vi "Position_TOTAL_R24_cleaned up front.vi"(5 "Distance Between \nCameras  (*unit)":sgl=2.3) -> (12 "dX, dY\nLeft Cam":cluster{"X":sgl[], "Y":sgl[]}={"X"=[-1.0065897, 0.099401906, 1.1628555, 2.2500029, 0.0], "Y"=[10.716516, 10.801518, 10.883252, 10.9668045, 0.0]}, 13 "Position Valid":bool=TRUE, 14 "Left Camera Real Coordinates":cluster{"X":sgl, "Y":sgl}={"X"=10.842023, "Y"=1.3735824}, 16 "dX, dY\nRight Cam":cluster{"X":sgl[], "Y":sgl[]}={"X"=[-2.8840373, -1.7780458, -0.7145921, 0.3725553, -1.8774476], "Y"=[9.387911, 9.472914, 9.554648, 9.638201, -1.3286046]}, 18 "Robot Coordinates":cluster{"X":sgl, "Y":sgl}={"X"=10.17772, "Y"=2.3123062}, 19 "Orietnation\n(current)":sgl=-30.94054 format="%#_13g")   [LabVIEW 2015]
uses:
  <vilib>/Analysis/coordinate.llb/2D Cartesian Coordinate Rotation (Array).vi
  <vilib>/myRIO/Common/Instrument Driver Framework/myRIO v1.0/DIO/vis/myRIO v1.0 Close DIO.vi
  <vilib>/myRIO/Common/Instrument Driver Framework/myRIO v1.0/DIO/vis/myRIO v1.0 Unreserve DIO.vi
  <vilib>/myRIO/Common/Instrument Driver Framework/myRIO v1.0/DIO/vis/myRIO v1.0 Build MUX Configuration DIO.vi
  <vilib>/myRIO/Common/Instrument Driver Framework/myRIO v1.0/Resource Manager/vis/myRIO v1.0 Unreserve Channel List.vi
  <vilib>/myRIO/Common/Instrument Driver Framework/myRIO v1.0/Resource Manager/vis/myRIO v1.0 Create Configuration List.vi
  <vilib>/myRIO/Common/Instrument Driver Framework/myRIO v1.0/Resource Manager/vis/myRIO v1.0 Unreserve Channel.vi
  <vilib>/myRIO/Common/Instrument Driver Framework/myRIO v1.0/Resource Manager/vis/myRIO v1.0 Build Mutex Name.vi
  <vilib>/Instr/_visa.llb/VISA Configure Serial Port (Instr).vi
  <vilib>/myRIO/Common/Instrument Driver Framework/myRIO v1.0/DIO/vis/myRIO v1.0 Shutdown DIO.vi
  <vilib>/Utility/error.llb/Error Cluster From Error Code.vi
  <vilib>/myRIO/Common/Instrument Driver Framework/myRIO v1.0/Resource Manager/vis/myRIO v1.0 Configure IO.vi
  <vilib>/myRIO/Common/Instrument Driver Framework/Utilities/vis/Configuration Manager.vi
  <vilib>/myRIO/Common/Instrument Driver Framework/Utilities/vis/IO Manager.vi
  <vilib>/myRIO/Common/Instrument Driver Framework/myRIO v1.0/myRIO v1.0 Close.vi
  <vilib>/Analysis/NI_AALPro.lvlib
  <vilib>/myRIO/Instrument Drivers/Onboard IO/DIO/DIO.lvlib
panel:
  in  "Tab Control 2":T1(tab)
  out "Beacon Coordinates - Right Image":T2={"Beacon Position - X px"=[88.975365, 121.85722, 157.60713, 192.74931, 229.82234], "Beacon Position - Y px"=[106.21975, 102.49595, 103.61968, 103.22959, 103.920715]}
  out "Beacon Coordinates - Left Image":T2={"Beacon Position - X px"=[96.57839, 127.0317, 159.93825, 190.94315, 221.86247], "Beacon Position - Y px"=[111.67795, 107.306076, 106.92789, 105.73433, 104.09002]}
  in  "Image Width (px)":sgl=320.0
  in  "Image Height (px)":sgl=240.0
  in  "Cam AOV Horizontal (deg)":sgl=58.0
  in  "Cam AOV Vertical (deg)":sgl=45.0
  out "Angle to Pixel Ratios":T3={"Angle to Pixel\nRatio - Horizontal"=0.18125, "Angle to Pixel\nRatio - Vertical"=0.1875} {"Angle to Pixel\nRatio - Vertical" format="%#_13g"; "Angle to Pixel\nRatio - Horizontal" format="%#_13g"}
  in  "Num of Beacons (Total)":i8=5
  out "Left Data\nInput Flag\n- Internal":bool
  out "Right Data\nInput Flag\n- Internal":bool
  out "This Servo \nAngle - Left":sgl=52.96875
  in  "Valid Angles - L":bool[](array[boolean])=[TRUE, TRUE, TRUE, TRUE, TRUE]
  in  "Valid Angles -R":bool[](array[boolean])=[TRUE, TRUE, TRUE, TRUE, TRUE]
  in  "Beacon Angles - L":sgl[](array[numeric])=[64.19745, 58.642975, 52.682835, 47.05908, 41.446476]
  in  "Beacon Angles -R":sgl[](array[numeric])=[71.43643, 65.46979, 58.9926, 52.62266, 45.904842]
  out "This Servo \nAngle - Right":sgl=58.76953
  in  "Position Calc\nReady":bool=TRUE
  out "Array":sgl[](array[numeric])=[9.555056, 8.575206, 8.036942, 7.810829, 6.6351933]
  out "Array 2":sgl[](array[numeric])=[5.5039287, 6.210328, 7.1312, 8.266513, 8.73579]
  out "Array 3":sgl[](array[numeric])=[3.2039287, 3.9103284, 4.8311996, 5.9665127, 6.4357905]
  in  "stop":bool
  in  "Current Servo Position\n- Left":u16
  in  "Current Servo Position\n- Right":u16
  in  "Servo Algorithm\nCycle Time(ms)":i32=25
  in  "Move Servo\nThreshold (deg)":sgl=2.0 format="%#_13g"
  in  "SERVO ENABLE":bool=TRUE
  in  "Max Write\nTx Attempts":u8=3
  in  "Max Read\nTx Attempts":u8=3
  in  "close comms":bool
  in  "Servo Comm\nLoop Time (ms)":i32=20
  out "dT - Comm Loop":u32=21
  in  "Left Servo\nID":string="\u0000"
  in  "Servo Comm\nWait Time - (ms)":i32
  in  "Right Servo\nID":string="\u0001"
  in  "Search Step Size\n(deg)":sgl=15.0 format="%#_13g"
  out "Last Orientation":sgl=-35.285717
  out "Last Position":cluster{"X":sgl, "Y":sgl}={"X"=10.147585, "Y"=2.64441}
  in  "Compliance Slope":u8=128
  in  "Search Step Size":u16=50
  in  "Mounting Offset - Left":sgl=-45.0
  in  "Minimum Delta \nServo Threshold":i16=3
  in  "Maximum Move \nServo Threshold":i16=300
  in  "Wait Tick Threshold":i32=10
  in  "Min Num Frames\nper Search":i32=5
  in  "Middle Beacon\nCoordinates":cluster{"X":sgl, "Y":sgl}={"X"=0.0, "Y"=2.5}
  in  "Max Recovery\nSearch Attempts":u16=3
  in  "Max Recovery Count\n(Recovery Search)":u16=20
  in  "Mounting Offset - Right":sgl=45.0
  in  "Tracking Timeout\nThreshold":i32=10
  in  "Timeout to \nEnable Reactive Predict":u16=5
  out "Beacon Scales - Right":sgl[](array[numeric])=[50.81787, 54.150085, 54.01553, 51.723366, 54.605507]
  out "Beacon Scales - Left":sgl[](array[numeric])=[46.59789, 48.180458, 47.842606, 46.504417, 45.297752]
  in  "Recovery Parallel\nSearch Offset":u16=50
  in  "Max # Pan Moves":u16=20
  in  "Current Angle\n - Right (internal)":sgl=58.76953
  in  "Current Angle\n - Left (internal)":sgl=52.96875
  in  "Servo Goal Position\n - Left":u16=232
  in  "Servo Goal Position\n - Right":u16=563
  out "Move Servo - R":bool
  out "Move Servo - L":bool
  out "Current L (10bit)":u16=232
  out "Servo Moving - L":bool
  out "Servo Moving - R":bool
  out "Current R (10bit)":u16=559
  out "deltaMoveServo\n- L":i16
  out "Move Respond - L":bool
  out "Move Respond - R":bool
  out "deltaMoveServo\n- R":i16
  out "Current Main State - Left":T4(ring)=enum."Tracking"
  in  "Initial Main State - Left":T4(ring)
  in  "Image Lock - Left":bool=TRUE
  in  "Track Angle Valid - Left":bool=TRUE
  out "New Data  Flag\nLeft Servo":bool
  in  "Tracking Angle - Left":sgl=52.933372
  in  "Search Direction - in - L":bool
  out "Frames Processed\nCount - in -L":i32
  out "Recovery Mode Count - in Left":u16
  in  "Image Lock - Right":bool
  out "Recovery Search\nmove Count - in - L":u16
  out "Recovery Search\nAttempt Count - in - L":u16
  out "Current Move Delta - L":u16
  out "Next Main State - Left":T4(ring)=enum."Tracking"
  in  "Recovery Search\nDirection - L":bool=TRUE
  out "Last Track Angle - L":sgl=52.96875
  in  "Initial Main State- Right":T4(ring)
  out "Current Main State - Right":T4(ring)=enum."Tracking"
  in  "Track Angle Valid  - Right":bool
  out "New Data  Flag\nRight Servo":bool
  in  "Tracking Angle - Right":sgl=58.953144
  out "Recovery Search\nAttempt Count - Right":u16
  out "Recovery Search\nmove Count - Right":u16
  out "Frames Processed\nCount - in Right":i32
  out "Recovery Mode Count in Right":i32
  in  "Recovery Search\nDirection - R":bool
  out "Next Main State - Right":T4(ring)=enum."Tracking"
  in  "Search Direction - in - Right":bool=TRUE
  out "Tracking Timeout\nCount - L":i32
  out "Tracking Timeout\nCount - R":i32
  out "Current Tracking State - Left":enum16{"Track", "Reactive Predict", ""}(ring)
  in  "Initial Tracking State - Left":enum16{"Track", "Reactive Predict", ""}(ring)
  out "Next Tracking State - Left":enum16{"Track", "Reactive Predict", ""}(ring)
  in  "Initial Tracking State - Right":enum16{"Track", "Reactive Predict", ""}(ring)
  out "Current Tracking State - Right 2":enum16{"Track", "Reactive Predict", ""}(ring)
  out "Next Tracking State - Right":enum16{"Track", "Reactive Predict", ""}(ring)
  in  "Initial Recovery State - L":enum16{"Generic Sweep", "Recovery Search"}(ring)=enum."Recovery Search"
  in  "Initial Recovery State  - Right":enum16{"Generic Sweep", "Recovery Search"}(ring)=enum."Recovery Search"
  out "Current Recovery State - Right":enum16{"Generic Sweep", "Recovery Search"}(ring)=enum."Recovery Search"
  out "Next Recovery State - Right":enum16{"Generic Sweep", "Recovery Search"}(ring)=enum."Recovery Search"
  out "Next Recovery State - Left":enum16{"Generic Sweep", "Recovery Search"}(ring)=enum."Recovery Search"
  out "Current Recovery State -L":enum16{"Generic Sweep", "Recovery Search"}(ring)=enum."Recovery Search"
  out "Current Move Delta - R":u16
  in  "Real Beacon\n - Coordinates":cluster{"X":dbl[], "Y":dbl[]}={"X"=[0.0, 0.0, 0.0, 0.0, 0.0, 0.0], "Y"=[0.5, 1.5, 2.5, 3.5, 4.5, 0.0]}
  out "LOCAL\nBeacon Coordinates\nRelative to Robot":cluster{"dX_beacon":sgl[], "dY_beacon":sgl[]}={"dX_beacon"=[5.5039287, 6.210328, 7.1312, 8.266513, 8.73579], "dY_beacon"=[9.555056, 8.575206, 8.036942, 7.810829, 6.6351933]}
  out "Local Coordinates - Calculated":cluster{sgl[], sgl[]}(graph)={[5.5039287, 6.210328, 7.1312, 8.266513, 8.73579], [9.555056, 8.575206, 8.036942, 7.810829, 6.6351933]}
  out "Distance to LBF":sgl[](array[numeric])=[0.024284193, 0.015691843, 0.008273765, 0.028971607, 0.03291407]
  out "Right Camera Real Coordinate":cluster{"X":sgl, "Y":sgl}={"X"=9.513418, "Y"=3.25103}
  out "Post Filtering\n- Valid Beacons":bool[](array[boolean])=[TRUE, TRUE, TRUE, TRUE, FALSE]
  in  "Distance\nBetween Beacons":sgl=1.0 format="%#_13g"
  in  "Distance\nBetween Beacons \n- Tolerance":sgl=0.5 format="%#_13g"
  out "All Object Coordinates \n- Local":cluster{"X":sgl[], "Y":sgl[]}={"X"=[2.3, 5.368779, 6.320682, 7.235974, 8.171657, 0.0], "Y"=[0.0, 9.329155, 8.759661, 8.21207, 7.6522775, 0.0]}
  out "Local Coordinates - Normalized":cluster{sgl[], dbl[]}(graph)={[2.3, 5.368779, 6.320682, 7.235974, 8.171657, 0.0], [0.0, 9.329154968261719, 8.759660720825195, 8.21207046508789, 7.65227746963501, 0.0]}
  out "All Object Coordinates \n- Local - Rotated":cluster{"X":sgl[], "Y":sgl[]}={"X"=[1.8774476, -1.0065897, 0.099401906, 1.1628555, 2.2500029, 0.0], "Y"=[1.3286046, 10.716516, 10.801518, 10.883252, 10.9668045, 0.0]}
  out "Local Coordinates - Rotated":cluster{dbl[], dbl[]}(graph)={[1.8774476489648846, -1.0065896210507148, 0.09940190570174412, 1.1628555490135675, 2.250002943734801, 0.0], [1.3286045709883498, 10.716515276262749, 10.801518262128845, 10.883252530212562, 10.966804865321656, 0.0]}
  out "Current Cam State - R":T5(ring)=enum."Normal - 5"
  out "Current Cam State - L":T5(ring)=enum."Normal - 5"
  out "Right_Flag 2":bool
  out "Beacons Found\n- Right (Bool Array)":bool[](array[boolean])=[TRUE, TRUE, TRUE, TRUE, TRUE]
  out "RIGHT Beacon Position - Y px (IN)":sgl[](array[numeric])=[106.21975, 102.49595, 103.61968, 103.22959, 103.920715]
  out "RIGHT Beacon Coord - X px (IN)":sgl[](array[numeric])=[88.975365, 121.85722, 157.60713, 192.74931, 229.82234]
  out "Left_Flag 2":bool
  out "Beacons Found\n- Left (Bool Array) 2":bool[](array[boolean])=[TRUE, TRUE, TRUE, TRUE, TRUE]
  out "LEFT Beacon Coord - X px (IN) 2":sgl[](array[numeric])=[96.57839, 127.0317, 159.93825, 190.94315, 221.86247]
  out "LEFT Beacon Position - Y px (IN) 2":sgl[](array[numeric])=[111.67795, 107.306076, 106.92789, 105.73433, 104.09002]
  in  "Fetch Input\n(mSec)":u32=20 caption="Update Camera Input\n(mSec)"
  in  "Max Std Dev (5)":sgl=0.1 format="%#_13g"
  out "Position \nLock Status":bool=TRUE
  out "Real Position in Course 2":cluster{"X":dbl[], "Y":dbl[]}(graph)={"X"=[10.147584990557128], "Y"=[2.644409845240164]}
  out "Robot Coordinates - Avgd":cluster{"X":sgl, "Y":sgl}={"X"=10.147585, "Y"=2.64441}
  in  "Max Std Dev (4)":sgl=0.1 format="%#_13g"
  in  "Max Std Dev (3)":sgl=0.2 format="%#_13g"
  in  "New Position\nWeight (X coord)":sgl=0.8 format="%#_13g"
  in  "Max X (arena)":sgl=35.0
  in  "Max Y (arena)":sgl=15.0
  in  "History Size":u8=15
  out "Orientation Avgd":sgl=-35.285717
  in  "New Position \nThreshold":sgl=2.0
  out "Robot Coordinates\nHistory":cluster{sgl, sgl}[](array[cluster])=[{10.147585, 2.64441}, {10.056327, 2.8351064}, {10.020484, 2.7815769}, {10.034186, 2.7172103}, {0.0, 0.0}, {10.036168, 2.7859242}, {9.938812, 2.8961887}, {10.1160965, 2.6632404}, {10.016709, 2.7454932}, {10.037537, 2.8544023}, {10.017025, 2.7817721}, {9.997087, 2.8064857}, {10.065648, 2.6537364}, {10.084976, 2.6750228}, {10.082739, 2.688601}]
  out "Orientation\nHistory":sgl[](array[numeric])=[-35.285717, -36.86449, -36.153664, -35.44657, 0.0, -37.6105, -36.02637, -35.82032, -36.08894, -37.01076, -36.293255, -36.40525, -35.738438, -35.683483, -35.770218]
  out "Position Valid\nHistory":bool[](array[boolean])=[TRUE, TRUE, TRUE, TRUE, FALSE, TRUE, TRUE, TRUE, TRUE, TRUE, TRUE, TRUE, TRUE, TRUE, TRUE]
  in  "Moving Average\nWindow Length":u8=10
  in  "New Orientation \nThreshold":sgl=20.0
  in  "Triangle Based\nWeight":sgl format="%#_13g"
  out "Scale Based\nWeight":sgl=1.0 format="%#_13g"
  in  "New Position\nWeight (Y coord)":sgl=0.3 format="%#_13g"
  in  "New Orientation\nWeight":sgl=0.2
  out "dT":dbl=144.111
  in  "Position Calc\nTimer":u32=100 caption="Position Calc Timer"
  out "dA2 3":sgl=44.126 format="%#_13g"
  in  "Distance Threshold\nRef Triangles (*unit)":sgl=30.0
  out "Valid Beacon Sets_":bool[](array[boolean])=[TRUE, TRUE, TRUE, TRUE, TRUE]
  in  "Check Shared Var Timer":u32=50 caption="Main Loop\n Timer (ms)"
  out "dA2 2":sgl=48.543114 format="%#_13g"
  out "dA2 4":sgl=48.543114 format="%#_13g"
  out "Last Track Angle - R":sgl=59.941406
  in  "Recovery Search\nDirection - L 2":bool
  in  "Max Recovery Count\n(Recovery Search) 2":u16
  in  "Max Recovery\nSearch Attempts 2":u16
  in  "Image Lock - Right 2":bool
  # "SETTINGS"
  # "IMAGE TO ANGLE VARIABLES"
  # "INPUTS"
  # "OUTPUT VALUES"
  # "CONFIG"
  # "SERVO CONTROL VARIABLES"
  # "SERVO CONTROL VARIABLES"
  # "CONFIG"
  # "SHARED VARIABLE INPUTS"
  # "LOCAL VARIABLE INPUTS"
  # "INTERNRAL VARIABLES"
  # "MISC"
  # "SERVO IDs"
  # "CONTROL DELAYS"
  # "COMM LOOP DELAY"
  # "COMM PROTOCOL"
  # "Make function of distance^^"
  # "LEFT SERVO"
  # "RIGHT SERVO"
  # "Main State Machine"
  # "Recovery State Machine"
  # "Current Track Angle Inputs"
  # "Servo Status Inputs"
  # "Main State Machine Inputs"
  # "Recovery State Machine Inputs"
  # "Current Track Angle Inputs"
  # "Servo Status Inputs"
  # "Tracking State Machine Inputs"
  # "Tracking State Machine Inputs"
  # "POSITION CALCULATION VARIABLES"
  # "OUTPUT VALUES"
  # "CONFIG VALUES"
  # "FILTER CONFIG VALUES"
  # "FEEDBACK INPUT VALUES"
  # "INPUT VALUES"
  # "INTERMEDIATE VALUES"
  # "Use moving average for previous orientation thresholds"
  # "*********************"
  # "unfiltered"
  # "Inter Beacon Distance Filtering"
  # "NOTE: Must be 1 bigger than amount of beacons"
  # "NOTE: Must be 1 bigger than amount of beacons"
  # "VISION PROCESSEING INPUTS"
  # "update to coordinate outlier filtering R2"
  # "NEW FILTER VALS"
  # "MOVING AVERAGE\nVARIABLES"
  # "DISTANCE SOURCE WEIGHT"
  # "*****  I made this 0\n         bc it seems to be \n        more stable"
  # "**** only left side starts search\nat previously known good angle"
  # "Recovery State Machine Feedback"
  # "SEARCH ROUTINE VARIABLES"
types:
  T1 = enum32{"image to angle ", "servo control 2", "servo control", "left and right servo", "left and right servo 2", "left and right servo 3", "left and right servo 4", "left and right servo 5", "left and right servo 6"}
  T2 = cluster{"Beacon Position - X px":sgl[], "Beacon Position - Y px":sgl[]}
  T3 = cluster{"Angle to Pixel\nRatio - Horizontal":sgl, "Angle to Pixel\nRatio - Vertical":sgl}
  T4 = enum16{"Start Up Search", "Tracking", "Recovery Mode", ""}
  T5 = enum16{"Sub - 2", "Sub - 3", "Sub - 4", "Normal - 5"}
  T6 = cluster{"Tracking Coordinates":cluster{"X":dbl, "Y":dbl}, "Current Valid":bool, "Current State - Out":enum16{"Sub - 2", "Sub - 3", "Sub - 4", "Normal - 5"}, "Setting Values":cluster{"Min Scale":dbl, "Max Scale":dbl, "Min Score":dbl}}
  T7 = cluster{"Array of Double":dbl[], "Array of Double":dbl[]}
  T8 = typedef "DIO.lvlib/DIO Reference.ctl" = cluster{"myRIO Reference":T9, "DIO Channels List":T13}
  T9 = typedef "myRIO Generic Hardware Reference.ctl" = cluster{"myRIO Model":T10, "myRIO Hardware Reference":T11}
  T10 = typedef "Hardware Version Enum.ctl" = enum16{"Unknown", "myRIO-1900", "myRIO-1950", "roboRIO"}
  T11 = typedef "myRIO v1.0 Reference.ctl" = cluster{"Generic FPGA Reference":T12, "Allow multiple opens":bool}
  T12 = typedef "Generic FPGA Reference.ctl" = refnum<k20>
  T13 = typedef "DIO Channels List.ctl" = T14[]
  T14 = typedef "DIO Channels Enum.ctl" = enum16{"Not Connected", "C/DIO0", "C/DIO1", "C/DIO2", "C/DIO3", "C/DIO4", "C/DIO5", "C/DIO6", "C/DIO7", "A/DIO0", "A/DIO1", "A/DIO2", "A/DIO3", "A/DIO4", "A/DIO5", "A/DIO6", "A/DIO7", "A/DIO8", "A/DIO9", "A/DIO10", "A/DIO11", "A/DIO12", "A/DIO13", "A/DIO14", "A/DIO15", "B/DIO0", "B/DIO1", "B/DIO2", "B/DIO3", "B/DIO4", "B/DIO5", "B/DIO6", "B/DIO7", "B/DIO8", "B/DIO9", "B/DIO10", "B/DIO11", "B/DIO12", "B/DIO13", "B/DIO14", "B/DIO15", "LED0", "LED1", "LED2", "LED3", "Button0", "DIO/DIO0", "DIO/DIO1", "DIO/DIO2", "DIO/DIO3", "DIO/DIO4", "DIO/DIO5", "DIO/DIO6", "DIO/DIO7", "DIO/DIO8", "DIO/DIO9", "SPI/CS0", "SPI/CS1", "SPI/CS2", "SPI/CS3", "LED RADIO (Green)", "LED RADIO (Red)", "LED COMM (Green)", "LED COMM (Red)", "LED MODE (Green)", "LED MODE (Red)"}
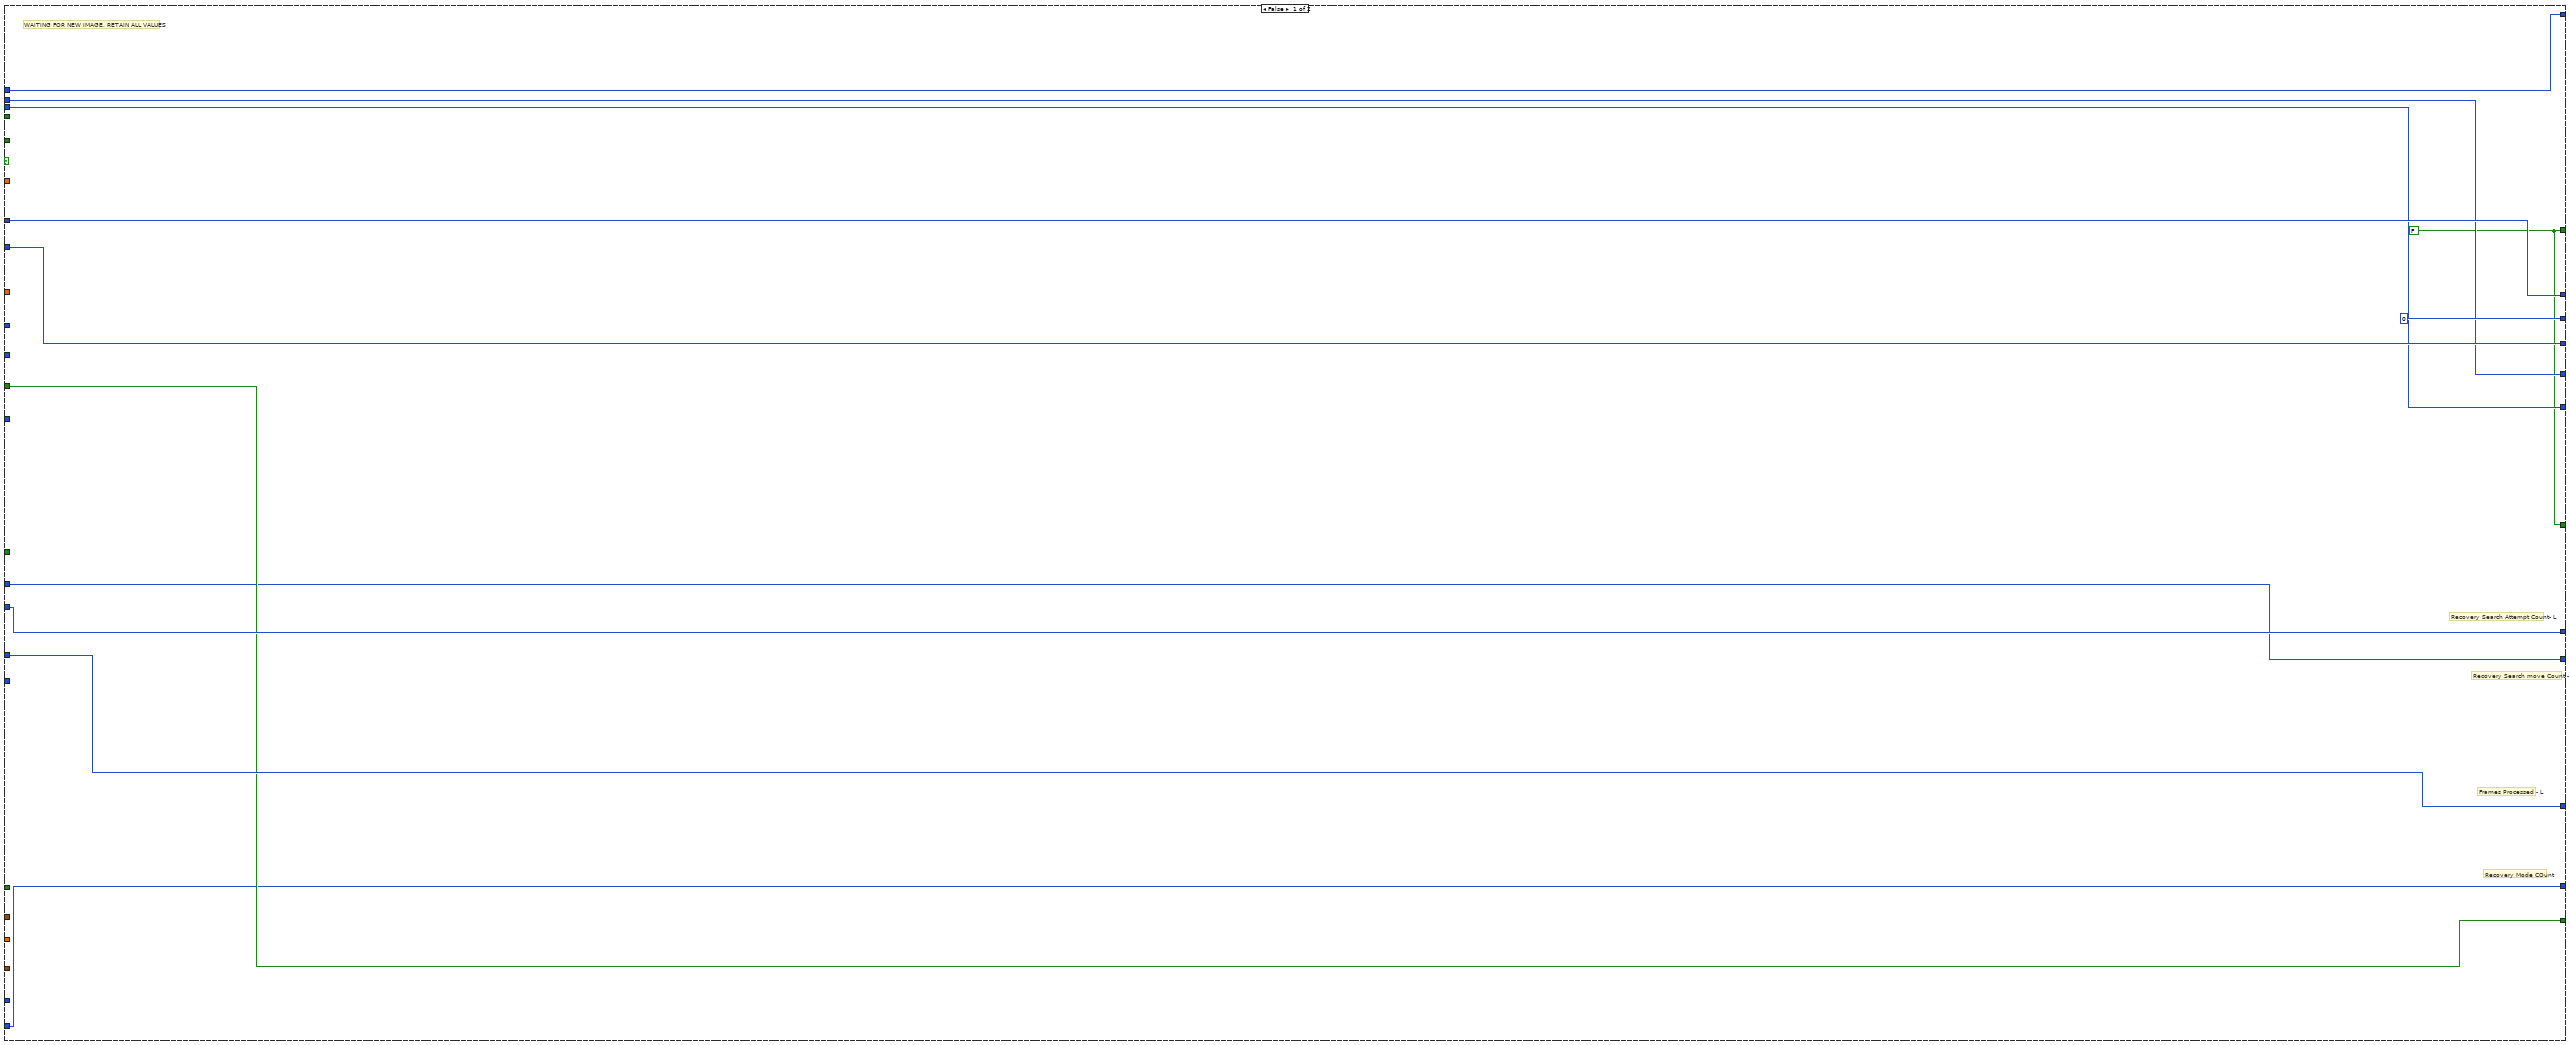
[diagram p2: hidden frame]
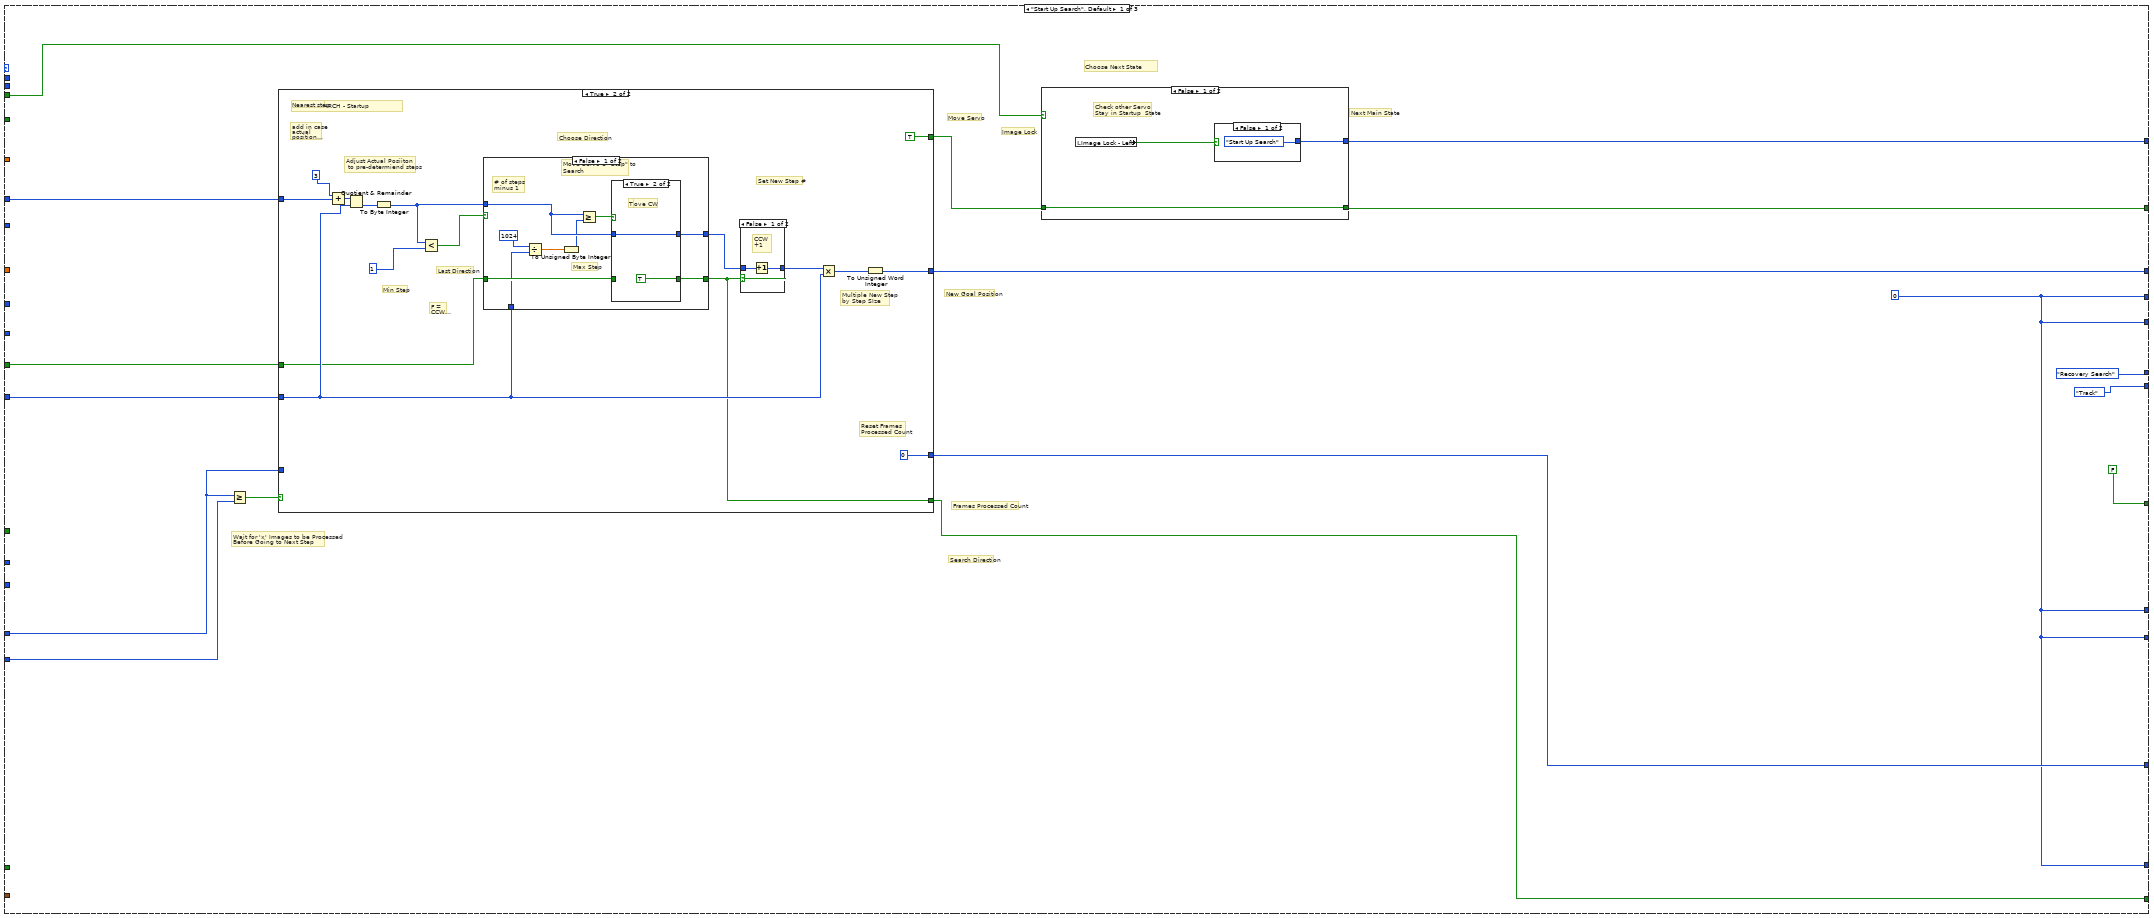
[diagram p3: hidden frame]
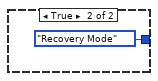
[diagram p4: hidden frame]
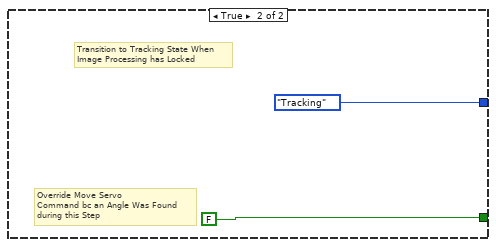
[diagram p5: hidden frame]
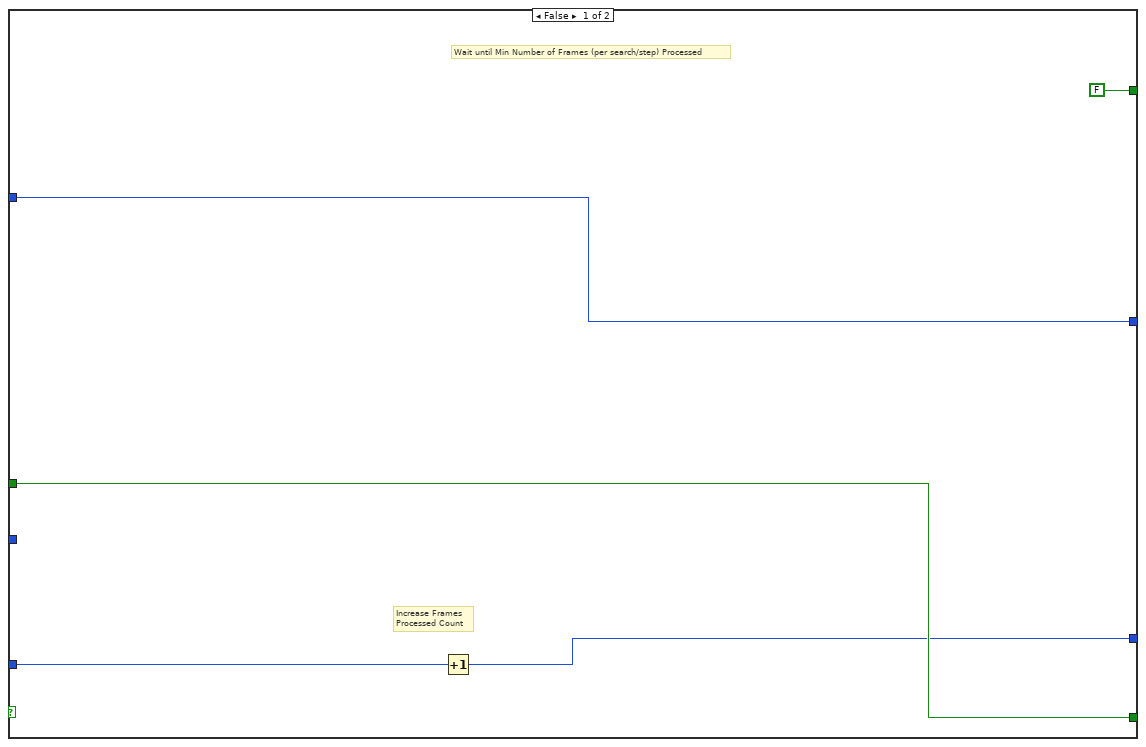
[diagram p6: hidden frame]
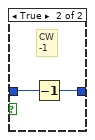
[diagram p7: hidden frame]
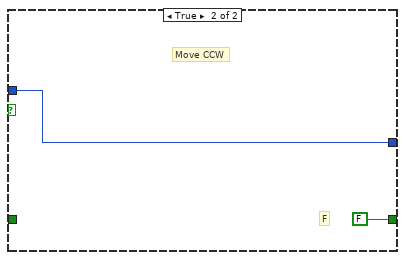
[diagram p9: hidden frame]
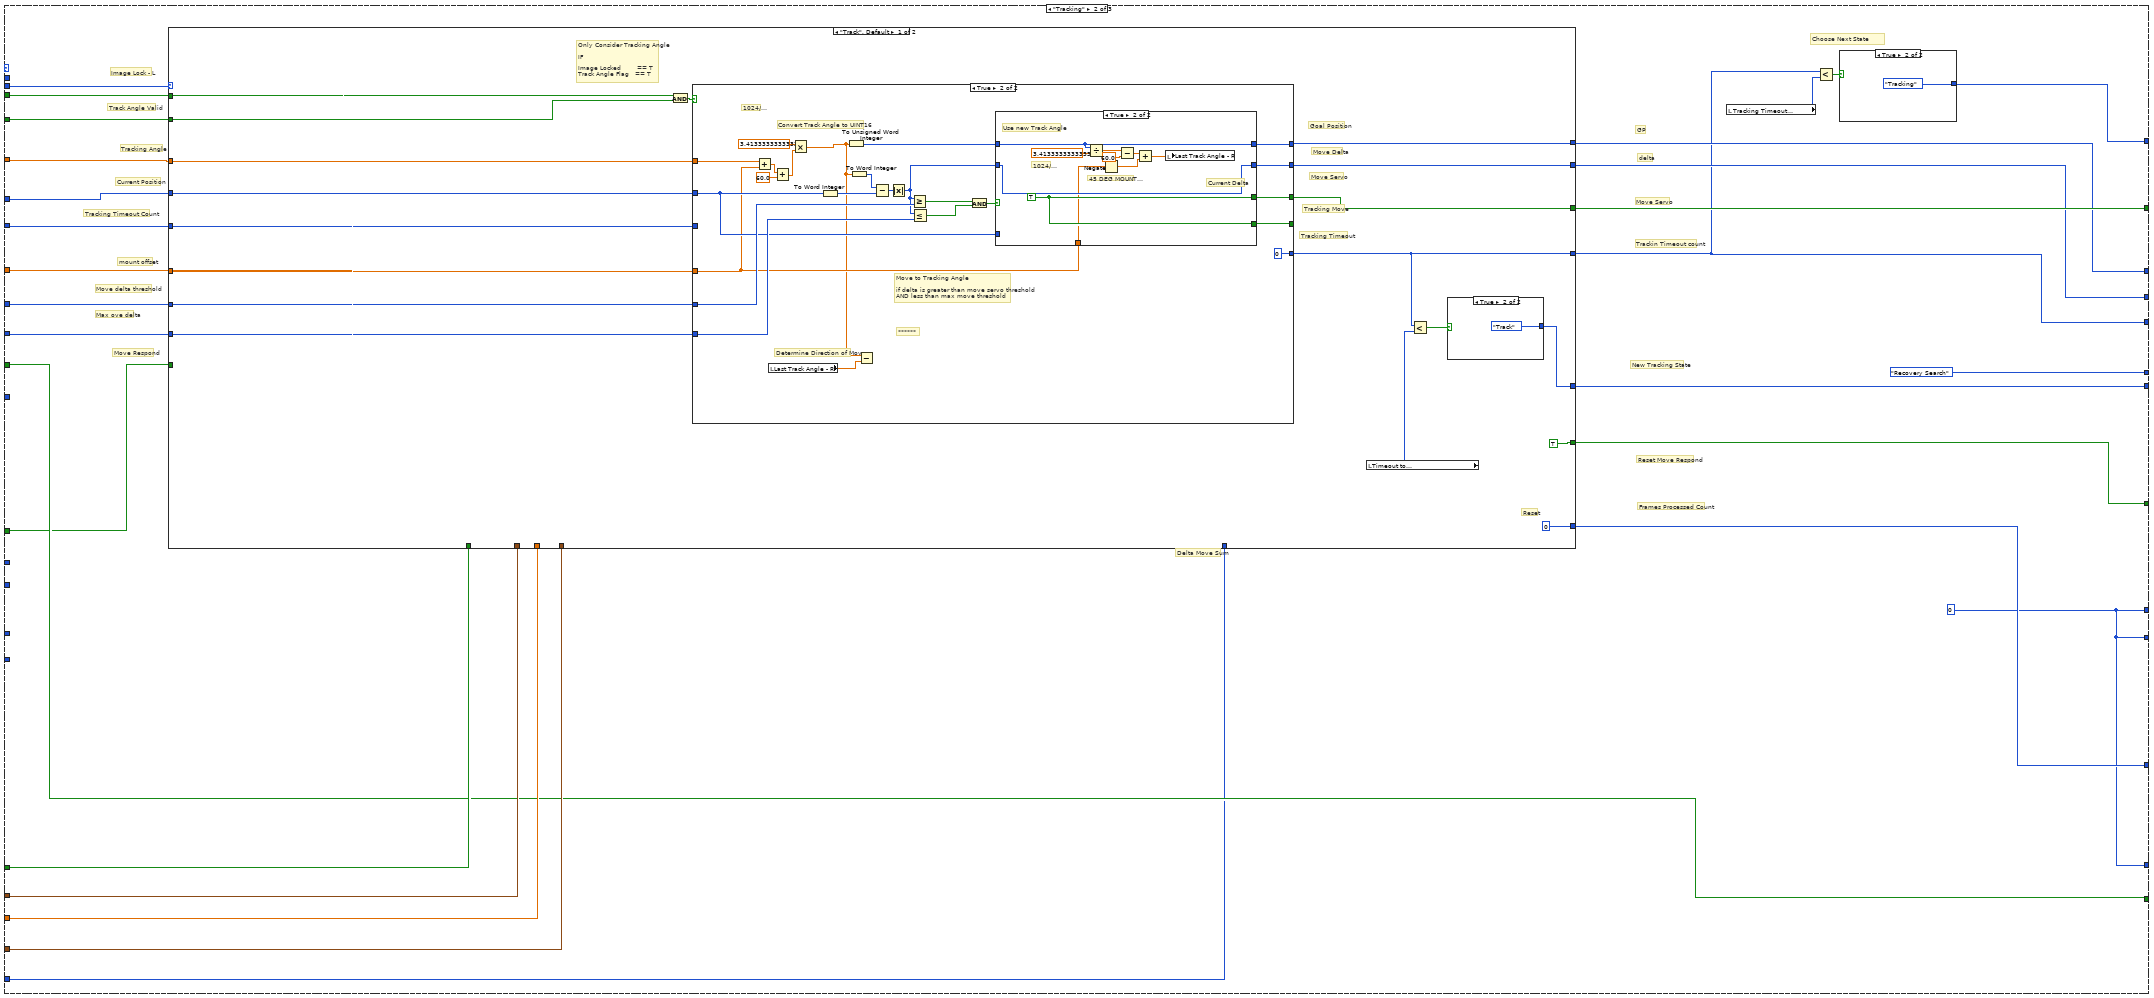
[diagram p10: hidden frame]
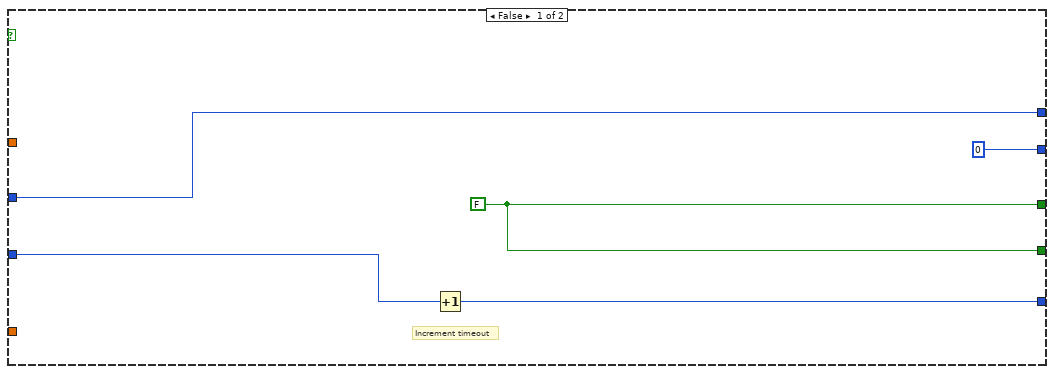
[diagram p11: hidden frame]
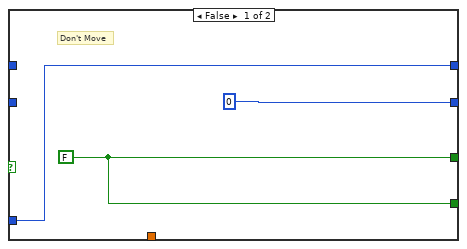
[diagram p12: hidden frame]
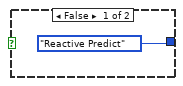
[diagram p13: hidden frame]
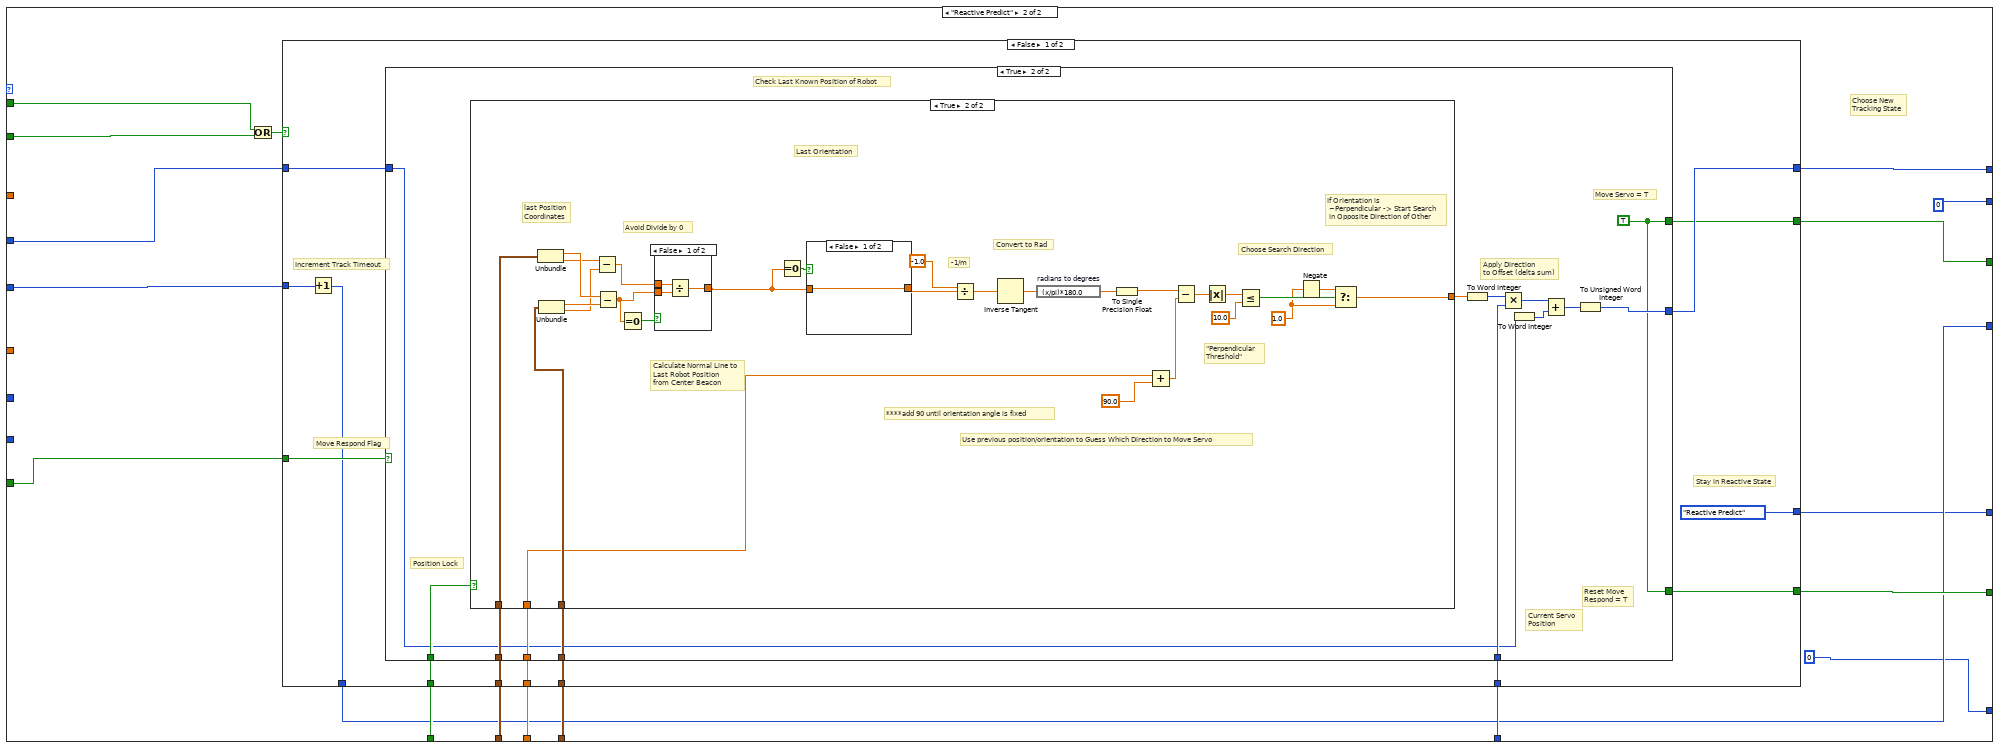
[diagram p14: hidden frame]
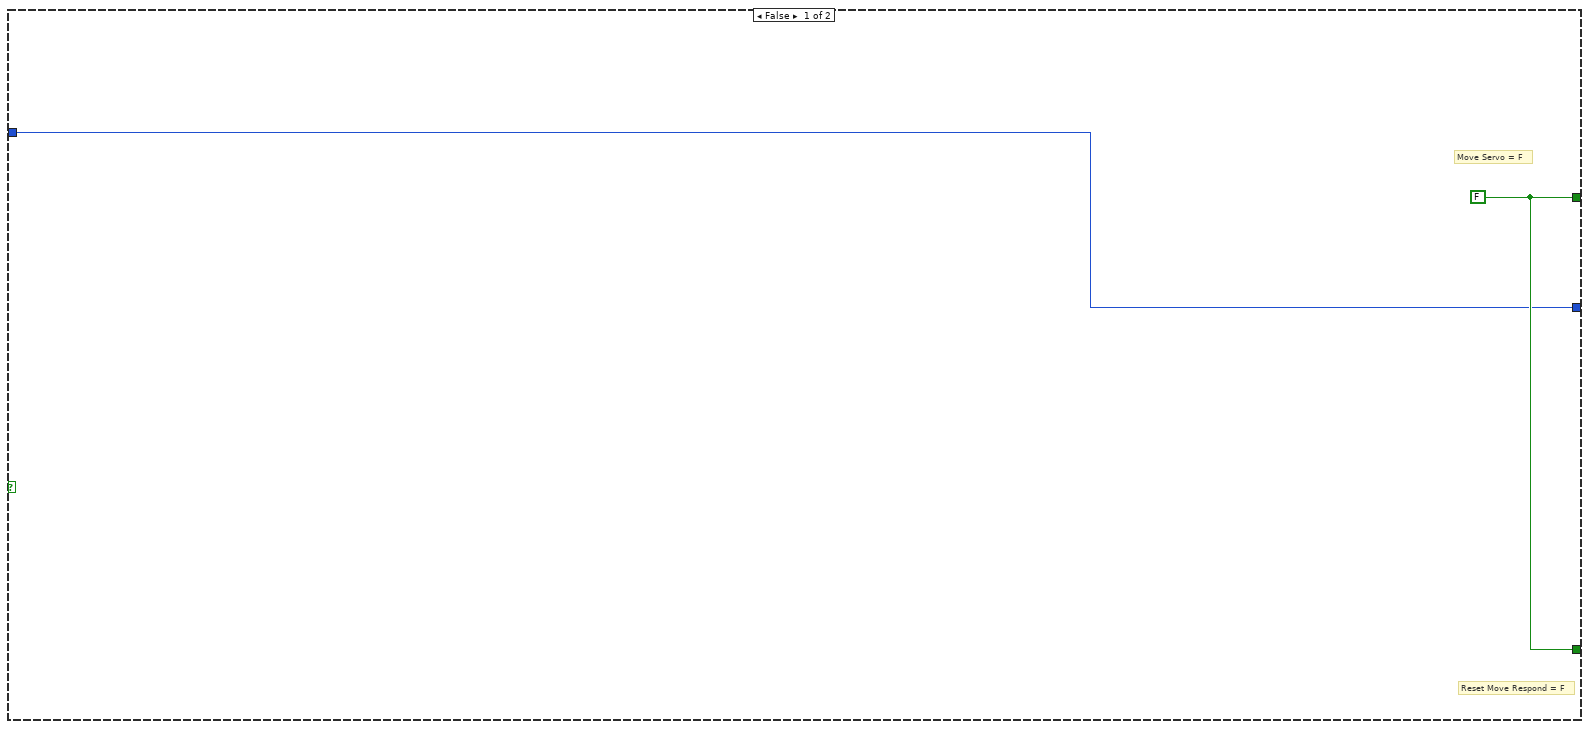
[diagram p15: hidden frame]
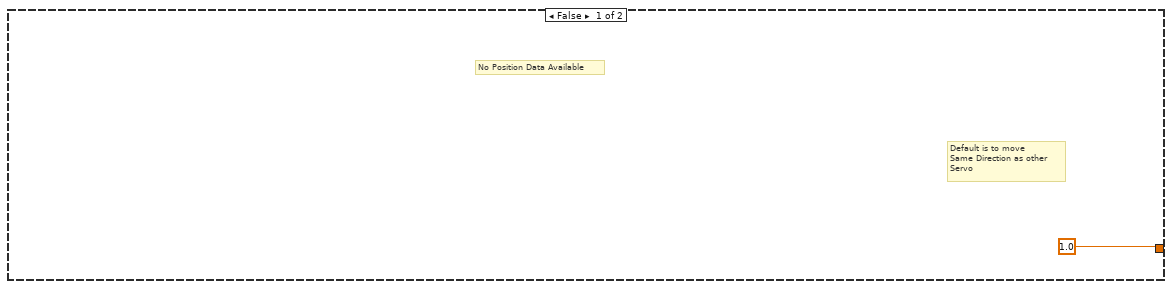
[diagram p16: hidden frame]
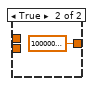
[diagram p17: hidden frame]
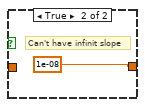
[diagram p18: hidden frame]
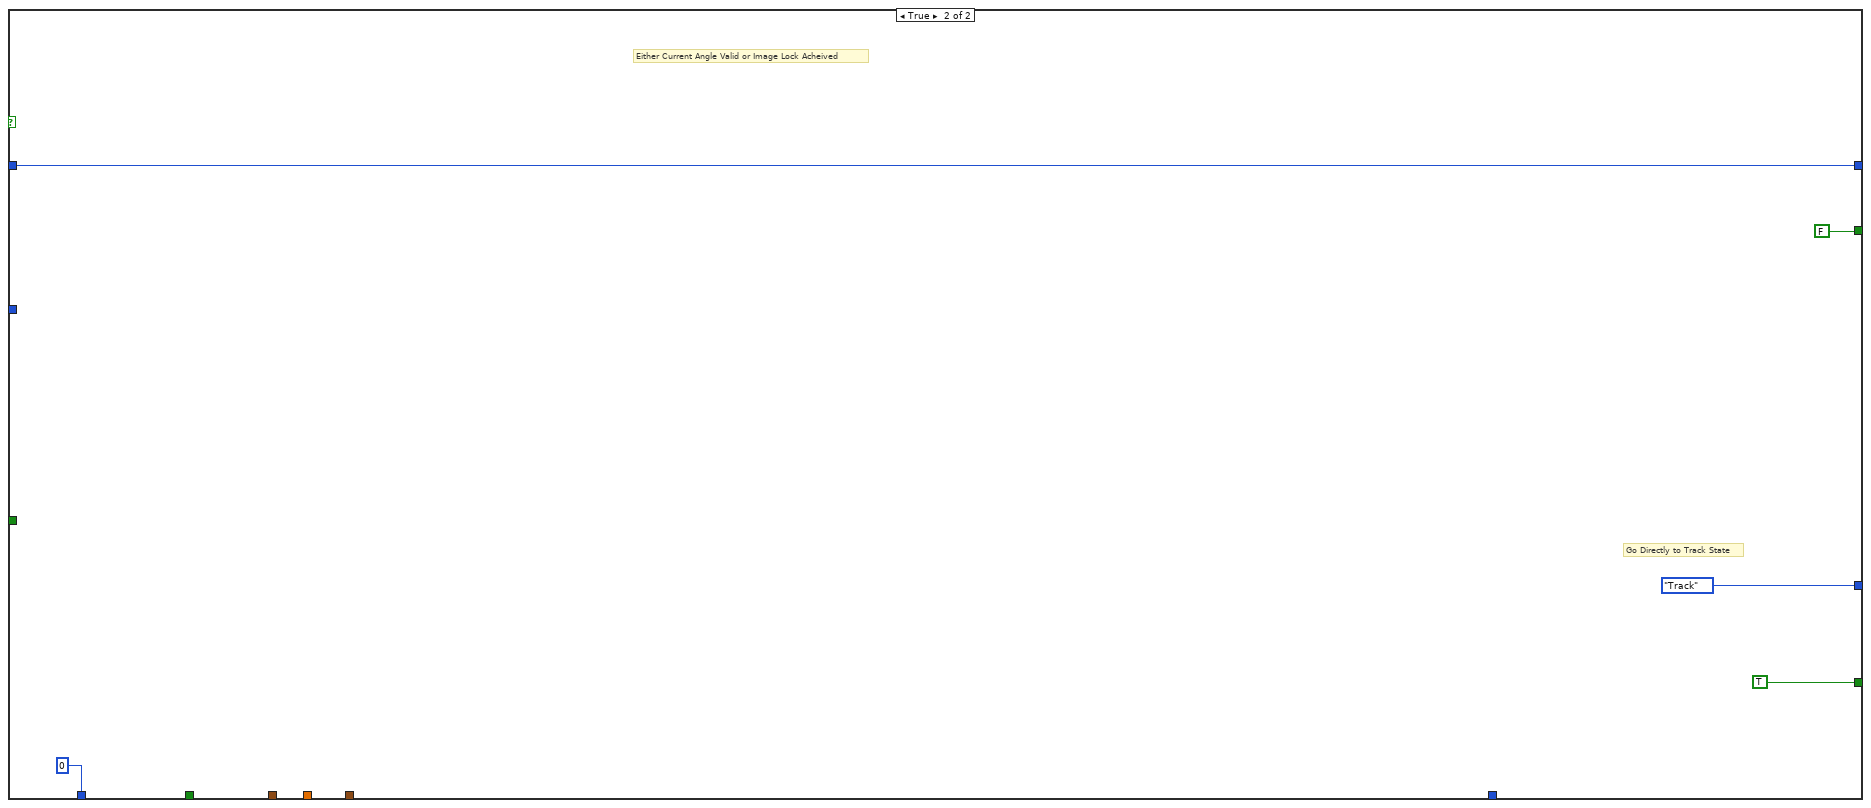
[diagram p19: hidden frame]
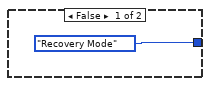
[diagram p20: hidden frame]
diagram:
  (unwired) enum16{"Generic Sweep", "Recovery Search"}."Recovery Search"
  w12 = 0 ("Frames Processed\nCount - in")
  w13 = 0 ("Frames Processed\nCount - in")
  w2 = FALSE
  w34 = sgl 0.0
  # "SERVO CONTROL FLAGS"
  # "***"
  # "Next Tracking State"
  # "Tracking Timeout Count"
  # "Search Direction - L"
  # "Next Recovery State"
  # "Move Respond"
  # "Recovery Mode Count - L"
  # "Delta Move Sum - L"
  # "Wait Tick Count - L"
  # "Frames Processed - L"
  # "Recovery Search move Count - L"
  # "Recovery Search Attempt Count- L"
  # "Next Main State"
  # "Search Direction - L"
  # "Next Recovery State"
  # "INPUTS - Local vars"
  # "Recovery Mode Count - L"
  # "Delta Move Sum - L"
  # "Frames Processed\nLeft"
  # "Move Respond - R"
  # "Initial Search Direction\n- Right"
  # "Move Respond"
  # "Recovery Mode Count - L"
  # "Delta Move Sum - L"
  # "Wait Tick Count - L"
  # "Frames Processed - L"
  # "Recovery Search move Count - L"
  # "Recovery Search Attempt Count- L"
  # "Next Main State"
  # "Settings -- Update in a slow loop"
  # "Recovery Mode Count - L"
  # "Delta Move Sum - L"
  # "Frames Processed\nLeft"
  # "Move Respond - L"
  # "Replace these with\nconstants"
  # "Initial Search Direction\n- Left"
  # "Read Inputs when Available"
  # "# of Physical Beacons"
  # "Right Data Internal Falg"
  # "Left Data Internal Falg"
  # "Initialize Shift Arrays"
  # "Robot Position (cluster)\nShift Array"
  # "Robot Position (cluster)\nShift Array"
  # "Position Valid Shift Array"
  # "Orientation Shift Array"
  # "Position Valid Shift Array"
  # "Orientation Shift Array"
  # "Servo Communication (to Servo- UART))"
  # "Internal Local Variables"
  # "Servo Control Logic"
  # "Local Variables"
  # "Images to Robot Position Calculation Process"
  # "SERVO MOTOR CONTROL"
  # "SERVO MOTOR CONTROL"
  n1 = Divide(x="Cam AOV Horizontal (deg)", y="Image Width (px)") -> (x/y=w25:sgl)
  n2 = Divide(x="Cam AOV Vertical (deg)", y="Image Height (px)") -> (x/y=w26:sgl)
  n3 = Bundle(w25, w26) -> (w20:cluster{sgl, sgl})  [unwired: 1 in]
  "Angle to Pixel Ratios" <- w20
  n4 = disable-structure shown="Disabled" {
    frame Disabled {
      # "Always Read Incoming Flags & Store"
      n5 = while {
        tunnel: "Check Shared Var Timer" -> [w46]
        stop <- FALSE stop-if-true
        n6 = shared-variable "myRIO-1900\\Lib1.lvlib\\RIGHT_FLAG"() -> (→"Right_Flag 2":bool)  [unwired: 1 in, 1 out]
        n7 = shared-variable "myRIO-1900\\Lib1.lvlib\\Left_Flag"() -> (→"Left_Flag 2":bool)  [unwired: 1 in, 1 out]
        n8 = call "Wait8"("Count(mSec)"=w46) -> ()  [unwired: 1 out]
      }
    }
    frame Enabled {
    }
  }
  n9 = while {
    shift-right: [w55] -> _
    shift-left: w2 -> [w60]
    shift-right: [w54] -> _
    shift-left: w2 -> [w58]
    tunnel: w20 -> [w56]
    tunnel: "Num of Beacons (Total)" -> [w57]
    stop <- FALSE stop-if-true
    # "Wait for Both Internal Flags"
    n10 = call "Wait6"("Count(mSec)"="Fetch Input\n(mSec)") -> ()  [unwired: 1 out]
    n11 = shared-variable "RT myRIO Target - Overlord\\Localization_Variables_r0.lvlib\\RIGHT_FLAG"() -> (w51:bool)  [unwired: 1 in, 1 out]
    n12 = shared-variable "RT myRIO Target - Overlord\\Localization_Variables_r0.lvlib\\Left_Flag"() -> (w52:bool)  [unwired: 1 in, 1 out]
    n13 = case shown="True" w51 {
      tunnel: w57 -> [_ w79]
      tunnel: w56 -> [_ w77]
      tunnel: [w61 w67] -> w49
      tunnel: w58 -> [w61 _]
      frame False {
        # "Don't Update Servo Position\nbc we're waiting on new Data to\ncome in and the servo position\nwas set at the previous set of data"
      }
      frame True {
        w67 = TRUE
        # "Store Values"
        # "Raise Internal Flag"
        # "If New Data Available"
        # "From Shift Reg"
        # "Perforrm Indivudual Angle Calculation"
        # "Pull Down Individual Flag"
        n14 = shared-variable "RT myRIO Target - Overlord\\Localization_Variables_r0.lvlib\\RIGHT_BEACON_X_array"() -> (w73:dbl[])  [unwired: 1 in, 1 out]
        "RIGHT Beacon Coord - X px (IN)" <- w73
        n15 = shared-variable "RT myRIO Target - Overlord\\Localization_Variables_r0.lvlib\\Image Lock - R"() -> (w68:bool)  [unwired: 1 in, 1 out]
        n16 = shared-variable "RT myRIO Target - Overlord\\Localization_Variables_r0.lvlib\\RIGHT_BEACON_Scales"() -> (→"Beacon Scales - Right":sgl[])  [unwired: 1 in, 1 out]
        n17 = shared-variable "RT myRIO Target - Overlord\\Localization_Variables_r0.lvlib\\Info - Right"() -> (w65:T6)  [unwired: 1 in, 1 out]
        n18 = shared-variable "RT myRIO Target - Overlord\\Localization_Variables_r0.lvlib\\RIGHT_BEACON_Y_array"() -> (w72:dbl[])  [unwired: 1 in, 1 out]
        "RIGHT Beacon Position - Y px (IN)" <- w72
        n19 = shared-variable "RT myRIO Target - Overlord\\Localization_Variables_r0.lvlib\\RIGHT_BEACON_BOOL_array"() -> (w71:bool[])  [unwired: 1 in, 1 out]
        "Beacons Found\n- Right (Bool Array)" <- w71
        n20 = Unbundle By Name(w65) -> ("Tracking Coordinates"=w64:cluster{"X":dbl, "Y":dbl}, "Current Valid"=w63:bool, "Current State - Out"=→"Current Cam State - R":T5)
        n21 = local write "Image Lock - Right"(w68) -> ()
        n22 = Bundle("Array of Double"=w73, "Array of Double"=w72) -> (w70:T7)  [unwired: 1 in]
        "Beacon Coordinates - Right Image" <- w70
        n23 = shared-variable "RT myRIO Target - Overlord\\Localization_Variables_r0.lvlib\\Right Servo Angle_Image"() -> (w69:dbl)  [unwired: 1 in, 1 out]
        "This Servo \nAngle - Right" <- w69
        n24 = shared-variable "RT myRIO Target - Overlord\\Localization_Variables_r0.lvlib\\RIGHT_FLAG"(FALSE) -> ()  [unwired: 1 in, 1 out]
        n25 = feedback #1() -> (w81:sgl[])  [unwired: 1 in]
        n26 = feedback #2() -> (w80:bool[])  [unwired: 1 in]
        n27 = call "Angle Calc_Individual Process R4.vi"("Angle to Pixel Ratios"=w77, "Previous Angles"=w81, "Num of Beacons"=w79, "Beacon Coordinates - Image"=w70, "Current Servo Angle"=w69, "Beacons Found (Bool Array)"=w71, "Previous Valid Angles"=w80, "Tracking Coordinates"=w64) -> ("Servo Goal Angle"=w76:sgl, "Valid Beacons (Bool Array)\nPosition Calc"=w75:bool[], "Angle Of Beacons \nRelative to Robot"=w74:sgl[])  [unwired: 4 in, 1 out]
        n28 = feedback-in #1(w74) -> ()
        n29 = feedback-in #2(w75) -> ()
        n30 = local write "Beacon Angles -R"(w74) -> ()
        n31 = local write "Tracking Angle - Right"(w76) -> ()
        n32 = local write "Valid Angles -R"(w75) -> ()
        n33 = local write "Track Angle Valid  - Right"(w63) -> ()
        n34 = local write "New Data  Flag\nRight Servo"(w67) -> ()
      }
    }
    "Right Data\nInput Flag\n- Internal" <- w49
    n35 = case shown="True" w52 {
      tunnel: [w82 w88] -> w48
      tunnel: w60 -> [w82 _]
      tunnel: w56 -> [_ w92]
      tunnel: w57 -> [_ w91]
      frame False {
        # "Don't Update Servo Position\nbc we're waiting on new Data to\ncome in and the servo position\nwas set at the previous set of data"
      }
      frame True {
        w88 = TRUE
        # "Store Values"
        # "Raise Internal Flag"
        # "If New Data Available"
        # "Perforrm Indivudual Angle Calculation"
        # "Pull Down Individual Flag"
        n36 = shared-variable ".\\Localization_Variables_r0.lvlib\\LEFT_BEACON_X_array"() -> (w98:dbl[])  [unwired: 1 in, 1 out]
        "LEFT Beacon Coord - X px (IN) 2" <- w98
        n37 = shared-variable "RT myRIO Target - Overlord\\Localization_Variables_r0.lvlib\\LEFT_BEACON_Scales"() -> (→"Beacon Scales - Left":sgl[])  [unwired: 1 in, 1 out]
        n38 = shared-variable "RT myRIO Target - Overlord\\Localization_Variables_r0.lvlib\\LEFT_BEACON_Y_array"() -> (w99:dbl[])  [unwired: 1 in, 1 out]
        "LEFT Beacon Position - Y px (IN) 2" <- w99
        n39 = shared-variable "RT myRIO Target - Overlord\\Localization_Variables_r0.lvlib\\LEFT_BEACON_BOOL_array"() -> (w100:bool[])  [unwired: 1 in, 1 out]
        "Beacons Found\n- Left (Bool Array) 2" <- w100
        n40 = shared-variable "RT myRIO Target - Overlord\\Localization_Variables_r0.lvlib\\Image Lock - L"() -> (w89:bool)  [unwired: 1 in, 1 out]
        n41 = shared-variable "RT myRIO Target - Overlord\\Localization_Variables_r0.lvlib\\Info - Left"() -> (w86:T6)  [unwired: 1 in, 1 out]
        n42 = Unbundle By Name(w86) -> ("Tracking Coordinates"=w85:cluster{"X":dbl, "Y":dbl}, "Current Valid"=w84:bool, "Current State - Out"=→"Current Cam State - L":T5)
        n43 = local write "Image Lock - Left"(w89) -> ()
        n44 = Bundle("Array of Double"=w98, "Array of Double"=w99) -> (w96:T7)  [unwired: 1 in]
        "Beacon Coordinates - Left Image" <- w96
        n45 = shared-variable "RT myRIO Target - Overlord\\Localization_Variables_r0.lvlib\\Left Servo Angle_Image"() -> (w90:dbl)  [unwired: 1 in, 1 out]
        "This Servo \nAngle - Left" <- w90
        n46 = shared-variable "RT myRIO Target - Overlord\\Localization_Variables_r0.lvlib\\Left_Flag"(FALSE) -> ()  [unwired: 1 in, 1 out]
        n47 = feedback #3() -> (w102:sgl[])  [unwired: 1 in]
        n48 = feedback #4() -> (w101:bool[])  [unwired: 1 in]
        n49 = call "Angle Calc_Individual Process R4.vi"("Angle to Pixel Ratios"=w92, "Previous Angles"=w102, "Num of Beacons"=w91, "Beacon Coordinates - Image"=w96, "Current Servo Angle"=w90, "Beacons Found (Bool Array)"=w100, "Previous Valid Angles"=w101, "Tracking Coordinates"=w85) -> ("Servo Goal Angle"=w95:sgl, "Valid Beacons (Bool Array)\nPosition Calc"=w94:bool[], "Angle Of Beacons \nRelative to Robot"=w93:sgl[])  [unwired: 4 in, 1 out]
        n50 = feedback-in #3(w93) -> ()
        n51 = feedback-in #4(w94) -> ()
        n52 = local write "Beacon Angles - L"(w93) -> ()
        n53 = local write "Valid Angles - L"(w94) -> ()
        n54 = local write "Tracking Angle - Left"(w95) -> ()
        n55 = local write "Track Angle Valid - Left"(w84) -> ()
        n56 = local write "New Data  Flag\nLeft Servo"(w88) -> ()
      }
    }
    "Left Data\nInput Flag\n- Internal" <- w48
    n57 = And(x=w48, y=w49) -> (x .and. y?=w59:bool)
    n58 = case shown="True" w59 {
      selector: w59 -> [_ w105]
      tunnel: w48 -> [w104 _]
      tunnel: [w104 w106] -> w55
      tunnel: [w103 w106] -> w54
      tunnel: w49 -> [w103 _]
      frame False {
      }
      frame True {
        w106 = FALSE
        # "Reset Internal Data Flags"
        # "Position Data\nReady Enabled"
        n59 = local write "Position Calc\nReady"(w105) -> ()
      }
    }
  }
  n60 = Bundle(w34, w34) -> (w37:cluster{sgl, sgl})  [unwired: 1 in]
  n61 = Initialize Array(w34, "History Size") -> (w32:sgl[])
  n62 = Initialize Array(w37, "History Size") -> (w33:cluster{sgl, sgl}[])
  n63 = Initialize Array(FALSE, "History Size") -> (w31:bool[])
  n64 = call "Tick Count4"() -> ("Tick Count(uSec)"=w30:u32)
  n65 = while {
    shift-right: [w117] -> _
    shift-left: w32 -> [w114]
    shift-right: [w116] -> _
    shift-left: w31 -> [w115]
    shift-right: [w118] -> _
    shift-left: w33 -> [w109]
    shift-right: [w110] -> _
    shift-left: w30 -> [w111]
    stop <- "stop" stop-if-true
    n66 = call "Wait5"("Count(mSec)"="Position Calc\nTimer") -> ()  [unwired: 1 out]
    n67 = case shown="True" "Position Calc\nReady" {
      selector: "Position Calc\nReady" -> [_ w188]
      tunnel: w109 -> [_ w209]
      tunnel: w109 -> [w127 w203]
      tunnel: w114 -> [w129 w202]
      tunnel: w115 -> [w128 w201]
      tunnel: [w129 w208] -> w117
      tunnel: [w128 w206] -> w116
      tunnel: [w127 w207] -> w118
      tunnel: w115 -> [_ w200]
      tunnel: w114 -> [_ w199]
      tunnel: [w126 w195] -> w112
      tunnel: w111 -> [_ w195]
      tunnel: [FALSE TRUE] -> w113
      tunnel: w109 -> [_ w190]
      frame False {
        n68 = call "Tick Count5"() -> ("Tick Count(uSec)"=w126:u32)
      }
      frame True {
        # "dY"
        # "dX"
        # "Valid"
        # "Find Local Coordinates"
        # "Valid COunt"
        # "Make sure 2+ Data Sets are Still available"
        # "Check 1st element\nwith rest of elements"
        # "Make Sure all Pointed \nIn Same Direction"
        # "For Each Valid Beacon\nCalculate Distance from Each Camera to Each Beacon"
        # "Find Common Beacons\nAmong Cameras"
        # "Currently will only\ncalculate position if 2+ \nbeacons are available \nfrom both cameras"
        # "System is in Normal (long range) State"
        # "Average Both Data Sets"
        # "Estimate Distance for each Available Beacon Angle\nPER Camera, indivduallly"
        # "At least 2+ Avaialbe"
        # "CALCULATE AVERAGE ORIENTATION"
        # "Update Outputs\nif Current Calc is Invalid\n(shouldn't matter)"
        # "Estimate Orienation Based on Previous Position"
        # "****# of previous in history that must be true\nin order for position to be considered \"locked\""
        # "New Position is Valid if both \nOrientation and Positions\nis within range of previous"
        # "Robot Position\n Shift Array"
        # "Position Valid Shift Array"
        # "Orientation Shift Array"
        # "Orientation Value"
        # "Shift & Insert Current Position Valid"
        # "Position Valid\n(orientation)"
        # "Position Valid\n(position)"
        # "Update Shift Registers"
        # "Shift & Insert Current Calculated Orientation"
        # "Shift & Insert Current Robot Position"
        # "UPDATE FINAL OUTPUT\n VALUES"
        n69 = local read "Num of Beacons (Total)"() -> (w171:i8)
        n70 = Not(x=w188) -> (.not. x?=w189:bool)
        n71 = local write "Position Calc\nReady"(w189) -> ()
        n72 = disable-structure shown="Disabled" {
          frame Disabled {
            w210 = T5."Normal - 5" ("Initial State")
            # "***********do for both"
            # "sTATE"
            n73 = local read "Current Cam State - L"() -> (w214:T5)
            n74 = local read "Current Cam State - R"() -> (w213:T5)
            n75 = Equal?(x=w214, y=w210) -> (x = y?=w212:bool)
            n76 = Equal?(x=w213, y=w210) -> (x = y?=w211:bool)
            n77 = And(x=w212, y=w211) -> ()  [unwired: 1 out]
          }
          frame Enabled {
          }
        }
        n78 = local read "Beacon Scales - Left"() -> (w177:sgl[])
        n79 = local read "Beacon Scales - Right"() -> (w174:sgl[])
        n80 = for {
          N: w171 -> [_]
          tunnel: "Valid Angles - L" -> [w346] mode=indexing
          tunnel: "Beacon Angles - L" -> [w353] mode=indexing
          tunnel: w177 -> [w354] mode=indexing
          tunnel: "Valid Angles -R" -> [w339] mode=indexing
          tunnel: "Beacon Angles -R" -> [w352] mode=indexing
          tunnel: w174 -> [w351] mode=indexing
          tunnel: "Distance Between \nCameras  (*unit)" -> [w350]
          tunnel: [w345] -> w168 mode=indexing
          tunnel: [w344] -> w167 mode=indexing
          tunnel: [w343] -> w169 mode=indexing
          tunnel: [w342] -> w133 mode=indexing
          tunnel: [w341] -> w132 mode=indexing
          tunnel: [w340] -> w131 mode=indexing
          # "dY"
          # "dX"
          # "Valid"
          # "If Both Cameras are using Same Beacon Data,\nAverage the 2 independently esitmated positions"
          # "dY"
          # "dX"
          # "dY"
          # "dX"
          n81 = case shown="True" w346 {
            tunnel: w353 -> [_ w431]
            tunnel: [w418 w422] -> w348
            tunnel: [w418 w423] -> w347
            tunnel: w354 -> [_ w419]
            frame False {
              w418 = sgl 0.0
              # "Current Data Set Was Not Valid\nFill with 0\nWill not be used later"
            }
            frame True {
              # "Estimate Distance"
              # "Negate dX if A2>90"
              # "Find LOCAL Coordinate of Each Beacon"
              # "Current - Valid Data Set"
              n82 = call "Scaling and Mapping"("Signals"=w419) -> ("Scaled Signals"=w420:dynamicdata)  [unwired: 9 in, 1 out]
              n83 = To Single Precision Float(number=w420) -> (single precision float=w421:sgl)
              n84 = Less?(x=w431, y=sgl 90.0) -> (x < y?=w433:bool)
              n85 = case shown="False" w433 {
                tunnel: w431 -> [w440 w442]
                tunnel: [w438 w443] -> w430
                tunnel: [FALSE TRUE] -> w425
                frame False {
                  # "Negative Y"
                  # "A2 is > 90"
                  n86 = Subtract(x=w440, y=sgl 90.0) -> (x-y=w438:sgl)
                }
                frame True {
                  # "Positive Y"
                  # "A2 is < 90"
                  n87 = Subtract(x=sgl 90.0, y=w442) -> (x-y=w443:sgl)
                }
              }
              "dA2 2" <- w430
              n88 = expression code="(x/180.0)*pi" "degrees to radians"(w430) -> (w428:sgl)
              n89 = expression code="(x/180.0)*pi" "degrees to radians"(w430) -> (w429:sgl)
              n90 = Cosine(x=w428) -> (cos(x)=w426:sgl)
              n91 = Sine(x=w429) -> (sin(x)=w427:sgl)
              n92 = Multiply(x=w421, y=w426) -> (x*y=w423:sgl)
              n93 = Multiply(x=w421, y=w427) -> (x*y=w424:sgl)
              n94 = case shown="True" w425 {
                tunnel: w424 -> [w435 w436]
                tunnel: [w434 w436] -> w422
                frame False {
                  n95 = Negate(x=w435) -> (-x=w434:sgl)
                }
                frame True {
                }
              }
            }
          }
          n96 = case shown="True" w339 {
            tunnel: w352 -> [_ w404]
            tunnel: [w389 w394] -> w341
            tunnel: [w389 w393] -> w342
            tunnel: w351 -> [_ w391]
            tunnel: w350 -> [_ w395]
            tunnel: [w389 w392] -> w340
            frame False {
              w389 = sgl 0.0
              # "Current Data Set Was Not Valid\nFill with 0\nWill not be used later"
            }
            frame True {
              # "Add delta for\nRIGHT camera ONLY"
              # "Estimate Distance"
              # "Negate dX if A2>90"
              # "Find LOCAL Coordinate of Each Beacon"
              # "Current - Valid Data Set"
              n97 = call "Scaling and Mapping3"("Signals"=w391) -> ("Scaled Signals"=w390:dynamicdata)  [unwired: 9 in, 1 out]
              n98 = To Single Precision Float(number=w390) -> (single precision float=w396:sgl)
              n99 = Less?(x=w404, y=sgl 90.0) -> (x < y?=w406:bool)
              n100 = case shown="False" w406 {
                tunnel: w404 -> [w413 w415]
                tunnel: [w411 w416] -> w403
                tunnel: [FALSE TRUE] -> w398
                frame False {
                  # "Negative Y"
                  # "A2 is > 90"
                  n101 = Subtract(x=w413, y=sgl 90.0) -> (x-y=w411:sgl)
                }
                frame True {
                  # "Positive Y"
                  # "A2 is < 90"
                  n102 = Subtract(x=sgl 90.0, y=w415) -> (x-y=w416:sgl)
                }
              }
              "dA2 3" <- w403
              n103 = expression code="(x/180.0)*pi" "degrees to radians"(w403) -> (w401:sgl)
              n104 = expression code="(x/180.0)*pi" "degrees to radians"(w403) -> (w402:sgl)
              n105 = Cosine(x=w401) -> (cos(x)=w399:sgl)
              n106 = Sine(x=w402) -> (sin(x)=w400:sgl)
              n107 = Multiply(x=w396, y=w399) -> (x*y=w393:sgl)
              n108 = Multiply(x=w396, y=w400) -> (x*y=w397:sgl)
              n109 = case shown="True" w398 {
                tunnel: w397 -> [w408 w409]
                tunnel: [w407 w409] -> w392
                frame False {
                  n110 = Negate(x=w408) -> (-x=w407:sgl)
                }
                frame True {
                }
              }
              n111 = Add(x=w395, y=w392) -> (x+y=w394:sgl)
            }
          }
          n112 = And(x=w346, y=w339) -> (x .and. y?=w349:bool)
          n113 = case shown="False" w349 {
            tunnel: w348 -> [w362 w388]
            tunnel: w347 -> [w359 w387]
            tunnel: w341 -> [w361 w386]
            tunnel: w342 -> [w360 w385]
            tunnel: [w357 w381] -> w345
            tunnel: [w356 w380] -> w344
            tunnel: w346 -> [w358 _]
            tunnel: w339 -> [w363 _]
            tunnel: [w355 TRUE] -> w343
            frame False {
              n114 = Exclusive Or(1:w363, 2:w358) -> (0:w364:bool)
              n115 = case shown="True" w364 {
                tunnel: w362 -> [_ w372]
                tunnel: w361 -> [_ w369]
                tunnel: w360 -> [_ w368]
                tunnel: w359 -> [_ w370]
                tunnel: w358 -> [_ w374]
                tunnel: [w365 w373] -> w357
                tunnel: [w365 w371] -> w356
                tunnel: [FALSE TRUE] -> w355
                frame False {
                  w365 = sgl 0.0
                  # "None are valid,"
                }
                frame True {
                  # "Only 1 beacon is valid,\nUse the valid beacon"
                  n116 = case shown="False" w374 {
                    tunnel: [w376 w378] -> w373
                    tunnel: w372 -> [_ w378]
                    tunnel: [w375 w377] -> w371
                    tunnel: w370 -> [_ w377]
                    tunnel: w369 -> [w376 _]
                    tunnel: w368 -> [w375 _]
                    frame False {
                      # "Left is invalid,\nRight MUST be valid"
                    }
                    frame True {
                      # "Left is Valid"
                    }
                  }
                }
              }
            }
            frame True {
              w382 = sgl 2.0 ("y")
              # "Both are Valid"
              n117 = Add(x=w388, y=w386) -> (x+y=w383:sgl)
              n118 = Add(x=w387, y=w385) -> (x+y=w384:sgl)
              n119 = Divide(x=w384, y=w382) -> (x/y=w380:sgl)
              n120 = Divide(x=w383, y=w382) -> (x/y=w381:sgl)
            }
          }
        }
        "Array" <- w133
        "Array 2" <- w132
        "Array 3" <- w131
        n121 = And(x="Valid Angles - L", y="Valid Angles -R") -> (x .and. y?=w159:bool[])
        n122 = Boolean To (0,1)(Boolean=w159) -> (0, 1=w156:i16[])
        n123 = Add Array Elements(numeric array=w156) -> (sum=w157:i16)
        n124 = Greater?(x=w157, y=1) -> (0:w155:bool)
        n125 = for {
          N: w171 -> [_]
          tunnel: w155 -> [w275]
          tunnel: "Beacon Angles - L" -> [w274] mode=indexing
          tunnel: "Beacon Angles -R" -> [w273] mode=indexing
          tunnel: "Distance Between \nCameras  (*unit)" -> [w272]
          tunnel: "Distance Threshold\nRef Triangles (*unit)" -> [w271]
          tunnel: [w270] -> w142 mode=indexing
          tunnel: [w269] -> _ mode=indexing
          tunnel: [w268] -> w141 mode=indexing
          tunnel: [w267] -> _ mode=indexing
          tunnel: [w266] -> w143 mode=indexing
          tunnel: [w265] -> w149 mode=indexing
          n126 = case shown="True" w275 {
            tunnel: w274 -> [w280 w290]
            tunnel: w273 -> [w279 w289]
            tunnel: w272 -> [_ w281]
            tunnel: w271 -> [_ w282]
            tunnel: [w280 w288] -> w270
            tunnel: [w279 w287] -> w269
            tunnel: [FALSE w286] -> w268
            tunnel: [w277 w285] -> w267
            tunnel: [w277 w284] -> w266
            tunnel: [0 w283] -> w265
            frame False {
              w277 = sgl 1.0
            }
            frame True {
              # "Build Reference Triangle"
              n127 = call "Position Calc_Build Reference Triangle_R1.vi"("A2_in"=w290, "A3_in"=w289, "S1 (Length Between\n Cameras - inches)"=w281, "Distance\nThreshold"=w282) -> ("S2"=w285:sgl, "S3"=w284:sgl, "Direction"=w283:i8, "A2"=w288:sgl, "A3"=w287:sgl, "Accept"=w286:bool)  [unwired: 6 in]
            }
          }
        }
        n128 = for {
          N: w171 -> [_]
          tunnel: w141 -> [w260] mode=indexing
          tunnel: w149 -> [w264] mode=indexing
          tunnel: [w264] -> w151 mode=indexing if=w260
          shift-right: [w263] -> w145
          shift-left: 0 -> [w261]
          # "Only add to array\nif valid distance"
          n129 = Increment(x=w261) -> (x+1=w262:i32)
          n130 = Select(t=w262, s=w260, f=w261) -> (s? t:f=w263:i32)
        }
        n131 = Index Array(array=w151, index=0) -> (element=w152:i32)
        n132 = Equal?(x=w151, y=w152) -> (x = y?=w153:bool[])
        n133 = And Array Elements(Boolean array=w153) -> (logical AND=w147:bool)
        n134 = Greater?(x=w145, y=1) -> (0:w146:bool)
        n135 = And(x=w147, y=w146) -> (x .and. y?=w140:bool)
        n136 = case shown="True" w140 {
          tunnel: w171 -> [w217 w226]
          tunnel: w143 -> [_ w225]
          tunnel: w142 -> [_ w224]
          tunnel: w141 -> [_ w223]
          tunnel: [w216 w222] -> w170
          tunnel: [w215 w221] -> w166
          tunnel: [w215 w220] -> w165
          frame False {
            # "Build Array for False"
            n137 = for {
              N: w217 -> [_]
              tunnel: [sgl 0.0] -> w215 mode=indexing
              tunnel: [FALSE] -> w216 mode=indexing
            }
          }
          frame True {
            n138 = for {
              N: w226 -> [_]
              tunnel: w224 -> [w232] mode=indexing
              tunnel: w225 -> [w231] mode=indexing
              tunnel: [w230] -> w221 mode=indexing
              tunnel: [w229] -> w220 mode=indexing
              tunnel: [w228] -> w222 mode=indexing
              tunnel: w223 -> [w227] mode=indexing
              n139 = case shown="True" w227 {
                selector: w227 -> [w234 w238]
                tunnel: w232 -> [_ w246]
                tunnel: [w233 w236] -> w230
                tunnel: [w233 w237] -> w229
                tunnel: w231 -> [_ w235]
                tunnel: [w234 w238] -> w228
                frame False {
                  w233 = sgl 0.0
                  # "Current Data Set Was Not Valid\nFill with 0\nWill not be used later"
                }
                frame True {
                  # "dY"
                  # "dX"
                  # "Negate dX if A2>90"
                  # "Find LOCAL Coordinate of Each Beacon"
                  # "Current - Valid Data Set"
                  n140 = Less?(x=w246, y=sgl 90.0) -> (x < y?=w248:bool)
                  n141 = case shown="False" w248 {
                    tunnel: w246 -> [w255 w257]
                    tunnel: [w253 w258] -> w245
                    tunnel: [FALSE TRUE] -> w240
                    frame False {
                      # "Negative Y"
                      # "A2 is > 90"
                      n142 = Subtract(x=w255, y=sgl 90.0) -> (x-y=w253:sgl)
                    }
                    frame True {
                      # "Positive Y"
                      # "A2 is < 90"
                      n143 = Subtract(x=sgl 90.0, y=w257) -> (x-y=w258:sgl)
                    }
                  }
                  "dA2 4" <- w245
                  n144 = expression code="(x/180.0)*pi" "degrees to radians"(w245) -> (w243:sgl)
                  n145 = expression code="(x/180.0)*pi" "degrees to radians"(w245) -> (w244:sgl)
                  n146 = Cosine(x=w243) -> (cos(x)=w241:sgl)
                  n147 = Sine(x=w244) -> (sin(x)=w242:sgl)
                  n148 = Multiply(x=w235, y=w241) -> (x*y=w237:sgl)
                  n149 = Multiply(x=w235, y=w242) -> (x*y=w239:sgl)
                  n150 = case shown="True" w240 {
                    tunnel: w239 -> [w250 w251]
                    tunnel: [w249 w251] -> w236
                    frame False {
                      n151 = Negate(x=w250) -> (-x=w249:sgl)
                    }
                    frame True {
                    }
                  }
                }
              }
            }
          }
        }
        n152 = Subtract(x=sgl 1.0, y="Triangle Based\nWeight") -> (x-y=w162:sgl)
        "Scale Based\nWeight" <- w162
        n153 = for {
          N: w171 -> [_]
          tunnel: w170 -> [w295] mode=indexing
          tunnel: w169 -> [w294] mode=indexing
          tunnel: w168 -> [w299] mode=indexing
          tunnel: w167 -> [w298] mode=indexing
          tunnel: w166 -> [w301] mode=indexing
          tunnel: w165 -> [w300] mode=indexing
          tunnel: "Triangle Based\nWeight" -> [w297]
          tunnel: w162 -> [w296]
          tunnel: [w293] -> w139 mode=indexing
          tunnel: [w292] -> w161 mode=indexing
          tunnel: [w291] -> w160 mode=indexing
          # "If Beacon info \nis available from\nboth"
          n154 = And(x=w295, y=w294) -> (x .and. y?=w302:bool)
          n155 = case shown="True" w302 {
            selector: w302 -> [_ w328]
            tunnel: w301 -> [w309 w336]
            tunnel: w300 -> [w307 w337]
            tunnel: w299 -> [w305 w335]
            tunnel: w298 -> [w304 w334]
            tunnel: w297 -> [_ w338]
            tunnel: w296 -> [_ w333]
            tunnel: [w308 w326] -> w291
            tunnel: [w310 w327] -> w292
            tunnel: w295 -> [w311 _]
            tunnel: w294 -> [w306 _]
            tunnel: [w303 w328] -> w293
            frame False {
              n156 = case shown="False" w311 {
                selector: w311 -> [_ w323]
                tunnel: [w316 w325] -> w310
                tunnel: w309 -> [_ w325]
                tunnel: [w314 w324] -> w308
                tunnel: w307 -> [_ w324]
                tunnel: w306 -> [w317 _]
                tunnel: w305 -> [w315 _]
                tunnel: w304 -> [w313 _]
                tunnel: [w312 w323] -> w303
                frame False {
                  n157 = case shown="False" w317 {
                    selector: w317 -> [w318 w320]
                    tunnel: [w319 w322] -> w316
                    tunnel: w315 -> [_ w322]
                    tunnel: [w319 w321] -> w314
                    tunnel: w313 -> [_ w321]
                    tunnel: [w318 w320] -> w312
                    frame False {
                      w319 = sgl 0.0
                      # "None avail"
                    }
                    frame True {
                    }
                  }
                }
                frame True {
                }
              }
            }
            frame True {
              n158 = Multiply(x=w336, y=w338) -> (x*y=w332:sgl)
              n159 = Multiply(x=w337, y=w338) -> (x*y=w330:sgl)
              n160 = Multiply(x=w335, y=w333) -> (x*y=w331:sgl)
              n161 = Multiply(x=w334, y=w333) -> (x*y=w329:sgl)
              n162 = Add(x=w332, y=w331) -> (x+y=w327:sgl)
              n163 = Add(x=w330, y=w329) -> (x+y=w326:sgl)
            }
          }
        }
        "Valid Beacon Sets_" <- w139
        n164 = Boolean To (0,1)(Boolean=w139) -> (0, 1=w182:i16[])
        n165 = Add Array Elements(numeric array=w182) -> (sum=w181:i16)
        n166 = Greater?(x=w181, y=i16 1) -> (0:w179:bool)
        n167 = case shown="True" w179 {
          tunnel: w209 -> [_ w535]
          tunnel: [0.0 ("f") w534] -> w205
          tunnel: [w447 w533] -> w204
          tunnel: w200 -> [_ w452]
          tunnel: w199 -> [_ w532]
          tunnel: [FALSE w531] -> w193
          tunnel: [FALSE w530] -> w192
          tunnel: w190 -> [_ w529]
          tunnel: [sgl 0.0 w527] -> w183
          tunnel: "Distance Between \nCameras  (*unit)" -> [_ w464]
          tunnel: w161 -> [_ w463]
          tunnel: w160 -> [_ w462]
          tunnel: w139 -> [_ w461]
          tunnel: w171 -> [_ w460]
          frame False {
            w446 = 0.0 ("f")
            n168 = Bundle("f"=w446, "f"=w446) -> (w447:cluster{"f":dbl, "f":dbl})  [unwired: 1 in]
          }
          frame True {
            w499 = sgl 2.0
            w516 = 0
            # "Current Orientaiton"
            # "Valid Position Ccount\n(within moving avg\nwinfow)"
            # "Valid Position Ccount"
            # "Only Apply This Filtering \nif 3 or More Beacons Still Valid"
            # "Orientation Value"
            # "Orientation Valid"
            # "Y (current)"
            # "X (current)"
            # "Number of Valid\nPrevious Orientations"
            # "More than 1 Previous\nValid Positions"
            # "More than\n2previous position\navailable"
            # "Choose Beacon Set\nwith Lowest Std Dev"
            # "Y value cannot be negative"
            # "Find New # Of Valid Beacons"
            # "Adjust/Normalize\nLocal Beacon Positions\nusing Line of Best fit"
            # "# Valid\nData Sets"
            # "cam, y"
            # "cam, x"
            # "Calculate dX and dY\nfor right cam"
            # "Average dX and dY from each (valid) beacon to find position of each camera\n\nthen average all  positions for each camera find center between"
            # "Convert Slope\nto Radians"
            # "*rotate CCW in rad"
            # "Rotate Coordinate\n System by Slope"
            n169 = Boolean To (0,1)(Boolean=w452) -> (0, 1=w483:i16[])
            n170 = Initialize Array(u8 0, "Moving Average\nWindow Length") -> (w457:u8[])
            n171 = Add Array Elements(numeric array=w483) -> (sum=w451:i16)
            n172 = Greater?(x=w451, y=0) -> (0:w454:bool)
            n173 = while {
              shift-right: [w537] -> w455
              shift-left: w457 -> [w539]
              tunnel: w452 -> [w544] mode=indexing
              shift-right: [w543] -> w453
              shift-left: u8 0 -> [w545]
              tunnel: "Moving Average\nWindow Length" -> [w536]
              i -> [w538]
              stop <- w540 stop-if-true
              # "Grab Last 2 Valid Position Indexes"
              n174 = case shown="True" w544 {
                tunnel: w545 -> [w547 w549]
                tunnel: [w547 w552] -> w543
                tunnel: w539 -> [w546 w551]
                tunnel: w538 -> [_ w550]
                tunnel: [w546 w548] -> w537
                frame False {
                }
                frame True {
                  # "Update Index\nto use"
                  # "Increment\nValid Count"
                  n175 = Replace Array Subset(array=w551, new element=w550, index=w549) -> (w548:u8[])
                  n176 = Increment(x=w549) -> (x+1=w552:u8)
                }
              }
              n177 = Greater Or Equal?(x=w543, y=w536) -> (x >= y?=w542:bool)
              n178 = Greater Or Equal?(x=w538, y=w536) -> (x >= y?=w541:bool)
              n179 = Or(x=w542, y=w541) -> (x .or. y?=w540:bool)
            }
            n180 = Bundle(w463, w462) -> (→"LOCAL\nBeacon Coordinates\nRelative to Robot" →"Local Coordinates - Calculated":cluster{sgl[], sgl[]})  [unwired: 1 in]
            n181 = call "Coordinate_Outlier_Filtering_R2.vi"("Num of Beacons"=w460, "Max Std Dev(all 5)"="Max Std Dev (5)", "X in"=w463, "Valid Data\nSets in"=w461, "Y in"=w462, "Max Std Dev( 4 )"="Max Std Dev (4)", "Max Std Dev (3)"="Max Std Dev (3)") -> ("Y out"=w474:sgl[], "X out"=w475:sgl[], "Valid Beacons\nout"=w472:bool[], "Slope out"=w480:dbl)  [unwired: 3 in, 2 out]
            n182 = Inverse Tangent(1:w480) -> (0:w495:dbl)
            n183 = expression code="(x/pi)*180.0" "radians to degrees"(w495) -> (w479:dbl)
            n184 = Boolean To (0,1)(Boolean=w472) -> (0, 1=w471:i16[])
            n185 = To Single Precision Float(number=w479) -> (single precision float=w527:sgl)
            n186 = case shown="True" w454 {
              tunnel: [w562 w580] -> w530
              tunnel: w532 -> [_ w582]
              tunnel: w527 -> [w563 w577]
              tunnel: [w561 w581] -> w534
              tunnel: w529 -> [_ _]
              tunnel: w455 -> [_ w578]
              tunnel: w453 -> [_ w568]
              frame False {
                # "Since no history available,\ncheck that current is with 0-360"
                # "Use Current Orientation bc \nPrevious are not available"
                # "New Position\nValid"
                n187 = In Range and Coerce(upper limit=sgl 360.0, x=w563, lower limit=sgl -360.0 ("upper limit")) -> (In Range?=w562:bool)  [unwired: 1 out]
                n188 = Select(t=w563, s=w562, f=sgl 0.0) -> (s? t:f=w561:sgl)
              }
              frame True {
                # "Moving Average Out"
                n189 = for {
                  N: w568 -> [_]
                  shift-right: [w606] -> w574
                  shift-left: 0.0 -> [w605]
                  tunnel: w578 -> [w604] mode=indexing
                  tunnel: w582 -> [w602]
                  # "Fetch Last Valid Values\nand Sum"
                  n190 = Index Array(array=w602, index=w604) -> (element=w603:sgl)
                  n191 = Add(x=w603, y=w605) -> (x+y=w606:dbl)
                }
                n192 = Subtract(x=sgl 1.0, y="New Orientation\nWeight") -> (x-y=w573:sgl)
                n193 = Multiply(x=w577, y="New Orientation\nWeight") -> (x*y=w571:sgl)
                n194 = Multiply(x=w573, y=w574) -> (x*y=w569:dbl)
                n195 = To Double Precision Float(number=w568) -> (double precision float=w567:dbl)
                n196 = Divide(x=w569, y=w567) -> (x/y=w570:dbl)
                n197 = Add(x=w571, y=w570) -> (x+y=w572:dbl)
                n198 = Greater Than 0?(x=w568) -> (x > 0?=w579:bool)
                n199 = case shown="True" w579 {
                  tunnel: w572 -> [w586 w592]
                  tunnel: w578 -> [_ w599]
                  tunnel: w582 -> [_ w598]
                  tunnel: [w585 w591] -> w581
                  tunnel: [w584 w594] -> w580
                  frame False {
                    # "No Pevious is Available to Compare\ncheck that current is real angle"
                    n200 = In Range and Coerce(upper limit=sgl 360.0, x=w586, lower limit=sgl -360.0 ("upper limit")) -> (In Range?=w584:bool)  [unwired: 1 out]
                    n201 = Select(t=w586, s=w584, f=sgl 0.0) -> (s? t:f=w585:dbl)
                  }
                  frame True {
                    # "Calculate New, Weighted\nOrientation"
                    # "Check That New Value\nis within Range of Old\n(avg)"
                    # "(X1 - X2)^2"
                    # "Previous"
                    # "Pevious is Available to Compare"
                    n202 = Index Array(array=w599, index=u8 0) -> (element=w600:u8)
                    n203 = Index Array(array=w598, index=w600) -> (element=w597:sgl)
                    n204 = Subtract(x=w597, y=w592) -> (x-y=w596:dbl)
                    n205 = Absolute Value(x=w596) -> (abs(x)=w595:dbl)
                    n206 = Less Or Equal?(x=w595, y="New Orientation \nThreshold") -> (x <= y?=w594:bool)
                    n207 = Select(t=w592, s=w594, f=sgl 0.0) -> (s? t:f=w591:dbl)
                  }
                }
              }
            }
            n208 = Add Array Elements(numeric array=w471) -> (sum=w470:i16)
            n209 = Greater?(x=w470, y=i16 2) -> (0:w468:bool)
            n210 = case shown="True" w468 {
              tunnel: w460 -> [_ w560]
              tunnel: w472 -> [w553 w559]
              tunnel: w475 -> [_ w558]
              tunnel: w474 -> [_ w557]
              tunnel: [w553 w556] -> w473
              tunnel: "Distance\nBetween Beacons" -> [_ w555]
              tunnel: "Distance\nBetween Beacons \n- Tolerance" -> [_ w554]
              frame False {
                # "Don't apply filtering,\nnot enough data points"
              }
              frame True {
                # "This will filter beacons if they are calculate to be \ntoo close to each other. The beacon(s) that is\n discarded is chosen based distance between each/every\nbeacon,. Capable of filtering as long as 1/2 of sample\nset has uniform distances (between beacons)."
                # "Validate Distance Between\nEach Beacon"
                n211 = call "Beacon_Filtering_Inter_Beacon_Distance_R1.vi"("Num of Beacons"=w560, "Inter Beacon\nReal Distance"=w555, "X in"=w558, "Inter Beacon\ndelta Threshold"=w554, "Y in"=w557, "Valid Data\nSets in"=w559) -> ("Beacons Valid - Out"=w556:bool[])  [unwired: 9 in]
              }
            }
            "Post Filtering\n- Valid Beacons" <- w473
            n212 = Increment(x=w460) -> (x+1=w517:i8)
            n213 = for {
              N: w517 -> [_]
              tunnel: [w722] -> w518 mode=indexing
              tunnel: w475 -> [w718]
              tunnel: w474 -> [w721]
              tunnel: [w720] -> w519 mode=indexing
              tunnel: w464 -> [w717]
              i -> [w719]
              # "Build Array's of Coordinates\nFor All Objects"
              n214 = Greater Than 0?(x=w719) -> (x > 0?=w723:bool)
              n215 = case shown="True" w723 {
                tunnel: [w725 w731] -> w722
                tunnel: w718 -> [w728 _]
                tunnel: w721 -> [w727 _]
                tunnel: [w724 0.0] -> w720
                tunnel: w719 -> [w729 _]
                tunnel: w717 -> [_ w731]
                frame True {
                  # "Rest of Array is\nBeacon Coordinates"
                  n216 = Decrement(x=w729) -> (x-1=w726:i32)
                  n217 = Index Array(array=w728, index=w726) -> (element=w725:sgl)
                  n218 = Index Array(array=w727, index=w726) -> (element=w724:sgl)
                }
                frame False {
                  # "First object is the\nother Camera\n\nthis coordinate\nis simply:\nx = 0\ny = distance btween cams"
                }
              }
            }
            n219 = Bundle(w518, w519) -> (→"All Object Coordinates \n- Local" →"Local Coordinates - Normalized":cluster{sgl[], dbl[]})  [unwired: 1 in]
            n220 = expression code="(x/180.0)*pi" "degrees to radians"(w534) -> (w478:dbl)
            n221 = call-poly <vilib>:"2D Cartesian Coordinate Rotation.vi"("theta"=w478, "Y"=w519, "X"=w518) -> ("Y Out"=w496:dbl[], "X Out"=w497:dbl[])  [unwired: 6 in, 1 out]
            n222 = Bundle("X Out"=w497, "Y Out"=w496) -> (→"All Object Coordinates \n- Local - Rotated" →"Local Coordinates - Rotated":cluster{"X Out":dbl[], "Y Out":dbl[]})  [unwired: 1 in]
            n223 = Index Array(array=w496, index=w516) -> (element=w492:dbl)
            n224 = Index Array(array=w497, index=w516) -> (element=w515:dbl)
            n225 = for {
              N: w460 -> [_]
              tunnel: w496 -> [w713]
              tunnel: w497 -> [w714]
              tunnel: w515 -> [w712]
              tunnel: w492 -> [w711]
              tunnel: [w710] -> w489 mode=indexing
              tunnel: [w709] -> w488 mode=indexing
              tunnel: [w708] -> w465 mode=indexing
              tunnel: [w707] -> w490 mode=indexing
              i -> [w716]
              n226 = Increment(x=w716) -> (x+1=w715:i32)
              n227 = Index Array(array=w713, index=w715) -> (element=w707:dbl)
              n228 = Index Array(array=w714, index=w715) -> (element=w708:dbl)
              n229 = Subtract(x=w707, y=w711) -> (x-y=w709:dbl)
              n230 = Subtract(x=w708, y=w712) -> (x-y=w710:dbl)
            }
            n231 = Bundle(w489, w488) -> (→"dX, dY\nRight Cam":cluster{dbl[], dbl[]})  [unwired: 1 in]
            n232 = Bundle(w465, w490) -> (→"dX, dY\nLeft Cam":cluster{dbl[], dbl[]})  [unwired: 1 in]
            n233 = Unbundle("Real Beacon\n - Coordinates") -> ("X"=w513:dbl[], "Y"=w493:dbl[])
            n234 = Boolean To (0,1)(Boolean=w473) -> (0, 1=w491:i16[])
            n235 = for {
              N: w460 -> [_]
              tunnel: w473 -> [w693] mode=indexing
              tunnel: w513 -> [w690] mode=indexing
              tunnel: w493 -> [w689] mode=indexing
              tunnel: w465 -> [w692] mode=indexing
              tunnel: w490 -> [w688] mode=indexing
              tunnel: w489 -> [w691] mode=indexing
              tunnel: w488 -> [w687] mode=indexing
              tunnel: [w686] -> w512 mode=indexing
              tunnel: [w685] -> w511 mode=indexing
              tunnel: [w684] -> w510 mode=indexing
              tunnel: [w683] -> w509 mode=indexing
              n236 = case shown="True" w693 {
                tunnel: w692 -> [_ w706]
                tunnel: w691 -> [_ w705]
                tunnel: w690 -> [_ w696]
                tunnel: w689 -> [_ w695]
                tunnel: w688 -> [_ w704]
                tunnel: w687 -> [_ w697]
                tunnel: [w694 w702] -> w686
                tunnel: [w694 w701] -> w685
                tunnel: [w694 w700] -> w684
                tunnel: [w694 w699] -> w683
                frame False {
                  w694 = sgl 0.0
                  # "Add Nothing"
                }
                frame True {
                  # "realX = beaconX + dY\nrealY = beaconY + (-dx)"
                  # "Right Cam"
                  # "Left Cam"
                  # "dX = -dX\nSwap dX, dY"
                  # "Translate to Real Coordinates\nOnly Apply for Valid Beacons"
                  n237 = Negate(x=w706) -> (-x=w703:dbl)
                  n238 = Negate(x=w705) -> (-x=w698:dbl)
                  n239 = Add(x=w696, y=w704) -> (x+y=w702:dbl)
                  n240 = Add(x=w695, y=w703) -> (x+y=w701:dbl)
                  n241 = Add(x=w696, y=w697) -> (x+y=w700:dbl)
                  n242 = Add(x=w695, y=w698) -> (x+y=w699:dbl)
                }
              }
            }
            n243 = Add Array Elements(numeric array=w491) -> (sum=w494:i16)
            n244 = Add Array Elements(numeric array=w512) -> (sum=w508:dbl)
            n245 = Add Array Elements(numeric array=w511) -> (sum=w507:dbl)
            n246 = Add Array Elements(numeric array=w510) -> (sum=w506:dbl)
            n247 = Add Array Elements(numeric array=w509) -> (sum=w505:dbl)
            n248 = Divide(x=w508, y=w494) -> (x/y=w504:dbl)
            n249 = Divide(x=w507, y=w494) -> (x/y=w502:dbl)
            n250 = Divide(x=w506, y=w494) -> (x/y=w503:dbl)
            n251 = Divide(x=w505, y=w494) -> (x/y=w501:dbl)
            n252 = Bundle(w504, w502) -> (→"Left Camera Real Coordinates":cluster{dbl, dbl})  [unwired: 1 in]
            n253 = Bundle(w503, w501) -> (→"Right Camera Real Coordinate":cluster{dbl, dbl})  [unwired: 1 in]
            n254 = Add(x=w504, y=w503) -> (x+y=w500:dbl)
            n255 = Add(x=w502, y=w501) -> (x+y=w498:dbl)
            n256 = Divide(x=w500, y=w499) -> (x/y=w482:dbl)
            n257 = Divide(x=w498, y=w499) -> (x/y=w481:dbl)
            n258 = Bundle(w482, w481) -> (→"Robot Coordinates":cluster{dbl, dbl})  [unwired: 1 in]
            n259 = Less Than 0?(x=w481) -> ()  [unwired: 1 out]
            n260 = case shown="True" w454 {
              tunnel: w451 -> [_ _]
              tunnel: w482 -> [w611 w632]
              tunnel: [w612 w642] -> w531
              tunnel: w535 -> [_ w636]
              tunnel: w481 -> [w610 w619]
              tunnel: [w609 w646] -> w533
              tunnel: "Max X (arena)" -> [w608 w641]
              tunnel: "Max Y (arena)" -> [w607 w640]
              tunnel: w455 -> [_ w638]
              tunnel: w453 -> [_ w637]
              frame False {
                # "New Position\nValid"
                # "Since no history available,\ncheck that current is within\nthe bounds of the arena size"
                # "Use Current Position bc \nPrevious are not available"
                n261 = In Range and Coerce(upper limit=w608, x=w611, lower limit=sgl 0.0 ("upper limit")) -> (In Range?=w614:bool)  [unwired: 1 out]
                n262 = In Range and Coerce(upper limit=w607, x=w610, lower limit=sgl 0.0 ("upper limit")) -> (In Range?=w613:bool)  [unwired: 1 out]
                n263 = Bundle(w611, w610) -> (w609:cluster{dbl, dbl})  [unwired: 1 in]
                n264 = And(x=w614, y=w613) -> (x .and. y?=w612:bool)
              }
              frame True {
                w639 = 0.0
                # "If needed, make seperate FOR Loop for \nY only... Using more previous values than X"
                # "New Y"
                # "New X"
                # "Only consider if velocity is\ngreater than certain speed"
                # "Weighted Robot \nCoordinates"
                # "Position\nValid\n(current)"
                n265 = for {
                  N: w637 -> [_]
                  shift-right: [w655] -> w635
                  shift-left: w639 -> [w654]
                  shift-right: [w653] -> w620
                  shift-left: w639 -> [w652]
                  tunnel: w638 -> [w650] mode=indexing
                  tunnel: w636 -> [w648]
                  # "Fetch Last Valid Values\nand Sum"
                  n266 = Index Array(array=w648, index=w650) -> (element=w649:cluster{sgl, sgl})
                  n267 = Unbundle(w649) -> (w651:sgl, w647:sgl)
                  n268 = Add(x=w647, y=w652) -> (x+y=w653:dbl)
                  n269 = Add(x=w651, y=w654) -> (x+y=w655:dbl)
                }
                n270 = Subtract(x=sgl 1.0, y="New Position\nWeight (X coord)") -> (x-y=w634:sgl)
                n271 = Subtract(x=sgl 1.0, y="New Position\nWeight (Y coord)") -> (x-y=w618:sgl)
                n272 = To Single Precision Float(number=w637) -> (single precision float=w626:sgl)
                n273 = Multiply(x=w634, y=w635) -> (x*y=w627:dbl)
                n274 = Multiply(x=w620, y=w618) -> (x*y=w628:dbl)
                n275 = Divide(x=w627, y=w626) -> (x/y=w624:dbl)
                n276 = Divide(x=w628, y=w626) -> (x/y=w625:dbl)
                n277 = Multiply(x="New Position\nWeight (X coord)", y=w632) -> (x*y=w630:dbl)
                n278 = Multiply(x=w619, y="New Position\nWeight (Y coord)") -> (x*y=w629:dbl)
                n279 = Add(x=w630, y=w624) -> (x+y=w623:dbl)
                n280 = Add(x=w629, y=w625) -> (x+y=w622:dbl)
                n281 = Greater Than 0?(x=w637) -> (x > 0?=w645:bool)
                n282 = case shown="True" w645 {
                  tunnel: w623 -> [w660 w667]
                  tunnel: w622 -> [w659 w666]
                  tunnel: w638 -> [_ w679]
                  tunnel: w636 -> [_ w678]
                  tunnel: [w657 w667] -> w644
                  tunnel: [w656 w666] -> w643
                  tunnel: [w661 w668] -> w642
                  tunnel: w641 -> [w663 _]
                  tunnel: w640 -> [w662 _]
                  frame False {
                    w658 = sgl 0.0 ("upper limit")
                    # "Check that within bounds of arena"
                    # "No Pevious is Available to Compare"
                    n283 = In Range and Coerce(upper limit=w663, x=w660, lower limit=w658) -> (In Range?=w665:bool)  [unwired: 1 out]
                    n284 = In Range and Coerce(upper limit=w662, x=w659, lower limit=w658) -> (In Range?=w664:bool)  [unwired: 1 out]
                    n285 = And(x=w665, y=w664) -> (x .and. y?=w661:bool)
                    n286 = Select(t=w660, s=w661, f=w658) -> (s? t:f=w657:dbl)
                    n287 = Select(t=w659, s=w661, f=w658) -> (s? t:f=w656:dbl)
                  }
                  frame True {
                    # "New"
                    # "(Y1 - Y2)^2"
                    # "(X1 - X2)^2"
                    # "Previous"
                    # "Pevious is Available to Compare"
                    n288 = Index Array(array=w679, index=u8 0) -> (element=w681:u8)
                    n289 = Index Array(array=w678, index=w681) -> (element=w680:cluster{sgl, sgl})
                    n290 = Unbundle(w680) -> (w670:sgl, w669:sgl)
                    n291 = Subtract(x=w670, y=w667) -> (x-y=w675:dbl)
                    n292 = Subtract(x=w666, y=w669) -> (x-y=w674:dbl)
                    n293 = Square(x=w675) -> (x^2=w673:dbl)
                    n294 = Square(x=w674) -> (x^2=w672:dbl)
                    n295 = Add(x=w673, y=w672) -> (x+y=w676:dbl)
                    n296 = Square Root(x=w676) -> (sqrt(x)=w671:dbl)
                    n297 = Less Or Equal?(x=w671, y="New Position \nThreshold") -> (x <= y?=w668:bool)
                  }
                }
                n298 = Bundle("upper limit"=w644, "upper limit"=w643) -> (w646:cluster{"upper limit":dbl, "upper limit":dbl})  [unwired: 1 in]
              }
            }
          }
        }
        "Orietnation\n(current)" <- w183
        n299 = And(x=w193, y=w192) -> (x .and. y?=w134:bool)
        "Position Valid" <- w134
        n300 = Exclusive Or(1:w192, 2:w193) -> (0:w191:bool)
        n301 = case shown="True" w134 {
          tunnel: [w738 w741] -> w135
          tunnel: [w739 w740] -> w138
          tunnel: w205 -> [_ w741]
          tunnel: w204 -> [_ w740]
          tunnel: w191 -> [_ _]
          frame False {
            w738 = sgl 0.0 ("f")
            n302 = Bundle("f"=w738, "f"=w738) -> (w739:cluster{"f":sgl, "f":sgl})  [unwired: 1 in]
          }
          frame True {
            # "For Servos"
            "Last Orientation" <- w741
            "Last Position" <- w740
          }
        }
        "Robot Coordinates - Avgd" <- w138
        "Orientation Avgd" <- w135
        n303 = local read "History Size"() -> (w185:u8)
        n304 = Decrement(x=w185) -> (x-1=w186:u8)
        n305 = for {
          N: w185 -> [_]
          shift-right: [w779] -> w207
          shift-left: w203 -> [w778]
          tunnel: w138 -> [w777]
          tunnel: w186 -> [w776]
          i -> [w775]
          n306 = Subtract(x=w776, y=w775) -> (x-y=w774:i32)
          n307 = Equal To 0?(x=w774) -> (x = 0?=w773:bool)
          n308 = case shown="False" w773 {
            tunnel: w774 -> [w781 w786]
            tunnel: w778 -> [w784 w787]
            tunnel: [w782 w788] -> w779
            tunnel: w777 -> [_ w785]
            frame False {
              n309 = Decrement(x=w781) -> (x-1=w780:i32)
              n310 = Index Array(array=w784, index=w780) -> (element=w783:cluster{sgl, sgl})
              n311 = Replace Array Subset(array=w784, new element=w783, index=w781) -> (w782:cluster{sgl, sgl}[])
            }
            frame True {
              n312 = Replace Array Subset(array=w787, new element=w785, index=w786) -> (w788:cluster{sgl, sgl}[])
            }
          }
        }
        n313 = Unbundle(w138) -> ("upper limit"=w137:dbl, "upper limit"=w136:dbl)
        n314 = shared-variable "RT myRIO Target - Overlord\\Localization_Variables_r0.lvlib\\loc_x"(w137) -> ()  [unwired: 1 in, 1 out]
        n315 = shared-variable "RT myRIO Target - Overlord\\Localization_Variables_r0.lvlib\\loc_y"(w136) -> ()  [unwired: 1 in, 1 out]
        n316 = shared-variable "RT myRIO Target - Overlord\\Localization_Variables_r0.lvlib\\loc_theta"(w135) -> ()  [unwired: 1 in, 1 out]
        n317 = shared-variable "RT myRIO Target - Overlord\\Localization_Variables_r0.lvlib\\loc_flag"(w134) -> ()  [unwired: 1 in, 1 out]
        n318 = Decrement(x=w185) -> (x-1=w187:u8)
        n319 = for {
          N: w185 -> [_]
          shift-right: [w763] -> w208
          shift-left: w202 -> [w762]
          tunnel: w135 -> [w761]
          tunnel: w187 -> [w760]
          i -> [w759]
          n320 = Subtract(x=w760, y=w759) -> (x-y=w757:i32)
          n321 = Equal To 0?(x=w757) -> (x = 0?=w758:bool)
          n322 = case shown="False" w758 {
            tunnel: w757 -> [w765 w770]
            tunnel: w762 -> [w768 w771]
            tunnel: [w766 w772] -> w763
            tunnel: w761 -> [_ w769]
            frame False {
              # "Shift"
              n323 = Decrement(x=w765) -> (x-1=w764:i32)
              n324 = Index Array(array=w768, index=w764) -> (element=w767:sgl)
              n325 = Replace Array Subset(array=w768, new element=w767, index=w765) -> (w766:sgl[])
            }
            frame True {
              # "insert new"
              n326 = Replace Array Subset(array=w771, new element=w769, index=w770) -> (w772:sgl[])
            }
          }
        }
        n327 = Decrement(x=w185) -> (x-1=w184:u8)
        n328 = for {
          N: w185 -> [_]
          shift-right: [w748] -> w206
          shift-left: w201 -> [w747]
          tunnel: w134 -> [w746]
          tunnel: w184 -> [w745]
          i -> [w744]
          n329 = Subtract(x=w745, y=w744) -> (x-y=w742:i32)
          n330 = Equal To 0?(x=w742) -> (x = 0?=w743:bool)
          n331 = case shown="False" w743 {
            tunnel: w747 -> [w753 w755]
            tunnel: [w751 w756] -> w748
            tunnel: w746 -> [_ w754]
            tunnel: w742 -> [w749 _]
            frame False {
              n332 = Decrement(x=w749) -> (x-1=w750:i32)
              n333 = Index Array(array=w753, index=w750) -> (element=w752:bool)
              n334 = Replace Array Subset(array=w753, new element=w752, index=w749) -> (w751:bool[])
            }
            frame True {
              n335 = Replace Array Subset(array=w755, new element=w754) -> (w756:bool[])  [unwired: 1 in]
            }
          }
        }
        n336 = Boolean To (0,1)(Boolean=w206) -> (0, 1=w198:i16[])
        n337 = Add Array Elements(numeric array=w198) -> (sum=w197:i16)
        n338 = Greater Or Equal?(x=w197, y=i16 2) -> (x >= y?=w130:bool)
        "Position \nLock Status" <- w130
        n339 = shared-variable "RT myRIO Target - Overlord\\Localization_Variables_r0.lvlib\\Position_Lock"(w130) -> ()  [unwired: 1 in, 1 out]
        n340 = case shown="True" w134 {
          tunnel: w138 -> [_ w737]
          frame False {
          }
          frame True {
            # "update debug graph\nif current is valid"
            n341 = Unbundle(w737) -> ("upper limit"=w736:dbl, "upper limit"=w735:dbl)
            n342 = Build Array(w735) -> (w733:dbl[])
            n343 = Build Array(w736) -> (w734:dbl[])
            n344 = Bundle(w734, w733) -> (→"Real Position in Course 2":cluster{dbl[], dbl[]})  [unwired: 1 in]
          }
        }
      }
    }
    n345 = case shown="True" w113 {
      tunnel: w112 -> [_ w120]
      frame False {
      }
      frame True {
        n346 = call "Tick Count3"() -> ("Tick Count(uSec)"=w121:u32)
        n347 = Subtract(x=w121, y=w120) -> (x-y=w124:u32)
        n348 = Divide(x=w124, y=u32 1000 ("x")) -> (x/y=→"dT":dbl)
      }
    }
    n349 = call "Tick Count6"() -> ("Tick Count(uSec)"=w110:u32)
    "Robot Coordinates\nHistory" <- w109
    "Orientation\nHistory" <- w114
    "Position Valid\nHistory" <- w115
  }
  n350 = disable-structure shown="Enabled" {
    disable-tunnel: [w791 _] -> _
    disable-tunnel: ["Search Step Size\n(deg)" _] -> _
    frame Enabled {
      n351 = Multiply(x=3.413333333333333, y="Search Step Size\n(deg)") -> (x*y=w789:dbl)
      n352 = To Unsigned Word Integer(number=w789) -> (unsigned 16bit integer=w791:u16)
    }
    frame Disabled {
    }
  }
  n353 = Multiply(x="Move Servo\nThreshold (deg)", y=3.413333333333333) -> (x*y=w18:dbl)
  n354 = To Unsigned Word Integer(number=w18) -> ()  [unwired: 1 out]
  n355 = call "Tick Count8"() -> ()  [unwired: 1 out]
  n356 = flat-sequence {
    tunnel: [w795] -> w42
    tunnel: [w794] -> w41
    tunnel: [w799] -> w40
    tunnel: ["Left Servo\nID"] -> w29
    tunnel: ["Right Servo\nID"] -> w28
    tunnel: ["Compliance Slope"] -> w27
    tunnel: [w839] -> w39
    tunnel: [w838] -> w38
    tunnel: w42 -> [w837]
    tunnel: w41 -> [w836]
    tunnel: w40 -> [w835]
    tunnel: w29 -> [w833]
    tunnel: w28 -> [w832]
    tunnel: w27 -> [w831]
    tunnel: w39 -> [w1112]
    tunnel: w38 -> [w1111]
    frame #0 {
      # "BAUD RATE"
      # "Initialize UART and DIO"
      n357 = call-poly "VISA Configure Serial Port"("VISA resource name"=refnum<visa-resource-name> "ASRL1::INSTR", "Enable Termination\nChar (T)"=FALSE ("Enable Termination\nChar (T)"), "baud rate (9600)"=u32 115200) -> ("VISA resource name out"=w795:refnum<visa-resource-name>)  [unwired: 11 in, 1 out]
      n358 = call <vilib>:"Smart Open.vi"("Channel Names"=tag[] ["A/DIO2"]) -> ("DIO Ref Out"=w794:T8)  [unwired: 9 in, 1 out]
      n359 = flat-sequence {
        tunnel: w795 -> [w807]
        tunnel: w794 -> [w806]
        tunnel: "Left Servo\nID" -> [w808]
        tunnel: [w805] -> w796
        tunnel: "Compliance Slope" -> [w804]
        tunnel: "Right Servo\nID" -> [w821]
        tunnel: w796 -> [w820]
        tunnel: "Compliance Slope" -> [w819]
        tunnel: w795 -> [w818]
        tunnel: w794 -> [w817]
        frame #0 {
          w805 = 3
          n360 = while {
            tunnel: w805 -> [w814]
            tunnel: w807 -> [w812]
            tunnel: w806 -> [w811]
            tunnel: w808 -> [w810]
            tunnel: w804 -> [w809]
            i -> [w815]
            stop <- w813 stop-if-true
            n361 = call "Set_Compliance_Slope_R2.vi"("Compliance Slope"=w809, "DIO Ref Out"=w811, "VISA resource name"=w812, "Servo ID"=w810) -> ()  [unwired: 6 in, 2 out]
            n362 = Increment(x=w815) -> (x+1=w816:i32)
            n363 = Greater Or Equal?(x=w816, y=w814) -> (x >= y?=w813:bool)
          }
        }
        frame #1 {
          n364 = while {
            tunnel: w820 -> [w827]
            tunnel: w821 -> [w825]
            tunnel: w818 -> [w824]
            tunnel: w817 -> [w823]
            tunnel: w819 -> [w822]
            i -> [w828]
            stop <- w826 stop-if-true
            n365 = call "Set_Compliance_Slope_R2.vi"("Compliance Slope"=w822, "DIO Ref Out"=w823, "VISA resource name"=w824, "Servo ID"=w825) -> ()  [unwired: 6 in, 2 out]
            n366 = Increment(x=w828) -> (x+1=w829:i32)
            n367 = Greater Or Equal?(x=w829, y=w827) -> (x >= y?=w826:bool)
          }
        }
      }
      n368 = call "Tick Count"() -> ("Tick Count(uSec)"=w799:u32)
    }
    frame #1 {
      # "Service Count"
      n369 = while {
        shift-right: [w842] -> _
        shift-left: w835 -> [w859]
        tunnel: "Max Write\nTx Attempts" -> [w854]
        tunnel: "Max Read\nTx Attempts" -> [w853]
        shift-right: [w849] -> w839
        shift-left: w837 -> [w852]
        shift-right: [w848] -> w838
        shift-left: w836 -> [w851]
        tunnel: w833 -> [w847]
        tunnel: w832 -> [w846]
        tunnel: w831 -> [w845]
        shift-right: [w843] -> _
        shift-left: u16 0 -> [w844]
        stop <- "close comms" stop-if-true
        # "Loop Timer"
        n370 = local read "SERVO ENABLE"() -> (w841:bool)
        n371 = call "Tick Count2"() -> ("Tick Count(uSec)"=w842:u32)
        n372 = Subtract(x=w842, y=w859) -> (x-y=w858:u32)
        n373 = call "Wait4"("Count(mSec)"="Servo Comm\nLoop Time (ms)") -> ()  [unwired: 1 out]
        n374 = Divide(x=w858, y=u32 1000) -> (x/y=→"dT - Comm Loop":dbl)
        n375 = case shown="True" w841 {
          tunnel: w854 -> [_ w868]
          tunnel: w853 -> [_ w899]
          tunnel: w852 -> [w862 w863]
          tunnel: w851 -> [w861 w892]
          tunnel: [w862 w865] -> w849
          tunnel: [w861 w864] -> w848
          tunnel: w847 -> [_ w871]
          tunnel: w846 -> [_ w870]
          tunnel: w845 -> [_ w869]
          tunnel: w844 -> [_ w867]
          tunnel: [u16 100 w866] -> w843
          frame False {
            # "Restart at same value\nUsed to Periodically update \nCompliance Slope"
          }
          frame True {
            n376 = flat-sequence {
              tunnel: [w905] -> w903
              tunnel: [w906] -> w902
              tunnel: [w904] -> w901
              tunnel: w899 -> [w907]
              tunnel: [w909] -> w890
              tunnel: [w908] -> w888
              tunnel: w863 -> [w909]
              tunnel: w892 -> [w908]
              tunnel: w871 -> [w904]
              tunnel: w903 -> [w927]
              tunnel: w902 -> [w928]
              tunnel: w901 -> [w926]
              tunnel: [w926] -> w900
              tunnel: [w925] -> w893
              tunnel: [w924] -> w891
              tunnel: w890 -> [w924]
              tunnel: [w923] -> w889
              tunnel: w888 -> [w923]
              tunnel: w900 -> [w949]
              tunnel: w868 -> [w948]
              tunnel: w893 -> [w943]
              tunnel: w891 -> [w945]
              tunnel: w889 -> [w944]
              tunnel: [w945] -> w886
              tunnel: [w944] -> w884
              tunnel: [w982] -> w887
              tunnel: w886 -> [w982]
              tunnel: [w981] -> w885
              tunnel: w884 -> [w981]
              tunnel: ["Servo Comm\nWait Time - (ms)"] -> w876
              tunnel: w899 -> [w989]
              tunnel: [w988] -> w898
              tunnel: [w987] -> w897
              tunnel: [w983] -> w895
              tunnel: w887 -> [w986]
              tunnel: w885 -> [w985]
              tunnel: [w986] -> w883
              tunnel: [w985] -> w880
              tunnel: [w984] -> w877
              tunnel: w876 -> [w984]
              tunnel: w870 -> [w983]
              tunnel: w898 -> [w1009]
              tunnel: w897 -> [w1008]
              tunnel: [w1007] -> w896
              tunnel: w895 -> [w1007]
              tunnel: [w1006] -> w894
              tunnel: w883 -> [w1005]
              tunnel: [w1005] -> w882
              tunnel: [w1004] -> w881
              tunnel: w880 -> [w1004]
              tunnel: w877 -> [w1003]
              tunnel: [w1003] -> w875
              tunnel: w896 -> [w1031]
              tunnel: w894 -> [w1029]
              tunnel: w868 -> [w1030]
              tunnel: w882 -> [w1028]
              tunnel: w881 -> [w1027]
              tunnel: [w1028] -> w879
              tunnel: [w1027] -> w878
              tunnel: w875 -> [w1024]
              tunnel: [w1024] -> w874
              tunnel: w879 -> [w1064]
              tunnel: w878 -> [w1063]
              tunnel: w874 -> [w1062]
              tunnel: [w1064] -> w873
              tunnel: [w1063] -> w872
              tunnel: w873 -> [w1068]
              tunnel: w872 -> [w1067]
              tunnel: w871 -> [w1073]
              tunnel: w870 -> [w1072]
              tunnel: w869 -> [w1071]
              tunnel: w867 -> [w1066]
              tunnel: w868 -> [w1070]
              tunnel: [w1069] -> w866
              tunnel: [w1068] -> w865
              tunnel: [w1067] -> w864
              frame #0 {
                n377 = while {
                  tunnel: [w922] -> w905
                  tunnel: w904 -> [w921]
                  tunnel: [w914] -> w906
                  tunnel: w907 -> [w912]
                  tunnel: w909 -> [w911]
                  tunnel: w908 -> [w910]
                  i -> [w913]
                  stop <- w915 stop-if-true
                  # "Attemp to Read Until\nMax Read Tx Attemps Limit"
                  n378 = call "ReadServo_R3.vi"("DIO Ref In"=w910, "VISA resource name out"=w911, "Servo ID"=w921) -> ("Error"=w918:u8, "Valid Checksum"=w919:bool, "Current Position"=w922:u64)  [unwired: 6 in]
                  n379 = Increment(x=w913) -> (x+1=w916:i32)
                  n380 = Equal To 0?(x=w918) -> (x = 0?=w920:bool)
                  n381 = Greater Or Equal?(x=w916, y=w912) -> (x >= y?=w917:bool)
                  n382 = And(x=w919, y=w920) -> (x .and. y?=w914:bool)
                  n383 = Or(x=w914, y=w917) -> (x .or. y?=w915:bool)
                }
              }
              frame #1 {
                # "Read Position First"
                n384 = local read "Servo Goal Position\n - Left"() -> (w925:u16)
                n385 = case shown="True" w928 {
                  tunnel: w927 -> [_ w933]
                  tunnel: w925 -> [_ w931]
                  frame False {
                  }
                  frame True {
                    # "Convert Received Position to Angle Relative to Robot"
                    # "45 DEG MOUNT OFFSET"
                    # "1024/300"
                    n386 = local write "Current L (10bit)"(w933) -> ()
                    n387 = To Word Integer(number=w933) -> (16bit integer=w937:i16)
                    n388 = To Word Integer(number=w931) -> (16bit integer=w936:i16)
                    n389 = Subtract(x=w936, y=w937) -> (x-y=w935:i16)
                    n390 = Divide(x=w933, y=3.413333333333333) -> (x/y=w941:dbl)
                    n391 = Absolute Value(x=w935) -> (abs(x)=w934:i16)
                    n392 = Subtract(x=w941, y=sgl 60.0) -> (x-y=w939:dbl)
                    n393 = Greater?(x=w934, y=u16 5) -> (0:w930:bool)
                    n394 = Add(x=w939, y=sgl 45.0) -> (x+y=w929:dbl)
                    n395 = local write "Move Servo - L"(w930) -> ()
                    n396 = local write "Servo Moving - L"(w930) -> ()
                    n397 = local write "Current Angle\n - Left (internal)"(w929) -> ()
                    n398 = shared-variable "RT myRIO Target - Overlord\\Localization_Variables_r0.lvlib\\Left Servo Angle_Current"(w929) -> ()  [unwired: 1 in, 1 out]
                  }
                }
              }
              frame #2 {
                n399 = local read "Move Servo - L"() -> (w946:bool)
                n400 = case shown="True" w946 {
                  tunnel: w949 -> [_ w964]
                  tunnel: w943 -> [_ w951]
                  tunnel: [TRUE w962] -> w947
                  tunnel: w948 -> [_ w954]
                  tunnel: w945 -> [_ w953]
                  tunnel: w944 -> [_ w952]
                  frame False {
                    # "Only Send if Current Position is far enough"
                  }
                  frame True {
                    w960 = 1
                    # "High Byte"
                    # "Low Byte"
                    n401 = Type Cast(type="", x=w951) -> (*(type *) &x=w961:string)
                    n402 = local write "Servo Moving - L"(TRUE) -> ()
                    n403 = String Subset(string=w961, offset (0)=1, length (rest)=w960) -> (substring=w956:string)
                    n404 = String Subset(string=w961, offset (0)=0, length (rest)=w960) -> (substring=w955:string)
                    n405 = while {
                      tunnel: w964 -> [w978]
                      tunnel: [w970] -> w962
                      tunnel: w956 -> [w974]
                      tunnel: w955 -> [w973]
                      tunnel: w954 -> [w967]
                      tunnel: w953 -> [w966]
                      tunnel: w952 -> [w965]
                      i -> [w968]
                      stop <- w969 stop-if-true
                      # "Attemp to Write Until\nMax Write Tx Attemps Limit"
                      n406 = call "MoveServo_R3.vi"("DIO Ref Out"=w965, "VISA resource name out"=w966, "GP - Low Byte"=w974, "GP - High Byte"=w973, "Servo ID"=w978) -> ("Valid Checksum"=w975:bool, "Error"=w977:u64)  [unwired: 5 in]
                      n407 = Equal To 0?(x=w977) -> (x = 0?=w976:bool)
                      n408 = And(x=w975, y=w976) -> (x .and. y?=w970:bool)
                      n409 = Increment(x=w968) -> (x+1=w972:i32)
                      n410 = Greater Or Equal?(x=w972, y=w967) -> (x >= y?=w971:bool)
                      n411 = Or(x=w970, y=w971) -> (x .or. y?=w969:bool)
                    }
                  }
                }
                n412 = case shown="True" w947 {
                  frame False {
                  }
                  frame True {
                    # "Update Servo flag"
                    n413 = local write "Move Servo - L"(FALSE) -> ()
                  }
                }
              }
              frame #3 {
                n414 = call "Wait2"("Count(mSec)"="Servo Comm\nWait Time - (ms)") -> ()  [unwired: 1 out]
              }
              frame #4 {
                n415 = while {
                  tunnel: [w1002] -> w988
                  tunnel: w983 -> [w1001]
                  tunnel: [w994] -> w987
                  tunnel: w989 -> [w992]
                  tunnel: w986 -> [w991]
                  tunnel: w985 -> [w990]
                  i -> [w993]
                  stop <- w995 stop-if-true
                  # "Attemp to Read Until\nMax Read Tx Attemps Limit"
                  n416 = call "ReadServo_R3.vi"("DIO Ref In"=w990, "VISA resource name out"=w991, "Servo ID"=w1001) -> ("Error"=w998:u8, "Valid Checksum"=w999:bool, "Current Position"=w1002:u64)  [unwired: 6 in]
                  n417 = Increment(x=w993) -> (x+1=w996:i32)
                  n418 = Equal To 0?(x=w998) -> (x = 0?=w1000:bool)
                  n419 = Greater Or Equal?(x=w996, y=w992) -> (x >= y?=w997:bool)
                  n420 = And(x=w999, y=w1000) -> (x .and. y?=w994:bool)
                  n421 = Or(x=w994, y=w997) -> (x .or. y?=w995:bool)
                }
              }
              frame #5 {
                n422 = local read "Servo Goal Position\n - Right"() -> (w1006:u16)
                n423 = case shown="True" w1008 {
                  tunnel: w1009 -> [_ w1013]
                  tunnel: w1006 -> [_ w1012]
                  frame False {
                    # "Don't update current position"
                  }
                  frame True {
                    # "Convert Received Position to Angle Relative to Robot"
                    # "45 DEG MOUNT OFFSET"
                    # "1024/300"
                    n424 = local write "Current R (10bit)"(w1013) -> ()
                    n425 = Divide(x=w1013, y=3.413333333333333) -> (x/y=w1022:dbl)
                    n426 = Subtract(x=w1022, y=sgl 60.0) -> (x-y=w1020:dbl)
                    n427 = Subtract(x=w1020, y=sgl 45.0) -> (x-y=w1010:dbl)
                    n428 = To Word Integer(number=w1012) -> (16bit integer=w1017:i16)
                    n429 = To Word Integer(number=w1013) -> (16bit integer=w1018:i16)
                    n430 = shared-variable "RT myRIO Target - Overlord\\Localization_Variables_r0.lvlib\\Right Servo Angle_Current"(w1010) -> ()  [unwired: 1 in, 1 out]
                    n431 = local write "Current Angle\n - Right (internal)"(w1010) -> ()
                    n432 = Subtract(x=w1017, y=w1018) -> (x-y=w1016:i16)
                    n433 = Absolute Value(x=w1016) -> (abs(x)=w1015:i16)
                    n434 = Greater?(x=w1015, y=u16 5) -> (0:w1011:bool)
                    n435 = local write "Move Servo - R"(w1011) -> ()
                    n436 = local write "Servo Moving - R"(w1011) -> ()
                  }
                }
              }
              frame #6 {
                n437 = local read "Move Servo - R"() -> (w1025:bool)
                n438 = case shown="True" w1025 {
                  tunnel: w1029 -> [_ w1034]
                  tunnel: w1031 -> [_ w1041]
                  tunnel: [TRUE w1042] -> w1026
                  tunnel: w1030 -> [_ w1037]
                  tunnel: w1028 -> [_ w1036]
                  tunnel: w1027 -> [_ w1035]
                  frame False {
                  }
                  frame True {
                    w1044 = 1
                    # "High Byte"
                    # "Low Byte"
                    n439 = Type Cast(type="", x=w1034) -> (*(type *) &x=w1043:string)
                    n440 = local write "Servo Moving - R"(TRUE) -> ()
                    n441 = String Subset(string=w1043, offset (0)=1, length (rest)=w1044) -> (substring=w1040:string)
                    n442 = String Subset(string=w1043, offset (0)=0, length (rest)=w1044) -> (substring=w1039:string)
                    n443 = while {
                      tunnel: [w1053] -> w1042
                      tunnel: w1041 -> [w1058]
                      tunnel: w1040 -> [w1057]
                      tunnel: w1039 -> [w1056]
                      tunnel: w1037 -> [w1051]
                      tunnel: w1036 -> [w1049]
                      tunnel: w1035 -> [w1048]
                      i -> [w1052]
                      stop <- w1050 stop-if-true
                      # "Attemp to Write Until\nMax Write Tx Attemps Limit"
                      n444 = call "MoveServo_R3.vi"("DIO Ref Out"=w1048, "VISA resource name out"=w1049, "GP - Low Byte"=w1057, "GP - High Byte"=w1056, "Servo ID"=w1058) -> ("Valid Checksum"=w1060:bool, "Error"=w1059:u64)  [unwired: 5 in]
                      n445 = Increment(x=w1052) -> (x+1=w1054:i32)
                      n446 = Greater Or Equal?(x=w1054, y=w1051) -> (x >= y?=w1055:bool)
                      n447 = Equal To 0?(x=w1059) -> (x = 0?=w1061:bool)
                      n448 = And(x=w1060, y=w1061) -> (x .and. y?=w1053:bool)
                      n449 = Or(x=w1053, y=w1055) -> (x .or. y?=w1050:bool)
                    }
                  }
                }
                n450 = case shown="True" w1026 {
                  frame False {
                  }
                  frame True {
                    # "Update Servo flag"
                    n451 = local write "Move Servo - R"(FALSE) -> ()
                  }
                }
              }
              frame #7 {
                n452 = call "Wait3"("Count(mSec)"=w1062) -> ()  [unwired: 1 out]
              }
              frame #8 {
                # "Increment Service Count"
                # "Update Compliance Slope\nEvery x loops"
                n453 = Equal?(x=w1066, y=u16 1000) -> (x = y?=w1075:bool)
                n454 = case shown="True" w1075 {
                  tunnel: w1071 -> [_ w1085]
                  tunnel: w1068 -> [_ w1084]
                  tunnel: w1067 -> [_ w1083]
                  tunnel: w1068 -> [_ w1082]
                  tunnel: w1067 -> [_ w1081]
                  tunnel: w1073 -> [_ w1080]
                  tunnel: w1072 -> [_ w1079]
                  tunnel: w1066 -> [w1076 _]
                  tunnel: [w1076 u16 0] -> w1074
                  tunnel: w1070 -> [_ w1077]
                  frame False {
                  }
                  frame True {
                    # "Reset Service\nCount"
                    n455 = flat-sequence {
                      tunnel: w1084 -> [w1090]
                      tunnel: w1083 -> [w1089]
                      tunnel: w1080 -> [w1091]
                      tunnel: [w1087] -> w1086
                      tunnel: w1085 -> [w1088]
                      tunnel: w1077 -> [w1087]
                      tunnel: w1079 -> [w1103]
                      tunnel: w1086 -> [w1102]
                      tunnel: w1085 -> [w1101]
                      tunnel: w1082 -> [w1100]
                      tunnel: w1081 -> [w1099]
                      frame #0 {
                        n456 = while {
                          tunnel: w1087 -> [w1098]
                          tunnel: w1090 -> [w1096]
                          tunnel: w1089 -> [w1095]
                          tunnel: w1091 -> [w1094]
                          tunnel: w1088 -> [w1093]
                          i -> [w1092]
                          stop <- w1097 stop-if-true
                          n457 = call "Set_Compliance_Slope_R2.vi"("Compliance Slope"=w1093, "DIO Ref Out"=w1095, "VISA resource name"=w1096, "Servo ID"=w1094) -> ()  [unwired: 6 in, 2 out]
                          n458 = Greater Or Equal?(x=w1092, y=w1098) -> (x >= y?=w1097:bool)
                        }
                      }
                      frame #1 {
                        n459 = while {
                          tunnel: w1102 -> [w1110]
                          tunnel: w1103 -> [w1108]
                          tunnel: w1100 -> [w1107]
                          tunnel: w1099 -> [w1106]
                          tunnel: w1101 -> [w1105]
                          i -> [w1104]
                          stop <- w1109 stop-if-true
                          n460 = call "Set_Compliance_Slope_R2.vi"("Compliance Slope"=w1105, "DIO Ref Out"=w1106, "VISA resource name"=w1107, "Servo ID"=w1108) -> ()  [unwired: 6 in, 2 out]
                          n461 = Greater Or Equal?(x=w1104, y=w1110) -> (x >= y?=w1109:bool)
                        }
                      }
                    }
                  }
                }
                n462 = Increment(x=w1074) -> (x+1=w1069:u16)
              }
            }
          }
        }
      }
    }
    frame #2 {
      n463 = VISA Close(VISA resource name=w1112) -> ()  [unwired: 1 in, 1 out]
      n464 = call <vilib>:"Close.vi"("DIO Ref In"=w1111) -> ()  [unwired: 10 in, 1 out]
    }
  }
  n465 = while {
    stop <- FALSE stop-if-true
    n466 = call "Wait9"("Count(mSec)"=u32 1000) -> ()  [unwired: 1 out]
  }
  n467 = while {
    shift-right: [w1183] -> _
    shift-left: "Initial Main State - Left" -> [w1205]
    shift-right: [w1175] -> _
    shift-left: "Search Direction - in - L" -> [w1199]
    shift-right: [w1174] -> _
    shift-left: FALSE -> [w1198]
    shift-right: [w1177] -> _
    shift-left: w13 -> [w1176]
    shift-right: [w1178] -> _
    shift-left: w13 -> [w1192]
    shift-right: [w1179] -> _
    shift-left: w13 -> [w1197]
    shift-right: [w1180] -> _
    shift-left: w13 -> [w1191]
    shift-right: [w1181] -> _
    shift-left: w13 -> [w1190]
    shift-right: [w1127] -> _
    shift-left: "Search Direction - in - Right" -> [w1140]
    shift-right: [w1171] -> _
    shift-left: FALSE -> [w1138]
    shift-right: [w1172] -> _
    shift-left: w12 -> [w1129]
    shift-right: [w1126] -> _
    shift-left: w12 -> [w1128]
    shift-right: [w1125] -> _
    shift-left: w12 -> [w1135]
    shift-right: [w1124] -> _
    shift-left: w12 -> [w1137]
    shift-right: [w1123] -> _
    shift-left: w12 -> [w1136]
    shift-right: [w1115] -> _
    shift-left: "Initial Main State- Right" -> [w1152]
    shift-right: [w1167] -> _
    shift-left: 0 -> [w1169]
    shift-right: [w1119] -> _
    shift-left: 0 -> [w1144]
    shift-right: [w1166] -> _
    shift-left: "Initial Tracking State - Left" -> [w1168]
    shift-right: [w1121] -> _
    shift-left: "Initial Tracking State - Right" -> [w1150]
    shift-right: [w1120] -> _
    shift-left: "Initial Recovery State  - Right" -> [w1151]
    shift-right: [w1164] -> _
    shift-left: "Initial Recovery State - L" -> [w1165]
    stop <- FALSE stop-if-true
    w1159 = enum16{"Track", "Reactive Predict", ""}."Track" ("Initial Tracking State - Right")
    w1185 = T4."Tracking" ("Next Main State")
    # "Wait for New"
    # "ADD TRACKING TIMEOUT COUNT**********************"
    # "Service Track Angle Flag"
    # "Add Logic to Have Search Directions\nopposite if Both Searching"
    # "REMOVE LAST GOAL POSITION WITH cURRENT"
    # "Go to Current State"
    # "Add Logic to Have Search Directions\nopposite if Both Searching"
    # "Manuallly Reset\nRespond Var"
    # "Manuallly Reset\nRespond Var"
    # "Update Comm Process Variables"
    # "Both  inTracking (main state)"
    # "Current delta - L"
    # "delta move sum - R"
    # "delta move sum - L"
    # "Current delta - R"
    # "Service Move Respond Variables"
    n468 = local read "Min Num Frames\nper Search"() -> (w1173:i32)
    n469 = local read "Minimum Delta \nServo Threshold"() -> (w1189:i16)
    n470 = local read "Maximum Move \nServo Threshold"() -> (w1188:i16)
    n471 = local read "Middle Beacon\nCoordinates"() -> (w1130:cluster{"X":sgl, "Y":sgl})
    n472 = local read "Position \nLock Status"() -> (w1196:bool)
    n473 = local read "Position \nLock Status"() -> (w1133:bool)
    n474 = local read "Search Step Size"() -> (w1187:u16)
    n475 = local read "Last Orientation"() -> (w1194:sgl)
    n476 = local read "Last Orientation"() -> (w1131:sgl)
    n477 = local read "Last Position"() -> (w1195:cluster{"X":sgl, "Y":sgl})
    n478 = local read "Last Position"() -> (w1132:cluster{"X":sgl, "Y":sgl})
    n479 = local read "Min Num Frames\nper Search"() -> (w1134:i32)
    n480 = call "Wait"("Count(mSec)"="Servo Algorithm\nCycle Time(ms)") -> ()  [unwired: 1 out]
    n481 = local read "Minimum Delta \nServo Threshold"() -> (w1142:i16)
    n482 = local read "Maximum Move \nServo Threshold"() -> (w1141:i16)
    n483 = local read "Search Step Size"() -> (w1139:u16)
    n484 = local read "New Data  Flag\nRight Servo"() -> (w1147:bool)
    n485 = local read "New Data  Flag\nLeft Servo"() -> (w1163:bool)
    n486 = local read "Image Lock - Right"() -> (w1149:bool)
    n487 = local read "Image Lock - Left"() -> (w1204:bool)
    n488 = local read "Tracking Angle - Right"() -> (w1146:sgl)
    n489 = local read "Tracking Angle - Left"() -> (w1202:sgl)
    n490 = local read "Current R (10bit)"() -> (w1145:u16)
    n491 = local read "Current L (10bit)"() -> (w1201:u16)
    n492 = case shown="True" w1163 {
      tunnel: [w1734 w1772] -> w1207
      tunnel: [w1728 w1771] -> w1206
      tunnel: w1205 -> [w1729 w1770]
      tunnel: w1204 -> [_ w1769]
      tunnel: "Track Angle Valid - Left" -> [_ w1768]
      tunnel: w1202 -> [_ w1767]
      tunnel: w1201 -> [w1734 w1766]
      tunnel: "Mounting Offset - Left" -> [_ w1765]
      tunnel: w1199 -> [w1725 w1764]
      tunnel: w1198 -> [_ w1763]
      tunnel: w1197 -> [w1726 w1762]
      tunnel: w1196 -> [_ w1761]
      tunnel: w1195 -> [_ w1760]
      tunnel: w1194 -> [_ w1759]
      tunnel: "Middle Beacon\nCoordinates" -> [_ w1758]
      tunnel: w1192 -> [w1724 w1757]
      tunnel: w1191 -> [w1723 w1756]
      tunnel: w1190 -> [w1727 w1755]
      tunnel: w1189 -> [_ w1754]
      tunnel: w1188 -> [_ w1753]
      tunnel: w1187 -> [_ w1752]
      tunnel: [0 w1751] -> w1184
      tunnel: [w1729 w1750] -> w1183
      tunnel: [w1728 w1749] -> w1182
      tunnel: [w1727 w1748] -> w1181
      tunnel: [w1723 w1747] -> w1180
      tunnel: [w1726 w1746] -> w1179
      tunnel: [w1724 w1745] -> w1178
      tunnel: w1176 -> [_ w1744]
      tunnel: [w1725 w1743] -> w1175
      tunnel: w1173 -> [_ w1742]
      tunnel: w1169 -> [w1732 w1741]
      tunnel: w1168 -> [w1731 w1740]
      tunnel: [w1732 w1739] -> w1167
      tunnel: [w1731 w1738] -> w1166
      tunnel: w1165 -> [w1730 w1737]
      tunnel: [w1730 w1736] -> w1164
      frame False {
        w1728 = FALSE
        # "Recovery Mode COunt"
        # "Frames Processed - L"
        # "Recovery Search move Count - L"
        # "Recovery Search Attempt Count- L"
        # "WAITING FOR NEW IMAGE, RETAIN ALL VALUES"
      }
      frame True {
        w1774 = u16 1023
        w1777 = u16 0
        # "New Tracking State"
        # "Tracking Timeout Count"
        # "Next Main State"
        # "Next Recovery State"
        # "Reset Respond"
        # "Search Direction"
        # "Recovery Count"
        # "Recovery Search move Count"
        # "Recovery Search Attempt Count"
        # "Frames Processed"
        # "Apply Floor/Ceiling to Goal Position"
        # "Current move Delta"
        # "Service Track Angle Flag"
        # "Move Servo"
        # "Goal Position"
        # "Go to Current State"
        n493 = case shown="\"Start Up Search\", Default" w1770 {
          tunnel: w1766 -> [w1795 w1871 w2050]
          tunnel: w1767 -> [_ w1873 _]
          tunnel: w1752 -> [w1794 _ w2045]
          tunnel: w1764 -> [w1793 w1854 w2039]
          tunnel: [w1792 w1869 w2049] -> w1778
          tunnel: [w1790 w1870 w2048] -> w1771
          tunnel: w1768 -> [_ w1864 w2026]
          tunnel: [w1788 w1866 w2035] -> w1750
          tunnel: w1769 -> [w1779 w1865 w2024]
          tunnel: w1765 -> [_ w1874 w2046]
          tunnel: w1754 -> [_ w1872 _]
          tunnel: [w1782 w1868 w2030] -> w1751
          tunnel: w1753 -> [_ w1867 _]
          tunnel: w1762 -> [w1787 _ w2040]
          tunnel: [enum16{"Generic Sweep", "Recovery Search"}."Recovery Search" enum16{"Generic Sweep", "Recovery Search"}."Recovery Search" w2047] -> w1736
          tunnel: w1757 -> [_ _ w2044]
          tunnel: w1737 -> [_ _ w2027]
          tunnel: w1763 -> [_ w1851 w2056]
          tunnel: w1744 -> [_ w1847 w2051]
          tunnel: w1759 -> [_ w1857 w2053]
          tunnel: w1760 -> [_ w1858 w2054]
          tunnel: w1761 -> [_ w1859 w2055]
          tunnel: w1758 -> [_ w1856 w2052]
          tunnel: [FALSE w1853 w2028] -> w1749
          tunnel: w1742 -> [w1786 _ w2038]
          tunnel: [w1782 w1848 w2037] -> w1745
          tunnel: [w1782 w1848 w2043] -> w1748
          tunnel: [w1782 w1848 w2042] -> w1747
          tunnel: [w1785 w1849 w2041] -> w1746
          tunnel: w1756 -> [_ _ w2033]
          tunnel: w1755 -> [_ _ w2032]
          tunnel: [w1783 w1854 w2031] -> w1743
          tunnel: w1741 -> [_ w1863 _]
          tunnel: [w1782 w1855 w2030] -> w1739
          tunnel: w1740 -> [_ w1860 _]
          tunnel: [enum16{"Track", "Reactive Predict", ""}."Track" ("Initial Tracking State - Right") w1852 enum16{"Track", "Reactive Predict", ""}."Track" ("Initial Tracking State - Right")] -> w1738
          frame "Start Up Search", Default {
            w1782 = u16 0
            # "Image Lock"
            # "Search Direction"
            # "Wait for 'x' Images to be Processed\nBefore Going to Next Step"
            # "Next Main State"
            # "New Goal Position"
            # "Move Servo"
            # "Choose Next State"
            # "Frames Processed Count"
            n494 = Greater Or Equal?(x=w1787, y=w1786) -> (x >= y?=w1791:bool)
            n495 = case shown="True" w1791 {
              tunnel: w1795 -> [w1805 w1821]
              tunnel: w1794 -> [_ w1819]
              tunnel: w1793 -> [w1804 w1818]
              tunnel: [w1805 w1811] -> w1792
              tunnel: [w1803 0] -> w1785
              tunnel: [FALSE TRUE] -> w1789
              tunnel: w1787 -> [w1806 _]
              tunnel: [w1804 w1812] -> w1783
              frame False {
                # "Wait until Min Number of Frames (per search/step) Processed"
                # "Increase Frames\nProcessed Count"
                n496 = Increment(x=w1806) -> (x+1=w1803:i32)
              }
              frame True {
                # "Reset Frames\nProcessed Count"
                # "SWEEP SEARCH - Startup"
                # "Multiple New Step\nby Step SIze"
                # "F = CCW\nT = CW"
                # "Last Direction"
                # "Min Step"
                # "add in case\nactual position\nis lower than GP"
                # "Set New Step #"
                # "Choose Direction"
                # "Nearest step"
                # "Adjust Actual Posiiton\n to pre-determiend steps"
                # "Move Servo 1 \"Step\" to\nSearch"
                n497 = Subtract(x=w1821, y=u16 200) -> (x-y=w1809:u16)
                n498 = Add(x=10, y=w1809) -> (x+y=w1827:i32)
                n499 = Quotient & Remainder(x=w1827, y=w1819) -> (floor(x/y)=w1825:i32)  [unwired: 1 out]
                n500 = To Byte Integer(number=w1825) -> (8bit integer=w1816:i8)
                n501 = Less?(x=w1816, y=1) -> (x < y?=w1822:bool)
                n502 = case shown="False" w1822 {
                  tunnel: w1816 -> [w1838 w1846]
                  tunnel: [w1840 FALSE] -> w1812
                  tunnel: [w1839 w1846] -> w1824
                  tunnel: w1818 -> [w1837 _]
                  tunnel: w1819 -> [w1835 _]
                  frame False {
                    # "Max Step"
                    # "# of steps\nminus 1"
                    n503 = Divide(x=300, y=w1835) -> (x/y=w1832:dbl)
                    n504 = To Unsigned Byte Integer(number=w1832) -> (unsigned 8bit integer=w1833:u8)
                    n505 = Greater Or Equal?(x=w1838, y=w1833) -> (x >= y?=w1834:bool)
                    n506 = case shown="True" w1834 {
                      tunnel: [w1841 TRUE] -> w1840
                      tunnel: [w1842 w1843] -> w1839
                      tunnel: w1838 -> [w1842 w1843]
                      tunnel: w1837 -> [w1841 _]
                      frame False {
                        # "No Need to\nChange Direction"
                      }
                      frame True {
                        # "T"
                        # "Move CW"
                      }
                    }
                  }
                  frame True {
                    # "F"
                    # "Move CCW"
                  }
                }
                n507 = case shown="False" w1812 {
                  tunnel: w1824 -> [w1829 w1830]
                  tunnel: [w1828 w1831] -> w1820
                  frame False {
                    # "CCW\n+1"
                    n508 = Increment(x=w1829) -> (x+1=w1828:i8)
                  }
                  frame True {
                    # "CW\n-1"
                    n509 = Decrement(x=w1830) -> (x-1=w1831:i8)
                  }
                }
                n510 = Multiply(x=w1820, y=w1819) -> (x*y=w1817:u16)
                n511 = To Unsigned Word Integer(number=w1817) -> (unsigned 16bit integer=w1815:u16)
                n512 = Add(x=w1815, y=u16 200) -> (x+y=w1811:u16)
              }
            }
            n513 = case shown="False" w1779 {
              tunnel: [w1797 FALSE] -> w1790
              tunnel: w1789 -> [w1797 _]
              tunnel: [w1798 T4."Tracking" ("Next Main State")] -> w1788
              frame False {
                # "Check other Servo\nStay in Startup  State"
                n514 = local read "Image Lock - Right"() -> (w1796:bool)
                n515 = case shown="False" w1796 {
                  tunnel: [T4."Start Up Search" ("Next Main State") T4."Recovery Mode" ("Next Main State")] -> w1798
                  frame False {
                  }
                  frame True {
                  }
                }
              }
              frame True {
                # "Override Move Servo\nCommand bc an Angle Was Found\nduring this Step"
                # "Transition to Tracking State When\nImage Processing has Locked"
              }
            }
          }
          frame "Tracking" {
            w1848 = 0
            # "Frames Processed Count"
            # "Image Lock - L"
            # "Track Angle Valid"
            # "Tracking Angle"
            # "Tracking Timeout Count"
            # "Max ove delta"
            # "Move delta threshold"
            # "mount offset"
            # "Current Position"
            # "Move Respond"
            # "Trackin Timeout count"
            # "Move Servo"
            # "delta"
            # "GP"
            # "Reset Move Respond"
            # "New Tracking State"
            # "Delta Move Sum"
            # "Choose Next State"
            n516 = case shown="\"Reactive Predict\"" w1860 {
              tunnel: w1874 -> [w1892 _]
              tunnel: w1873 -> [w1891 _]
              tunnel: w1872 -> [w1890 _]
              tunnel: w1871 -> [w1889 w1948]
              tunnel: [w1888 w1946] -> w1870
              tunnel: [w1887 w1954] -> w1869
              tunnel: [w1886 0] -> w1868
              tunnel: w1867 -> [w1885 _]
              tunnel: w1865 -> [w1884 w1938]
              tunnel: w1864 -> [w1883 w1941]
              tunnel: w1863 -> [w1882 w1943]
              tunnel: w1859 -> [_ w1953]
              tunnel: w1858 -> [_ w1952]
              tunnel: w1857 -> [_ w1951]
              tunnel: w1856 -> [_ w1950]
              tunnel: w1851 -> [_ w1949]
              tunnel: w1847 -> [_ w1947]
              tunnel: [TRUE w1944] -> w1853
              tunnel: [w1879 w1942] -> w1855
              tunnel: [w1877 w1940] -> w1852
              tunnel: [0 0] -> w1849
              frame "Track", Default {
                # "Reset"
                # "Tracking Timeout"
                # "Move Delta"
                # "Goal Position"
                # "Tracking Move"
                # "Move Servo"
                # "Only Consider Tracking Angle\n\nIF\n\nImage Locked        == T\nTrack Angle Flag   == T"
                n517 = And(x=w1884, y=w1883) -> (x .and. y?=w1876:bool)
                n518 = case shown="False" w1876 {
                  tunnel: w1892 -> [_ w1900]
                  tunnel: w1891 -> [_ w1917]
                  tunnel: w1890 -> [_ w1914]
                  tunnel: w1889 -> [w1895 w1904]
                  tunnel: [w1895 w1913] -> w1887
                  tunnel: [w1897 w1912] -> w1888
                  tunnel: [w1897 w1911] -> _
                  tunnel: [u16 0 w1910] -> w1886
                  tunnel: w1885 -> [_ w1906]
                  tunnel: w1882 -> [w1894 _]
                  tunnel: [w1893 0] -> w1879
                  frame False {
                    w1897 = FALSE
                    # "Increment timeout"
                    n519 = Increment(x=w1894) -> (x+1=w1893:i32)
                  }
                  frame True {
                    # "******"
                    # "Determine Direction of Move"
                    # "Convert Track Angle to UINT16"
                    # "1024/300"
                    # "Move to Tracking Angle \n\nif delta is greater than move servo threshold\nAND less than max move threshold"
                    n520 = Add(x=w1917, y=w1900) -> (x+y=w1920:sgl)
                    n521 = local read "Last Track Angle - L"() -> (w1899:sgl)
                    n522 = Add(x=w1920, y=sgl 60.0) -> (x+y=w1919:sgl)
                    n523 = Multiply(x=3.413333333333333, y=w1919) -> (x*y=w1898:dbl)
                    n524 = To Word Integer(number=w1904) -> (16bit integer=w1902:i16)
                    n525 = To Unsigned Word Integer(number=w1898) -> (unsigned 16bit integer=w1916:u16)
                    n526 = To Word Integer(number=w1898) -> (16bit integer=w1915:i16)
                    n527 = Subtract(x=w1898, y=w1899) -> ()  [unwired: 1 out]
                    n528 = Subtract(x=w1915, y=w1902) -> (x-y=w1905:i16)
                    n529 = Absolute Value(x=w1905) -> (abs(x)=w1901:i16)
                    n530 = Greater Or Equal?(x=w1901, y=w1914) -> (x >= y?=w1908:bool)
                    n531 = Less Or Equal?(x=w1901, y=w1906) -> (x <= y?=w1907:bool)
                    n532 = And(x=w1908, y=w1907) -> (x .and. y?=w1909:bool)
                    n533 = case shown="True" w1909 {
                      tunnel: w1916 -> [_ w1928]
                      tunnel: [w1923 w1928] -> w1913
                      tunnel: [w1924 w1934] -> w1912
                      tunnel: [w1924 w1934] -> w1911
                      tunnel: w1904 -> [w1923 _]
                      tunnel: w1901 -> [_ w1933]
                      tunnel: [u16 0 w1933] -> w1910
                      tunnel: w1900 -> [_ w1927]
                      frame False {
                        w1924 = FALSE
                        # "Don't Move"
                      }
                      frame True {
                        w1934 = TRUE
                        # "45 DEG MOUNT OFFSET"
                        # "1024/300"
                        # "Current Delta"
                        # "Use new Track Angle"
                        n534 = Divide(x=w1928, y=3.413333333333333) -> (x/y=w1930:dbl)
                        n535 = Negate(x=w1927) -> (-x=w1926:sgl)
                        n536 = Subtract(x=w1930, y=sgl 60.0) -> (x-y=w1932:dbl)
                        n537 = Add(x=w1932, y=w1926) -> (x+y=w1925:dbl)
                        n538 = local write "Last Track Angle - L"(w1925) -> ()
                      }
                    }
                  }
                }
                n539 = local read "Timeout to \nEnable Reactive Predict"() -> (w1880:u16)
                n540 = Less?(x=w1879, y=w1880) -> (x < y?=w1878:bool)
                n541 = case shown="True" w1878 {
                  tunnel: [enum16{"Track", "Reactive Predict", ""}."Reactive Predict" ("Initial Tracking State - Right") enum16{"Track", "Reactive Predict", ""}."Track" ("Initial Tracking State - Right")] -> w1877
                  frame False {
                  }
                  frame True {
                  }
                }
              }
              frame "Reactive Predict" {
                # "Choose New\nTracking State"
                n542 = Or(x=w1938, y=w1941) -> (x .or. y?=w1937:bool)
                n543 = case shown="False" w1937 {
                  tunnel: [w1967 w2020] -> w1954
                  tunnel: w1953 -> [w1966 _]
                  tunnel: w1952 -> [w1965 _]
                  tunnel: w1951 -> [w1964 _]
                  tunnel: w1950 -> [w1963 _]
                  tunnel: w1949 -> [w1962 _]
                  tunnel: w1947 -> [w1961 _]
                  tunnel: [w1960 FALSE] -> w1946
                  tunnel: [w1959 TRUE] -> w1944
                  tunnel: w1943 -> [w1958 _]
                  tunnel: [w1957 0] -> w1942
                  tunnel: [enum16{"Track", "Reactive Predict", ""}."Reactive Predict" ("Initial Tracking State - Right") enum16{"Track", "Reactive Predict", ""}."Track" ("Initial Tracking State - Right")] -> w1940
                  tunnel: w1948 -> [w1955 w2020]
                  frame False {
                    # "Stay in Reactive State"
                    # "Increment Track Timeout"
                    # "Move Respond Flag"
                    n544 = Increment(x=w1958) -> (x+1=w1957:i32)
                    n545 = case shown="False" w1962 {
                      tunnel: w1966 -> [_ w1982]
                      tunnel: w1965 -> [_ w1981]
                      tunnel: w1964 -> [_ w1980]
                      tunnel: w1963 -> [_ w1979]
                      tunnel: w1961 -> [_ w1976]
                      tunnel: [w1968 w1972] -> w1967
                      tunnel: [w1969 w1971] -> w1960
                      tunnel: [w1969 w1971] -> w1959
                      tunnel: w1955 -> [w1968 w1970]
                      frame False {
                        w1969 = FALSE
                        # "Reset Move Respond = F"
                        # "Move Servo = F"
                      }
                      frame True {
                        w1971 = TRUE
                        # "Position Lock"
                        # "Current Servo\nPosition"
                        # "Reset Move\nRespond = T"
                        # "Move Servo = T"
                        # "Apply Direction \nto Offset (delta sum)"
                        # "Check Last Known Position of Robot"
                        n546 = case shown="True" w1982 {
                          tunnel: w1981 -> [_ w2010]
                          tunnel: w1980 -> [_ w1985]
                          tunnel: w1979 -> [_ w1986]
                          tunnel: [sgl 1.0 ("y") w1984] -> w1978
                          frame False {
                            # "No Position Data Available"
                            # "Default is to move\nSame Direction as other\nServo"
                          }
                          frame True {
                            w1991 = sgl 1.0 ("y")
                            # "Use previous position/orientation to Guess Which Direction to Move Servo"
                            # "Choose Search Direction"
                            # "\"Perpendicular \nThreshold\""
                            # "If Orientation is\n ~Perpendicular -> Start Search\n in Opposite Direction of Other"
                            # "****add 90 until orientation angle is fixed"
                            # "Last Orientation"
                            # "Convert to Rad"
                            # "Avoid Divide by 0"
                            # "-1/m"
                            # "Calculate Normal Line to \nLast Robot Position\nfrom Center Beacon"
                            # "last Position \nCoordinates"
                            n547 = Unbundle(w2010) -> ("X"=w1990:sgl, "Y"=w1989:sgl)
                            n548 = Unbundle(w1986) -> ("X"=w1988:sgl, "Y"=w1987:sgl)
                            n549 = Subtract(x=w1989, y=w1987) -> (x-y=w2006:sgl)
                            n550 = Subtract(x=w1990, y=w1988) -> (x-y=w2004:sgl)
                            n551 = Equal To 0?(x=w2004) -> (x = 0?=w2005:bool)
                            n552 = case shown="False" w2005 {
                              tunnel: w2006 -> [w2013 _]
                              tunnel: w2004 -> [w2012 _]
                              tunnel: [w2011 1000000000000000.0] -> w2003
                              frame False {
                                n553 = Divide(x=w2013, y=w2012) -> (x/y=w2011:sgl)
                              }
                              frame True {
                              }
                            }
                            n554 = Equal To 0?(x=w2003) -> (x = 0?=w2008:bool)
                            n555 = case shown="False" w2008 {
                              tunnel: [w2015 1e-08] -> w2007
                              tunnel: w2003 -> [w2015 _]
                              frame False {
                              }
                              frame True {
                                # "Can't have infinit slope"
                              }
                            }
                            n556 = Divide(x=-1.0, y=w2007) -> (x/y=w2002:dbl)
                            n557 = Inverse Tangent(1:w2002) -> (0:w2000:dbl)
                            n558 = expression code="(x/pi)*180.0" "radians to degrees"(w2000) -> (w2001:dbl)
                            n559 = To Single Precision Float(number=w2001) -> (single precision float=w1998:sgl)
                            n560 = Add(x=w1985, y=sgl 90.0) -> (x+y=w1997:sgl)
                            n561 = Subtract(x=w1998, y=w1997) -> (x-y=w1996:sgl)
                            n562 = Absolute Value(x=w1996) -> (abs(x)=w1995:sgl)
                            n563 = Less Or Equal?(x=w1995, y=sgl 10.0) -> (x <= y?=w1993:bool)
                            n564 = Negate(x=w1991) -> (-x=w1992:sgl)
                            n565 = Select(t=w1992, s=w1993, f=w1991) -> (s? t:f=w1984:sgl)
                          }
                        }
                        n566 = To Word Integer(number=w1978) -> (16bit integer=w1977:i16)
                        n567 = Multiply(x=w1977, y=w1976) -> (x*y=w1975:i32)
                        n568 = To Word Integer(number=w1970) -> (16bit integer=w1974:i16)
                        n569 = Add(x=w1975, y=w1974) -> (x+y=w1973:i32)
                        n570 = To Unsigned Word Integer(number=w1973) -> (unsigned 16bit integer=w1972:u16)
                      }
                    }
                  }
                  frame True {
                    # "Either Current Angle Valid or Image Lock Acheived"
                    # "Go Directly to Track State"
                  }
                }
              }
            }
            n571 = local read "Tracking Timeout\nThreshold"() -> (w1861:i32)
            n572 = Less?(x=w1855, y=w1861) -> (x < y?=w1862:bool)
            n573 = case shown="True" w1862 {
              tunnel: [T4."Recovery Mode" ("Next Main State") T4."Tracking" ("Next Main State")] -> w1866
              frame False {
              }
              frame True {
              }
            }
          }
          frame "Recovery Mode" {
            w2030 = u16 0
            # "Recovery Search Move Count"
            # "***Compltetly resets as of R17, used to just reset to \"Max Recovery Count - 1\""
            # "Increment Recoveyr Mode Count"
            # "Frames Processed"
            # "Choose Next Main State"
            # "Reset recovery count"
            # "Recovery move\nCount"
            # "Recovery Search\nAttempt count"
            # "Move Servo = T"
            # "delta move sum"
            # "Robot Position Valid"
            n574 = local read "Image Lock - Right"() -> (w2034:bool)
            n575 = case shown="\"Recovery Search\"" w2027 {
              tunnel: w2056 -> [_ _]
              tunnel: w2055 -> [_ _]
              tunnel: w2054 -> [_ _]
              tunnel: w2053 -> [_ _]
              tunnel: w2052 -> [_ _]
              tunnel: w2051 -> [_ _]
              tunnel: w2050 -> [w2084 w2170]
              tunnel: [w2076 w2168] -> w2049
              tunnel: [w2073 w2162] -> w2048
              tunnel: [FALSE FALSE] -> w2028
              tunnel: [w2078 w2160] -> w2047
              tunnel: w2044 -> [w2082 _]
              tunnel: w2046 -> [w2085 _]
              tunnel: w2045 -> [w2083 w2165]
              tunnel: [w2075 w2159] -> w2042
              tunnel: [w2074 w2159] -> w2043
              tunnel: w2034 -> [w2072 _]
              tunnel: [w2063 w2169] -> w2041
              tunnel: w2040 -> [w2061 w2157]
              tunnel: w2039 -> [w2066 w2166]
              tunnel: w2038 -> [w2062 w2164]
              tunnel: w2024 -> [_ _]
              tunnel: w2026 -> [_ _]
              tunnel: [FALSE w2161] -> w2036
              tunnel: w2033 -> [w2070 _]
              tunnel: w2032 -> [w2069 _]
              tunnel: [w2066 w2158] -> w2031
              tunnel: w2024 -> [_ w2155]
              frame "Recovery Search" {
                # "Wait for 2 Images to be Processed\nBefore Going to Next Step"
                # "Choose Next Reovery State"
                # "Recovery Search \nAttempt Count"
                # "Move Servo"
                # "Goal Position"
                # "Recovery Search\nmove Count"
                # "Attempt Recovery Search if Other Servo has Valid Angle"
                n576 = local read "Last Track Angle - R"() -> (w2065:sgl)
                n577 = Greater Or Equal?(x=w2061, y=w2062) -> (x >= y?=w2064:bool)
                n578 = case shown="True" w2064 {
                  tunnel: w2085 -> [_ w2105]
                  tunnel: [w2090 w2104] -> w2074
                  tunnel: w2084 -> [w2093 w2103]
                  tunnel: w2083 -> [_ w2102]
                  tunnel: [w2091 w2101] -> w2075
                  tunnel: [w2093 w2100] -> w2076
                  tunnel: [FALSE w2099] -> w2073
                  tunnel: w2070 -> [w2091 w2098]
                  tunnel: w2069 -> [w2090 w2097]
                  tunnel: w2072 -> [_ w2096]
                  tunnel: w2065 -> [_ w2095]
                  tunnel: [w2088 0 ("Frames Processed\nCount - in")] -> w2063
                  tunnel: w2061 -> [w2089 _]
                  frame False {
                    # "Increment Frames Processed"
                    # "WAIT"
                    n579 = Increment(x=w2089) -> (x+1=w2088:i32)
                  }
                  frame True {
                    n580 = case shown="True" w2096 {
                      tunnel: w2095 -> [_ w2118]
                      tunnel: w2098 -> [w2106 w2114]
                      tunnel: w2105 -> [_ w2119]
                      tunnel: [w2109 w2117] -> w2100
                      tunnel: [w2107 w2116] -> w2104
                      tunnel: w2097 -> [w2107 w2115]
                      tunnel: w2103 -> [w2109 w2113]
                      tunnel: w2102 -> [_ w2112]
                      tunnel: [FALSE TRUE] -> w2099
                      tunnel: [w2106 w2110] -> w2101
                      frame False {
                        # "Don't Move bc Other Servo Doesn't Have Image Lock"
                      }
                      frame True {
                        # "Move Servo = T"
                        n581 = Greater Than 0?(x=w2114) -> (x > 0?=w2120:bool)
                        n582 = case shown="False" w2120 {
                          tunnel: w2119 -> [w2129 _]
                          tunnel: w2118 -> [w2124 _]
                          tunnel: [w2121 w2139] -> w2117
                          tunnel: [w2127 w2145] -> w2116
                          tunnel: w2115 -> [w2128 w2145]
                          tunnel: w2114 -> [w2126 w2142]
                          tunnel: [w2125 w2144] -> w2110
                          tunnel: w2113 -> [_ w2140]
                          tunnel: w2112 -> [_ w2137]
                          frame False {
                            # "************************"
                            # "Increment move count to transition\nto Pan mode"
                            # "Increment Recovery Search Attempt Count"
                            # "1024/300"
                            # "Move Parallel to Other Servo"
                            n583 = Increment(x=w2128) -> (x+1=w2127:i32)
                            n584 = Add(x=w2124, y=w2129) -> (x+y=w2135:sgl)
                            n585 = Add(x=w2135, y=sgl 60.0) -> (x+y=w2134:sgl)
                            n586 = Multiply(x=3.413333333333333, y=w2134) -> (x*y=w2132:dbl)
                            n587 = Add(x=0.5, y=w2132) -> (x+y=w2130:dbl)
                            n588 = To Unsigned Word Integer(number=w2130) -> (unsigned 16bit integer=w2122:u16)
                            n589 = Increment(x=w2126) -> (x+1=w2125:i32)
                            n590 = Add(x=w2122, y="Recovery Parallel\nSearch Offset") -> (x+y=w2121:u16)
                          }
                          frame True {
                            # "Apply Direction"
                            # "Step SIze"
                            # "Current Position"
                            # "Attempt to Pan in Steps Towards other Servo"
                            # "Could be same or function of \nregular search step size"
                            # "Max # of Pan\nMoves"
                            # "Pan Towards Other Servo"
                            n591 = Greater Or Equal?(x=w2142, y="Max # Pan Moves") -> (x >= y?=w2143:bool)
                            n592 = case shown="False" w2143 {
                              tunnel: w2142 -> [w2153 _]
                              tunnel: [w2152 u16 0] -> w2144
                              frame False {
                                # "Increment Pan Count"
                                n593 = Increment(x=w2153) -> (x+1=w2152:i32)
                              }
                              frame True {
                                # "Reset move count"
                              }
                            }
                            n594 = local read "Recovery Search\nDirection - L"() -> (w2138:bool)
                            n595 = case shown="True" w2138 {
                              tunnel: w2140 -> [w2147 w2151]
                              tunnel: w2137 -> [w2148 w2150]
                              tunnel: [w2146 w2149] -> w2139
                              frame False {
                                # "CCW"
                                n596 = Add(x=w2147, y=w2148) -> (x+y=w2146:u16)
                              }
                              frame True {
                                # "CW"
                                n597 = Subtract(x=w2151, y=w2150) -> (x-y=w2149:u16)
                              }
                            }
                          }
                        }
                      }
                    }
                  }
                }
                n598 = local read "Max Recovery Count\n(Recovery Search)"() -> (w2067:u16)
                n599 = local read "Max Recovery\nSearch Attempts"() -> (w2068:u16)
                n600 = Less Or Equal?(x=w2074, y=w2068) -> (x <= y?=w2080:bool)
                n601 = Less Or Equal?(x=w2082, y=w2067) -> (x <= y?=w2081:bool)
                n602 = And(x=w2080, y=w2081) -> (x .and. y?=w2079:bool)
                n603 = case shown="True" w2079 {
                  tunnel: [enum16{"Generic Sweep", "Recovery Search"}."Generic Sweep" enum16{"Generic Sweep", "Recovery Search"}."Recovery Search"] -> w2078
                  frame False {
                  }
                  frame True {
                  }
                }
              }
              frame "Generic Sweep" {
                w2159 = u16 0
                # "Image Locked?"
                # "Choose Next Recovery State"
                # "Wait for 2 Images to be Processed\nBefore Going to Next Step"
                # "New Goal Position"
                # "Move Servo"
                # "Frames Processed Count"
                n604 = Greater Or Equal?(x=w2157, y=w2164) -> (x >= y?=w2171:bool)
                n605 = case shown="True" w2171 {
                  tunnel: w2170 -> [w2187 w2199]
                  tunnel: w2165 -> [_ w2197]
                  tunnel: w2166 -> [w2186 w2196]
                  tunnel: [w2187 w2193] -> w2168
                  tunnel: [w2185 0] -> w2169
                  tunnel: [FALSE TRUE] -> w2163
                  tunnel: w2157 -> [w2188 _]
                  tunnel: [w2186 w2190] -> w2158
                  frame False {
                    # "Increment Frames Processed"
                    n606 = Increment(x=w2188) -> (x+1=w2185:i32)
                  }
                  frame True {
                    # "Reset Frames\nProcessed Count"
                    # "SWEEP SEARCH - Startup"
                    # "Multiple New Step\nby Step SIze"
                    # "F = CCW\nT = CW"
                    # "Last Direction"
                    # "Min Step"
                    # "add 10 in case\nactual position\nis lower than GP"
                    # "Set New Step #"
                    # "Choose Direction"
                    # "Nearest step"
                    # "Adjust Actual Posiiton\n to pre-determiend steps"
                    # "Move Servo 1 \"Step\" to\nSearch"
                    n607 = Add(x=5, y=w2199) -> (x+y=w2205:i32)
                    n608 = Quotient & Remainder(x=w2205, y=w2197) -> (floor(x/y)=w2203:i32)  [unwired: 1 out]
                    n609 = To Byte Integer(number=w2203) -> (8bit integer=w2194:i8)
                    n610 = Less?(x=w2194, y=1) -> (x < y?=w2200:bool)
                    n611 = case shown="False" w2200 {
                      tunnel: w2194 -> [w2216 w2224]
                      tunnel: [w2218 FALSE] -> w2190
                      tunnel: [w2217 w2224] -> w2202
                      tunnel: w2196 -> [w2215 _]
                      tunnel: w2197 -> [w2213 _]
                      frame False {
                        # "Max Step"
                        # "# of steps\nminus 1"
                        n612 = Divide(x=1024, y=w2213) -> (x/y=w2210:dbl)
                        n613 = To Unsigned Byte Integer(number=w2210) -> (unsigned 8bit integer=w2211:u8)
                        n614 = Greater Or Equal?(x=w2216, y=w2211) -> (x >= y?=w2212:bool)
                        n615 = case shown="True" w2212 {
                          tunnel: [w2219 TRUE] -> w2218
                          tunnel: [w2220 w2221] -> w2217
                          tunnel: w2216 -> [w2220 w2221]
                          tunnel: w2215 -> [w2219 _]
                          frame False {
                            # "No Need to\nChange Direction"
                          }
                          frame True {
                            # "T"
                            # "Move CW"
                          }
                        }
                      }
                      frame True {
                        # "F"
                        # "Move CCW"
                      }
                    }
                    n616 = case shown="True" w2190 {
                      tunnel: w2202 -> [w2207 w2208]
                      tunnel: [w2206 w2209] -> w2198
                      frame False {
                        # "CCW\n+1"
                        n617 = Increment(x=w2207) -> (x+1=w2206:i8)
                      }
                      frame True {
                        # "CW\n-1"
                        n618 = Decrement(x=w2208) -> (x-1=w2209:i8)
                      }
                    }
                    n619 = Multiply(x=w2198, y=w2197) -> (x*y=w2195:u16)
                    n620 = To Unsigned Word Integer(number=w2195) -> (unsigned 16bit integer=w2193:u16)
                  }
                }
                n621 = local read "Image Lock - Right"() -> (w2156:bool)
                n622 = case shown="True" w2155 {
                  tunnel: [w2174 w2184] -> w2162
                  tunnel: w2163 -> [w2175 _]
                  tunnel: [w2176 enum16{"Generic Sweep", "Recovery Search"}."Generic Sweep"] -> w2160
                  tunnel: [w2173 w2184] -> w2161
                  tunnel: w2156 -> [w2172 _]
                  frame False {
                    # "Is other servo tracking?"
                    n623 = case shown="True" w2172 {
                      tunnel: [enum16{"Generic Sweep", "Recovery Search"}."Generic Sweep" enum16{"Generic Sweep", "Recovery Search"}."Recovery Search"] -> w2176
                      tunnel: w2175 -> [w2179 _]
                      tunnel: [w2179 FALSE] -> w2174
                      tunnel: [FALSE TRUE] -> w2173
                      frame False {
                        # "Stay in Sweep"
                      }
                      frame True {
                        # "G o to Recovery Search  State"
                      }
                    }
                  }
                  frame True {
                    w2184 = FALSE
                    # "Override Move Servo\nCommand bc an Angle Was Found\nduring this Step"
                    # "Stay In Sweep\nLet Main State Machine transition\ninto Tracking"
                  }
                }
              }
            }
            n624 = Increment(x=w2044) -> (x+1=w2025:i32)
            n625 = case shown="False" w2036 {
              tunnel: w2025 -> [w2059 _]
              tunnel: [w2059 0] -> w2037
              frame False {
              }
              frame True {
              }
            }
            n626 = case shown="False" w2024 {
              tunnel: [T4."Recovery Mode" ("Next Main State") T4."Tracking" ("Next Main State")] -> w2035
              frame False {
              }
              frame True {
              }
            }
          }
        }
        "Current Move Delta - L" <- w1751
        n627 = Less?(x=w1778, y=w1777) -> (x < y?=w1776:bool)
        n628 = local write "New Data  Flag\nLeft Servo"(FALSE) -> ()
        n629 = Select(t=w1777, s=w1776, f=w1778) -> (s? t:f=w1773:u16)
        n630 = Greater?(x=w1773, y=w1774) -> (0:w1775:bool)
        n631 = Select(t=w1774, s=w1775, f=w1773) -> (s? t:f=w1772:u16)
      }
    }
    "Next Main State - Left" <- w1183
    "Next Tracking State - Left" <- w1166
    "Next Recovery State - Left" <- w1164
    n632 = case shown="True" w1147 {
      tunnel: [w1232 w1270] -> w1117
      tunnel: [w1226 w1269] -> w1116
      tunnel: w1152 -> [w1227 w1268]
      tunnel: w1149 -> [_ w1267]
      tunnel: "Track Angle Valid  - Right" -> [_ w1266]
      tunnel: w1146 -> [_ w1265]
      tunnel: w1145 -> [w1232 w1264]
      tunnel: "Mounting Offset - Right" -> [_ w1263]
      tunnel: w1140 -> [w1223 w1262]
      tunnel: w1138 -> [_ w1261]
      tunnel: w1135 -> [w1224 w1260]
      tunnel: w1133 -> [_ w1259]
      tunnel: w1132 -> [_ w1258]
      tunnel: w1131 -> [_ w1257]
      tunnel: w1130 -> [_ w1256]
      tunnel: w1128 -> [w1222 w1255]
      tunnel: w1137 -> [w1221 w1254]
      tunnel: w1136 -> [w1225 w1253]
      tunnel: w1142 -> [_ w1252]
      tunnel: w1141 -> [_ w1251]
      tunnel: w1139 -> [_ w1250]
      tunnel: [0 w1249] -> w1118
      tunnel: [w1227 w1248] -> w1115
      tunnel: [w1226 w1247] -> w1122
      tunnel: [w1225 w1246] -> w1123
      tunnel: [w1221 w1245] -> w1124
      tunnel: [w1224 w1244] -> w1125
      tunnel: [w1222 w1243] -> w1126
      tunnel: w1129 -> [_ w1242]
      tunnel: [w1223 w1241] -> w1127
      tunnel: w1134 -> [_ w1240]
      tunnel: w1144 -> [w1230 w1239]
      tunnel: w1150 -> [w1229 w1238]
      tunnel: [w1230 w1237] -> w1119
      tunnel: [w1229 w1236] -> w1121
      tunnel: w1151 -> [w1228 w1235]
      tunnel: [w1228 w1234] -> w1120
      frame False {
        w1226 = FALSE
        # "Recovery Mode COunt"
        # "Frames Processed - L"
        # "Recovery Search move Count - L"
        # "Recovery Search Attempt Count- L"
        # "WAITING FOR NEW IMAGE, RETAIN ALL VALUES"
      }
      frame True {
        w1272 = u16 1023
        w1275 = u16 0
        # "New Tracking State"
        # "Tracking Timeout Count"
        # "Next Main State"
        # "Next Recovery State"
        # "Reset Respond"
        # "Search Direction"
        # "Recovery Count"
        # "Recovery Search move Count"
        # "Recovery Search Attempt Count"
        # "Frames Processed"
        # "Apply Floor/Ceiling to Goal Position"
        # "Current move Delta"
        # "Service Track Angle Flag"
        # "Move Servo"
        # "Goal Position"
        # "Go to Current State"
        n633 = case shown="\"Recovery Mode\"" w1268 {
          tunnel: w1264 -> [w1293 w1365 w1544]
          tunnel: w1265 -> [_ w1367 _]
          tunnel: w1250 -> [w1292 _ w1539]
          tunnel: w1262 -> [w1291 w1348 w1533]
          tunnel: [w1290 w1363 w1543] -> w1276
          tunnel: [w1288 w1364 w1542] -> w1269
          tunnel: w1266 -> [_ w1358 w1520]
          tunnel: [w1286 w1360 w1529] -> w1248
          tunnel: w1267 -> [w1277 w1359 w1518]
          tunnel: w1263 -> [_ w1368 w1540]
          tunnel: w1252 -> [_ w1366 _]
          tunnel: [w1280 w1362 w1524] -> w1249
          tunnel: w1251 -> [_ w1361 _]
          tunnel: w1260 -> [w1285 _ w1534]
          tunnel: [enum16{"Generic Sweep", "Recovery Search"}."Recovery Search" enum16{"Generic Sweep", "Recovery Search"}."Recovery Search" w1541] -> w1234
          tunnel: w1255 -> [_ _ w1538]
          tunnel: w1235 -> [_ _ w1521]
          tunnel: w1261 -> [_ w1345 w1550]
          tunnel: w1242 -> [_ w1341 w1545]
          tunnel: w1257 -> [_ w1351 w1547]
          tunnel: w1258 -> [_ w1352 w1548]
          tunnel: w1259 -> [_ w1353 w1549]
          tunnel: w1256 -> [_ w1350 w1546]
          tunnel: [FALSE w1347 w1522] -> w1247
          tunnel: w1240 -> [w1284 _ w1532]
          tunnel: [w1280 w1342 w1531] -> w1243
          tunnel: [w1280 w1342 w1537] -> w1246
          tunnel: [w1280 w1342 w1536] -> w1245
          tunnel: [w1283 w1343 w1535] -> w1244
          tunnel: w1254 -> [_ _ w1527]
          tunnel: w1253 -> [_ _ w1526]
          tunnel: [w1281 w1348 w1525] -> w1241
          tunnel: w1239 -> [_ w1357 _]
          tunnel: [w1280 w1349 w1524] -> w1237
          tunnel: w1238 -> [_ w1354 _]
          tunnel: [enum16{"Track", "Reactive Predict", ""}."Track" ("Initial Tracking State - Right") w1346 enum16{"Track", "Reactive Predict", ""}."Track" ("Initial Tracking State - Right")] -> w1236
          frame "Start Up Search", Default {
            w1280 = u16 0
            # "Image Lock"
            # "Search Direction"
            # "Wait for 'x' Images to be Processed\nBefore Going to Next Step"
            # "Next Main State"
            # "New Goal Position"
            # "Move Servo"
            # "Choose Next State"
            # "Frames Processed Count"
            n634 = Greater Or Equal?(x=w1285, y=w1284) -> (x >= y?=w1289:bool)
            n635 = case shown="True" w1289 {
              tunnel: w1293 -> [w1303 w1315]
              tunnel: w1292 -> [_ w1313]
              tunnel: w1291 -> [w1302 w1312]
              tunnel: [w1303 w1309] -> w1290
              tunnel: [w1301 0] -> w1283
              tunnel: [FALSE TRUE] -> w1287
              tunnel: w1285 -> [w1304 _]
              tunnel: [w1302 w1306] -> w1281
              frame False {
                # "Wait until Min Number of Frames (per search/step) Processed"
                # "Increase Frames\nProcessed Count"
                n636 = Increment(x=w1304) -> (x+1=w1301:i32)
              }
              frame True {
                # "Reset Frames\nProcessed Count"
                # "SWEEP SEARCH - Startup"
                # "Multiple New Step\nby Step SIze"
                # "F = CCW\nT = CW"
                # "Last Direction"
                # "Min Step"
                # "add in case\nactual position\nis lower than GP"
                # "Set New Step #"
                # "Choose Direction"
                # "Nearest step"
                # "Adjust Actual Posiiton\n to pre-determiend steps"
                # "Move Servo 1 \"Step\" to\nSearch"
                n637 = Add(x=3, y=w1315) -> (x+y=w1321:i32)
                n638 = Quotient & Remainder(x=w1321, y=w1313) -> (floor(x/y)=w1319:i32)  [unwired: 1 out]
                n639 = To Byte Integer(number=w1319) -> (8bit integer=w1310:i8)
                n640 = Less?(x=w1310, y=1) -> (x < y?=w1316:bool)
                n641 = case shown="False" w1316 {
                  tunnel: w1310 -> [w1332 w1340]
                  tunnel: [w1334 FALSE] -> w1306
                  tunnel: [w1333 w1340] -> w1318
                  tunnel: w1312 -> [w1331 _]
                  tunnel: w1313 -> [w1329 _]
                  frame False {
                    # "Max Step"
                    # "# of steps\nminus 1"
                    n642 = Divide(x=1024, y=w1329) -> (x/y=w1326:dbl)
                    n643 = To Unsigned Byte Integer(number=w1326) -> (unsigned 8bit integer=w1327:u8)
                    n644 = Greater Or Equal?(x=w1332, y=w1327) -> (x >= y?=w1328:bool)
                    n645 = case shown="True" w1328 {
                      tunnel: [w1335 TRUE] -> w1334
                      tunnel: [w1336 w1337] -> w1333
                      tunnel: w1332 -> [w1336 w1337]
                      tunnel: w1331 -> [w1335 _]
                      frame False {
                        # "No Need to\nChange Direction"
                      }
                      frame True {
                        # "T"
                        # "Move CW"
                      }
                    }
                  }
                  frame True {
                    # "F"
                    # "Move CCW"
                  }
                }
                n646 = case shown="False" w1306 {
                  tunnel: w1318 -> [w1323 w1324]
                  tunnel: [w1322 w1325] -> w1314
                  frame False {
                    # "CCW\n+1"
                    n647 = Increment(x=w1323) -> (x+1=w1322:i8)
                  }
                  frame True {
                    # "CW\n-1"
                    n648 = Decrement(x=w1324) -> (x-1=w1325:i8)
                  }
                }
                n649 = Multiply(x=w1314, y=w1313) -> (x*y=w1311:u16)
                n650 = To Unsigned Word Integer(number=w1311) -> (unsigned 16bit integer=w1309:u16)
              }
            }
            n651 = case shown="False" w1277 {
              tunnel: [w1295 FALSE] -> w1288
              tunnel: w1287 -> [w1295 _]
              tunnel: [w1296 T4."Tracking" ("Next Main State")] -> w1286
              frame False {
                # "Check other Servo\nStay in Startup  State"
                n652 = local read "Image Lock - Left"() -> (w1294:bool)
                n653 = case shown="False" w1294 {
                  tunnel: [T4."Start Up Search" ("Next Main State") T4."Recovery Mode" ("Next Main State")] -> w1296
                  frame False {
                  }
                  frame True {
                  }
                }
              }
              frame True {
                # "Override Move Servo\nCommand bc an Angle Was Found\nduring this Step"
                # "Transition to Tracking State When\nImage Processing has Locked"
              }
            }
          }
          frame "Tracking" {
            w1342 = 0
            # "Frames Processed Count"
            # "Image Lock - L"
            # "Track Angle Valid"
            # "Tracking Angle"
            # "Tracking Timeout Count"
            # "Max ove delta"
            # "Move delta threshold"
            # "mount offset"
            # "Current Position"
            # "Move Respond"
            # "Trackin Timeout count"
            # "Move Servo"
            # "delta"
            # "GP"
            # "Reset Move Respond"
            # "New Tracking State"
            # "Delta Move Sum"
            # "Choose Next State"
            n654 = case shown="\"Track\", Default" w1354 {
              tunnel: w1368 -> [w1386 _]
              tunnel: w1367 -> [w1385 _]
              tunnel: w1366 -> [w1384 _]
              tunnel: w1365 -> [w1383 w1442]
              tunnel: [w1382 w1440] -> w1364
              tunnel: [w1381 w1448] -> w1363
              tunnel: [w1380 0] -> w1362
              tunnel: w1361 -> [w1379 _]
              tunnel: w1359 -> [w1378 w1432]
              tunnel: w1358 -> [w1377 w1435]
              tunnel: w1357 -> [w1376 w1437]
              tunnel: w1353 -> [_ w1447]
              tunnel: w1352 -> [_ w1446]
              tunnel: w1351 -> [_ w1445]
              tunnel: w1350 -> [_ w1444]
              tunnel: w1345 -> [_ w1443]
              tunnel: w1341 -> [_ w1441]
              tunnel: [TRUE w1438] -> w1347
              tunnel: [w1373 w1436] -> w1349
              tunnel: [w1371 w1434] -> w1346
              tunnel: [0 0] -> w1343
              frame "Track", Default {
                # "Reset"
                # "Tracking Timeout"
                # "Move Delta"
                # "Goal Position"
                # "Tracking Move"
                # "Move Servo"
                # "Only Consider Tracking Angle\n\nIF\n\nImage Locked        == T\nTrack Angle Flag   == T"
                n655 = And(x=w1378, y=w1377) -> (x .and. y?=w1370:bool)
                n656 = case shown="True" w1370 {
                  tunnel: w1386 -> [_ w1394]
                  tunnel: w1385 -> [_ w1411]
                  tunnel: w1384 -> [_ w1408]
                  tunnel: w1383 -> [w1389 w1398]
                  tunnel: [w1389 w1407] -> w1381
                  tunnel: [w1391 w1406] -> w1382
                  tunnel: [w1391 w1405] -> _
                  tunnel: [u16 0 w1404] -> w1380
                  tunnel: w1379 -> [_ w1400]
                  tunnel: w1376 -> [w1388 _]
                  tunnel: [w1387 0] -> w1373
                  frame False {
                    w1391 = FALSE
                    # "Increment timeout"
                    n657 = Increment(x=w1388) -> (x+1=w1387:i32)
                  }
                  frame True {
                    # "******"
                    # "Determine Direction of Move"
                    # "Convert Track Angle to UINT16"
                    # "1024/300"
                    # "Move to Tracking Angle \n\nif delta is greater than move servo threshold\nAND less than max move threshold"
                    n658 = Add(x=w1411, y=w1394) -> (x+y=w1414:sgl)
                    n659 = local read "Last Track Angle - R"() -> (w1393:sgl)
                    n660 = Add(x=w1414, y=sgl 60.0) -> (x+y=w1413:sgl)
                    n661 = Multiply(x=3.413333333333333, y=w1413) -> (x*y=w1392:dbl)
                    n662 = To Word Integer(number=w1398) -> (16bit integer=w1396:i16)
                    n663 = To Unsigned Word Integer(number=w1392) -> (unsigned 16bit integer=w1410:u16)
                    n664 = To Word Integer(number=w1392) -> (16bit integer=w1409:i16)
                    n665 = Subtract(x=w1392, y=w1393) -> ()  [unwired: 1 out]
                    n666 = Subtract(x=w1409, y=w1396) -> (x-y=w1399:i16)
                    n667 = Absolute Value(x=w1399) -> (abs(x)=w1395:i16)
                    n668 = Greater Or Equal?(x=w1395, y=w1408) -> (x >= y?=w1402:bool)
                    n669 = Less Or Equal?(x=w1395, y=w1400) -> (x <= y?=w1401:bool)
                    n670 = And(x=w1402, y=w1401) -> (x .and. y?=w1403:bool)
                    n671 = case shown="True" w1403 {
                      tunnel: w1410 -> [_ w1422]
                      tunnel: [w1417 w1422] -> w1407
                      tunnel: [w1418 w1428] -> w1406
                      tunnel: [w1418 w1428] -> w1405
                      tunnel: w1398 -> [w1417 _]
                      tunnel: w1395 -> [_ w1427]
                      tunnel: [u16 0 w1427] -> w1404
                      tunnel: w1394 -> [_ w1421]
                      frame False {
                        w1418 = FALSE
                        # "Don't Move"
                      }
                      frame True {
                        w1428 = TRUE
                        # "45 DEG MOUNT OFFSET"
                        # "1024/300"
                        # "Current Delta"
                        # "Use new Track Angle"
                        n672 = Divide(x=w1422, y=3.413333333333333) -> (x/y=w1424:dbl)
                        n673 = Negate(x=w1421) -> (-x=w1420:sgl)
                        n674 = Subtract(x=w1424, y=sgl 60.0) -> (x-y=w1426:dbl)
                        n675 = Add(x=w1426, y=w1420) -> (x+y=w1419:dbl)
                        n676 = local write "Last Track Angle - R"(w1419) -> ()
                      }
                    }
                  }
                }
                n677 = local read "Timeout to \nEnable Reactive Predict"() -> (w1374:u16)
                n678 = Less?(x=w1373, y=w1374) -> (x < y?=w1372:bool)
                n679 = case shown="True" w1372 {
                  tunnel: [enum16{"Track", "Reactive Predict", ""}."Reactive Predict" ("Initial Tracking State - Right") enum16{"Track", "Reactive Predict", ""}."Track" ("Initial Tracking State - Right")] -> w1371
                  frame False {
                  }
                  frame True {
                  }
                }
              }
              frame "Reactive Predict" {
                # "Choose New\nTracking State"
                n680 = Or(x=w1432, y=w1435) -> (x .or. y?=w1431:bool)
                n681 = case shown="False" w1431 {
                  tunnel: [w1461 w1514] -> w1448
                  tunnel: w1447 -> [w1460 _]
                  tunnel: w1446 -> [w1459 _]
                  tunnel: w1445 -> [w1458 _]
                  tunnel: w1444 -> [w1457 _]
                  tunnel: w1443 -> [w1456 _]
                  tunnel: w1441 -> [w1455 _]
                  tunnel: [w1454 FALSE] -> w1440
                  tunnel: [w1453 TRUE] -> w1438
                  tunnel: w1437 -> [w1452 _]
                  tunnel: [w1451 0] -> w1436
                  tunnel: [enum16{"Track", "Reactive Predict", ""}."Reactive Predict" ("Initial Tracking State - Right") enum16{"Track", "Reactive Predict", ""}."Track" ("Initial Tracking State - Right")] -> w1434
                  tunnel: w1442 -> [w1449 w1514]
                  frame False {
                    # "Stay in Reactive State"
                    # "Increment Track Timeout"
                    # "Move Respond Flag"
                    n682 = Increment(x=w1452) -> (x+1=w1451:i32)
                    n683 = case shown="True" w1456 {
                      tunnel: w1460 -> [_ w1476]
                      tunnel: w1459 -> [_ w1475]
                      tunnel: w1458 -> [_ w1474]
                      tunnel: w1457 -> [_ w1473]
                      tunnel: w1455 -> [_ w1470]
                      tunnel: [w1462 w1466] -> w1461
                      tunnel: [w1463 w1465] -> w1454
                      tunnel: [w1463 w1465] -> w1453
                      tunnel: w1449 -> [w1462 w1464]
                      frame False {
                        w1463 = FALSE
                        # "Reset Move Respond = F"
                        # "Move Servo = F"
                      }
                      frame True {
                        w1465 = TRUE
                        # "Position Lock"
                        # "Current Servo\nPosition"
                        # "Reset Move\nRespond = T"
                        # "Move Servo = T"
                        # "Apply Direction \nto Offset (delta sum)"
                        # "Check Last Known Position of Robot"
                        n684 = case shown="True" w1476 {
                          tunnel: w1475 -> [_ w1504]
                          tunnel: w1474 -> [_ w1479]
                          tunnel: w1473 -> [_ w1480]
                          tunnel: [sgl 1.0 ("y") w1478] -> w1472
                          frame False {
                            # "No Position Data Available"
                            # "Default is to move\nSame Direction as other\nServo"
                          }
                          frame True {
                            w1485 = sgl 1.0 ("y")
                            # "Use previous position/orientation to Guess Which Direction to Move Servo"
                            # "Choose Search Direction"
                            # "\"Perpendicular \nThreshold\""
                            # "If Orientation is\n ~Perpendicular -> Start Search\n in Opposite Direction of Other"
                            # "****add 90 until orientation angle is fixed"
                            # "Last Orientation"
                            # "Convert to Rad"
                            # "Avoid Divide by 0"
                            # "-1/m"
                            # "Calculate Normal Line to \nLast Robot Position\nfrom Center Beacon"
                            # "last Position \nCoordinates"
                            n685 = Unbundle(w1504) -> ("X"=w1484:sgl, "Y"=w1483:sgl)
                            n686 = Unbundle(w1480) -> ("X"=w1482:sgl, "Y"=w1481:sgl)
                            n687 = Subtract(x=w1483, y=w1481) -> (x-y=w1500:sgl)
                            n688 = Subtract(x=w1484, y=w1482) -> (x-y=w1498:sgl)
                            n689 = Equal To 0?(x=w1498) -> (x = 0?=w1499:bool)
                            n690 = case shown="False" w1499 {
                              tunnel: w1500 -> [w1507 _]
                              tunnel: w1498 -> [w1506 _]
                              tunnel: [w1505 1000000000000000.0] -> w1497
                              frame False {
                                n691 = Divide(x=w1507, y=w1506) -> (x/y=w1505:sgl)
                              }
                              frame True {
                              }
                            }
                            n692 = Equal To 0?(x=w1497) -> (x = 0?=w1502:bool)
                            n693 = case shown="False" w1502 {
                              tunnel: [w1509 1e-08] -> w1501
                              tunnel: w1497 -> [w1509 _]
                              frame False {
                              }
                              frame True {
                                # "Can't have infinit slope"
                              }
                            }
                            n694 = Divide(x=-1.0, y=w1501) -> (x/y=w1496:dbl)
                            n695 = Inverse Tangent(1:w1496) -> (0:w1494:dbl)
                            n696 = expression code="(x/pi)*180.0" "radians to degrees"(w1494) -> (w1495:dbl)
                            n697 = To Single Precision Float(number=w1495) -> (single precision float=w1492:sgl)
                            n698 = Add(x=w1479, y=sgl 90.0) -> (x+y=w1491:sgl)
                            n699 = Subtract(x=w1492, y=w1491) -> (x-y=w1490:sgl)
                            n700 = Absolute Value(x=w1490) -> (abs(x)=w1489:sgl)
                            n701 = Less Or Equal?(x=w1489, y=sgl 10.0) -> (x <= y?=w1487:bool)
                            n702 = Negate(x=w1485) -> (-x=w1486:sgl)
                            n703 = Select(t=w1486, s=w1487, f=w1485) -> (s? t:f=w1478:sgl)
                          }
                        }
                        n704 = To Word Integer(number=w1472) -> (16bit integer=w1471:i16)
                        n705 = Multiply(x=w1471, y=w1470) -> (x*y=w1469:i32)
                        n706 = To Word Integer(number=w1464) -> (16bit integer=w1468:i16)
                        n707 = Add(x=w1469, y=w1468) -> (x+y=w1467:i32)
                        n708 = To Unsigned Word Integer(number=w1467) -> (unsigned 16bit integer=w1466:u16)
                      }
                    }
                  }
                  frame True {
                    # "Either Current Angle Valid or Image Lock Acheived"
                    # "Go Directly to Track State"
                  }
                }
              }
            }
            n709 = local read "Tracking Timeout\nThreshold"() -> (w1355:i32)
            n710 = Less?(x=w1349, y=w1355) -> (x < y?=w1356:bool)
            n711 = case shown="True" w1356 {
              tunnel: [T4."Recovery Mode" ("Next Main State") T4."Tracking" ("Next Main State")] -> w1360
              frame False {
              }
              frame True {
              }
            }
          }
          frame "Recovery Mode" {
            w1524 = u16 0
            # "Recovery Search Move Count"
            # "***Compltetly resets as of R17, used to just reset to \"Max Recovery Count - 1\""
            # "Increment Recoveyr Mode Count"
            # "Frames Processed"
            # "Choose Next Main State"
            # "Reset recovery count"
            # "Recovery move\nCount"
            # "Recovery Search\nAttempt count"
            # "Move Servo = T"
            # "delta move sum"
            # "Robot Position Valid"
            n712 = local read "Image Lock - Left"() -> (w1528:bool)
            n713 = case shown="\"Generic Sweep\"" w1521 {
              tunnel: w1550 -> [_ _]
              tunnel: w1549 -> [_ _]
              tunnel: w1548 -> [_ _]
              tunnel: w1547 -> [_ _]
              tunnel: w1546 -> [_ _]
              tunnel: w1545 -> [_ _]
              tunnel: w1544 -> [w1578 w1664]
              tunnel: [w1570 w1662] -> w1543
              tunnel: [w1567 w1656] -> w1542
              tunnel: [FALSE FALSE] -> w1522
              tunnel: [w1572 w1654] -> w1541
              tunnel: w1538 -> [w1576 _]
              tunnel: w1540 -> [w1579 _]
              tunnel: w1539 -> [w1577 w1659]
              tunnel: [w1569 w1653] -> w1536
              tunnel: [w1568 w1653] -> w1537
              tunnel: w1528 -> [w1566 _]
              tunnel: [w1557 w1663] -> w1535
              tunnel: w1534 -> [w1555 w1651]
              tunnel: w1533 -> [w1560 w1660]
              tunnel: w1532 -> [w1556 w1658]
              tunnel: w1518 -> [_ _]
              tunnel: w1520 -> [_ _]
              tunnel: [FALSE w1655] -> w1530
              tunnel: w1527 -> [w1564 _]
              tunnel: w1526 -> [w1563 _]
              tunnel: [w1560 w1652] -> w1525
              tunnel: w1518 -> [_ w1649]
              frame "Recovery Search" {
                # "Wait for 2 Images to be Processed\nBefore Going to Next Step"
                # "Choose Next Reovery State"
                # "Recovery Search \nAttempt Count"
                # "Move Servo"
                # "Goal Position"
                # "Recovery Search\nmove Count"
                # "Attempt Recovery Search if Other Servo has Valid Angle"
                n714 = local read "Last Track Angle - L"() -> (w1559:sgl)
                n715 = Greater Or Equal?(x=w1555, y=w1556) -> (x >= y?=w1558:bool)
                n716 = case shown="False" w1558 {
                  tunnel: w1579 -> [_ w1599]
                  tunnel: [w1584 w1598] -> w1568
                  tunnel: w1578 -> [w1587 w1597]
                  tunnel: w1577 -> [_ w1596]
                  tunnel: [w1585 w1595] -> w1569
                  tunnel: [w1587 w1594] -> w1570
                  tunnel: [FALSE w1593] -> w1567
                  tunnel: w1564 -> [w1585 w1592]
                  tunnel: w1563 -> [w1584 w1591]
                  tunnel: w1566 -> [_ w1590]
                  tunnel: w1559 -> [_ w1589]
                  tunnel: [w1582 0 ("Frames Processed\nCount - in")] -> w1557
                  tunnel: w1555 -> [w1583 _]
                  frame False {
                    # "Increment Frames Processed"
                    # "WAIT"
                    n717 = Increment(x=w1583) -> (x+1=w1582:i32)
                  }
                  frame True {
                    n718 = case shown="False" w1590 {
                      tunnel: w1589 -> [_ w1612]
                      tunnel: w1592 -> [w1600 w1608]
                      tunnel: w1599 -> [_ w1613]
                      tunnel: [w1603 w1611] -> w1594
                      tunnel: [w1601 w1610] -> w1598
                      tunnel: w1591 -> [w1601 w1609]
                      tunnel: w1597 -> [w1603 w1607]
                      tunnel: w1596 -> [_ w1606]
                      tunnel: [FALSE TRUE] -> w1593
                      tunnel: [w1600 w1604] -> w1595
                      frame False {
                        # "Don't Move bc Other Servo Doesn't Have Image Lock"
                      }
                      frame True {
                        # "Move Servo = T"
                        n719 = Greater Than 0?(x=w1608) -> (x > 0?=w1614:bool)
                        n720 = case shown="False" w1614 {
                          tunnel: w1613 -> [w1623 _]
                          tunnel: w1612 -> [w1618 _]
                          tunnel: [w1616 w1634] -> w1611
                          tunnel: [w1621 w1639] -> w1610
                          tunnel: w1609 -> [w1622 w1639]
                          tunnel: w1608 -> [w1620 w1636]
                          tunnel: [w1619 w1638] -> w1604
                          tunnel: w1607 -> [_ w1635]
                          tunnel: w1606 -> [_ w1632]
                          frame False {
                            # "************************"
                            # "Increment move count to transition\nto Pan mode"
                            # "Increment Recovery Search Attempt Count"
                            # "1024/300"
                            # "Move Parallel to Other Servo"
                            n721 = Increment(x=w1622) -> (x+1=w1621:i32)
                            n722 = Add(x=w1618, y=w1623) -> (x+y=w1629:sgl)
                            n723 = Add(x=w1629, y=sgl 60.0) -> (x+y=w1628:sgl)
                            n724 = Multiply(x=3.413333333333333, y=w1628) -> (x*y=w1626:dbl)
                            n725 = Add(x=0.5, y=w1626) -> (x+y=w1624:dbl)
                            n726 = To Unsigned Word Integer(number=w1624) -> (unsigned 16bit integer=w1617:u16)
                            n727 = Increment(x=w1620) -> (x+1=w1619:i32)
                            n728 = local read "Recovery Parallel\nSearch Offset"() -> (w1615:u16)
                            n729 = Add(x=w1617, y=w1615) -> (x+y=w1616:u16)
                          }
                          frame True {
                            # "Apply Direction"
                            # "Step SIze"
                            # "Current Position"
                            # "Attempt to Pan in Steps Towards other Servo"
                            # "Could be same or function of \nregular search step size"
                            # "Max # of Pan\nMoves"
                            # "Pan Towards Other Servo"
                            n730 = local read "Max # Pan Moves"() -> (w1631:u16)
                            n731 = Greater Or Equal?(x=w1636, y=w1631) -> (x >= y?=w1637:bool)
                            n732 = case shown="False" w1637 {
                              tunnel: w1636 -> [w1647 _]
                              tunnel: [w1646 u16 0] -> w1638
                              frame False {
                                # "Increment Pan Count"
                                n733 = Increment(x=w1647) -> (x+1=w1646:i32)
                              }
                              frame True {
                                # "Reset move count"
                              }
                            }
                            n734 = local read "Recovery Search\nDirection - R"() -> (w1633:bool)
                            n735 = case shown="True" w1633 {
                              tunnel: w1635 -> [w1641 w1645]
                              tunnel: w1632 -> [w1642 w1644]
                              tunnel: [w1640 w1643] -> w1634
                              frame False {
                                # "CCW"
                                n736 = Add(x=w1641, y=w1642) -> (x+y=w1640:u16)
                              }
                              frame True {
                                # "CW"
                                n737 = Subtract(x=w1645, y=w1644) -> (x-y=w1643:u16)
                              }
                            }
                          }
                        }
                      }
                    }
                  }
                }
                n738 = local read "Max Recovery Count\n(Recovery Search)"() -> (w1561:u16)
                n739 = local read "Max Recovery\nSearch Attempts"() -> (w1562:u16)
                n740 = Less Or Equal?(x=w1568, y=w1562) -> (x <= y?=w1574:bool)
                n741 = Less Or Equal?(x=w1576, y=w1561) -> (x <= y?=w1575:bool)
                n742 = And(x=w1574, y=w1575) -> (x .and. y?=w1573:bool)
                n743 = case shown="True" w1573 {
                  tunnel: [enum16{"Generic Sweep", "Recovery Search"}."Generic Sweep" enum16{"Generic Sweep", "Recovery Search"}."Recovery Search"] -> w1572
                  frame False {
                  }
                  frame True {
                  }
                }
              }
              frame "Generic Sweep" {
                w1653 = u16 0
                # "Image Locked?"
                # "Choose Next Recovery State"
                # "Wait for 2 Images to be Processed\nBefore Going to Next Step"
                # "New Goal Position"
                # "Move Servo"
                # "Frames Processed Count"
                n744 = Greater Or Equal?(x=w1651, y=w1658) -> (x >= y?=w1665:bool)
                n745 = case shown="True" w1665 {
                  tunnel: w1664 -> [w1681 w1697]
                  tunnel: w1659 -> [_ w1695]
                  tunnel: w1660 -> [w1680 w1694]
                  tunnel: [w1681 w1687] -> w1662
                  tunnel: [w1679 0] -> w1663
                  tunnel: [FALSE TRUE] -> w1657
                  tunnel: w1651 -> [w1682 _]
                  tunnel: [w1680 w1688] -> w1652
                  frame False {
                    # "Increment Frames Processed"
                    n746 = Increment(x=w1682) -> (x+1=w1679:i32)
                  }
                  frame True {
                    # "Reset Frames\nProcessed Count"
                    # "SWEEP SEARCH - Startup"
                    # "Multiple New Step\nby Step SIze"
                    # "F = CCW\nT = CW"
                    # "Last Direction"
                    # "Min Step"
                    # "add 10 in case\nactual position\nis lower than GP"
                    # "Set New Step #"
                    # "Choose Direction"
                    # "Nearest step"
                    # "Adjust Actual Posiiton\n to pre-determiend steps"
                    # "Move Servo 1 \"Step\" to\nSearch"
                    n747 = Subtract(x=w1697, y=u16 524) -> (x-y=w1685:u16)
                    n748 = Add(x=5, y=w1685) -> (x+y=w1703:i32)
                    n749 = Quotient & Remainder(x=w1703, y=w1695) -> (floor(x/y)=w1701:i32)  [unwired: 1 out]
                    n750 = To Byte Integer(number=w1701) -> (8bit integer=w1692:i8)
                    n751 = Less?(x=w1692, y=1) -> (x < y?=w1698:bool)
                    n752 = case shown="False" w1698 {
                      tunnel: w1692 -> [w1714 w1722]
                      tunnel: [w1716 FALSE] -> w1688
                      tunnel: [w1715 w1722] -> w1700
                      tunnel: w1694 -> [w1713 _]
                      tunnel: w1695 -> [w1711 _]
                      frame False {
                        # "Max Step"
                        # "# of steps\nminus 1"
                        n753 = Divide(x=300, y=w1711) -> (x/y=w1708:dbl)
                        n754 = To Unsigned Byte Integer(number=w1708) -> (unsigned 8bit integer=w1709:u8)
                        n755 = Greater Or Equal?(x=w1714, y=w1709) -> (x >= y?=w1710:bool)
                        n756 = case shown="True" w1710 {
                          tunnel: [w1717 TRUE] -> w1716
                          tunnel: [w1718 w1719] -> w1715
                          tunnel: w1714 -> [w1718 w1719]
                          tunnel: w1713 -> [w1717 _]
                          frame False {
                            # "No Need to\nChange Direction"
                          }
                          frame True {
                            # "T"
                            # "Move CW"
                          }
                        }
                      }
                      frame True {
                        # "F"
                        # "Move CCW"
                      }
                    }
                    n757 = case shown="True" w1688 {
                      tunnel: w1700 -> [w1705 w1706]
                      tunnel: [w1704 w1707] -> w1696
                      frame False {
                        # "CCW\n+1"
                        n758 = Increment(x=w1705) -> (x+1=w1704:i8)
                      }
                      frame True {
                        # "CW\n-1"
                        n759 = Decrement(x=w1706) -> (x-1=w1707:i8)
                      }
                    }
                    n760 = Multiply(x=w1696, y=w1695) -> (x*y=w1693:u16)
                    n761 = To Unsigned Word Integer(number=w1693) -> (unsigned 16bit integer=w1691:u16)
                    n762 = Add(x=w1691, y=u16 524) -> (x+y=w1687:u16)
                  }
                }
                n763 = local read "Image Lock - Left"() -> (w1650:bool)
                n764 = case shown="False" w1649 {
                  tunnel: [w1668 w1678] -> w1656
                  tunnel: w1657 -> [w1669 _]
                  tunnel: [w1670 enum16{"Generic Sweep", "Recovery Search"}."Generic Sweep"] -> w1654
                  tunnel: [w1667 w1678] -> w1655
                  tunnel: w1650 -> [w1666 _]
                  frame False {
                    # "Is other servo tracking?"
                    n765 = case shown="True" w1666 {
                      tunnel: [enum16{"Generic Sweep", "Recovery Search"}."Generic Sweep" enum16{"Generic Sweep", "Recovery Search"}."Recovery Search"] -> w1670
                      tunnel: w1669 -> [w1673 _]
                      tunnel: [w1673 FALSE] -> w1668
                      tunnel: [FALSE TRUE] -> w1667
                      frame False {
                        # "Stay in Sweep"
                      }
                      frame True {
                        # "G o to Recovery Search  State"
                      }
                    }
                  }
                  frame True {
                    w1678 = FALSE
                    # "Override Move Servo\nCommand bc an Angle Was Found\nduring this Step"
                    # "Stay In Sweep\nLet Main State Machine transition\ninto Tracking"
                  }
                }
              }
            }
            n766 = Increment(x=w1538) -> (x+1=w1519:i32)
            n767 = case shown="False" w1530 {
              tunnel: w1519 -> [w1553 _]
              tunnel: [w1553 0] -> w1531
              frame False {
              }
              frame True {
              }
            }
            n768 = case shown="False" w1518 {
              tunnel: [T4."Recovery Mode" ("Next Main State") T4."Tracking" ("Next Main State")] -> w1529
              frame False {
              }
              frame True {
              }
            }
          }
        }
        "Current Move Delta - R" <- w1249
        n769 = Less?(x=w1276, y=w1275) -> (x < y?=w1274:bool)
        n770 = local write "New Data  Flag\nRight Servo"(FALSE) -> ()
        n771 = Select(t=w1275, s=w1274, f=w1276) -> (s? t:f=w1271:u16)
        n772 = Greater?(x=w1271, y=w1272) -> (0:w1273:bool)
        n773 = Select(t=w1272, s=w1273, f=w1271) -> (s? t:f=w1270:u16)
      }
    }
    "Next Main State - Right" <- w1115
    "Next Tracking State - Right" <- w1121
    "Next Recovery State - Right" <- w1120
    n774 = flat-sequence {
      tunnel: w1206 -> [w2231]
      tunnel: w1116 -> [w2230]
      tunnel: w1207 -> [w2233]
      tunnel: w1117 -> [w2232]
      tunnel: [w2231] -> w1220
      tunnel: [w2230] -> w1219
      tunnel: w1220 -> [w2239]
      tunnel: [w2238] -> w1215
      tunnel: [w2237] -> w1216
      tunnel: w1219 -> [w2236]
      frame #0 {
        # "Only Update GP if Moving Servo"
        n775 = case shown="True" w2231 {
          tunnel: w2233 -> [_ w2235]
          frame False {
          }
          frame True {
            # "Update Goal Position"
            n776 = local write "Servo Goal Position\n - Left"(w2235) -> ()
          }
        }
        n777 = case shown="True" w2230 {
          tunnel: w2232 -> [_ w2234]
          frame False {
          }
          frame True {
            # "New Direction"
            # "Update Goal Position"
            # "Update Direction"
            n778 = local write "Servo Goal Position\n - Right"(w2234) -> ()
          }
        }
      }
      frame #1 {
        # "Allow Comm Process to Take Down the Flag\nOnly Raise if not already in motion"
        n779 = local read "Servo Moving - R"() -> (w2244:bool)
        n780 = local read "Servo Moving - L"() -> (w2241:bool)
        n781 = local read "Move Servo - L"() -> (w2240:bool)
        n782 = local read "Move Servo - R"() -> (w2247:bool)
        n783 = Not(x=w2244) -> (.not. x?=w2246:bool)
        n784 = Not(x=w2241) -> (.not. x?=w2243:bool)
        n785 = And(x=w2236, y=w2246) -> (x .and. y?=w2245:bool)
        n786 = And(x=w2239, y=w2243) -> (x .and. y?=w2242:bool)
        n787 = case shown="True" w2245 {
          selector: w2245 -> [_ w2249]
          tunnel: [w2248 w2249] -> w2237
          tunnel: w2247 -> [w2248 _]
          frame False {
          }
          frame True {
          }
        }
        n788 = case shown="False" w2242 {
          selector: w2242 -> [_ w2251]
          tunnel: [w2250 w2251] -> w2238
          tunnel: w2240 -> [w2250 _]
          frame False {
          }
          frame True {
          }
        }
        n789 = local write "Move Servo - R"(w2237) -> ()
        n790 = local write "Move Servo - L"(w2238) -> ()
      }
    }
    n791 = local read "Current Tracking State - Right 2"() -> (w1160:enum16{"Track", "Reactive Predict", ""})
    n792 = local read "Current Tracking State - Left"() -> (w1162:enum16{"Track", "Reactive Predict", ""})
    n793 = local read "Current Main State - Left"() -> (w1186:T4)
    n794 = local read "Current Main State - Right"() -> (w1161:T4)
    n795 = Equal?(x=w1161, y=w1185) -> (x = y?=w1155:bool)
    n796 = Equal?(x=w1160, y=w1159) -> (x = y?=w1154:bool)
    n797 = Equal?(x=w1186, y=w1185) -> (x = y?=w1157:bool)
    n798 = Equal?(x=w1162, y=w1159) -> (x = y?=w1158:bool)
    n799 = And(x=w1155, y=w1154) -> (x .and. y?=w1153:bool)
    n800 = And(x=w1157, y=w1158) -> (x .and. y?=w1156:bool)
    n801 = And(x=w1156, y=w1215) -> (x .and. y?=w1211:bool)
    n802 = And(x=w1216, y=w1153) -> (x .and. y?=w1212:bool)
    n803 = And(x=w1156, y=w1153) -> (x .and. y?=w1210:bool)
    n804 = Exclusive Or(1:w1212, 2:w1211) -> (0:w1209:bool)
    n805 = case shown="True" w1209 {
      tunnel: [w2262 w2283] -> w1217
      tunnel: [w2263 w2282] -> w1213
      tunnel: w1118 -> [_ w2286]
      tunnel: w1176 -> [w2260 w2287]
      tunnel: w1129 -> [w2258 w2285]
      tunnel: [w2261 w2273] -> w1214
      tunnel: [w2259 w2272] -> w1218
      tunnel: w1184 -> [_ w2284]
      tunnel: w1210 -> [w2257 _]
      tunnel: w1211 -> [_ w2283]
      tunnel: w1212 -> [_ w2282]
      frame False {
        n806 = case shown="False" w2257 {
          tunnel: [w2267 w2269] -> w2263
          tunnel: [w2266 w2269] -> w2262
          tunnel: [w2265 w2268] -> w2261
          tunnel: w2260 -> [w2265 _]
          tunnel: [w2264 w2268] -> w2259
          tunnel: w2258 -> [w2264 _]
          frame False {
            # "No Movement\nRetain All Values"
            n807 = local read "Move Respond - L"() -> (w2267:bool)
            n808 = local read "Move Respond - R"() -> (w2266:bool)
          }
          frame True {
            w2268 = i16 0
            w2269 = FALSE
            # "Reset Delta Move sum\nfor both"
            # "F"
            # "Both Moved,\nMake Flags False"
          }
        }
      }
      frame True {
        w2279 = 200 ("y")
        w2270 = -200 ("y")
        # "Add/Clear Sum for \nServo That didn't move"
        # "Update Moving Servo's  Delta Position"
        # "if one Servo Moves, other should \nmove too eventually,\nUsed in Search Process"
        # "Only 1 Servo is Moving Due to Tracking --> Update delta move sum"
        n809 = case shown="True" w2282 {
          tunnel: w2287 -> [_ w2295]
          tunnel: w2286 -> [_ w2294]
          tunnel: [i16 0 w2293] -> w2280
          frame False {
          }
          frame True {
            n810 = Add(x=w2295, y=w2294) -> (x+y=w2293:i32)
          }
        }
        n811 = case shown="True" w2283 {
          tunnel: w2285 -> [_ w2291]
          tunnel: w2284 -> [_ w2290]
          tunnel: [i16 0 w2289] -> w2277
          frame False {
          }
          frame True {
            n812 = Add(x=w2291, y=w2290) -> (x+y=w2289:i32)
          }
        }
        n813 = Greater?(x=w2280, y=w2279) -> (0:w2281:bool)
        n814 = Greater?(x=w2277, y=w2279) -> (0:w2278:bool)
        n815 = Select(t=w2279, s=w2278, f=w2277) -> (s? t:f=w2274:i32)
        n816 = Select(t=w2279, s=w2281, f=w2280) -> (s? t:f=w2275:i32)
        n817 = Greater?(x=w2275, y=w2270) -> (0:w2271:bool)
        n818 = Greater?(x=w2274, y=w2270) -> (0:w2276:bool)
        n819 = Select(t=w2274, s=w2276, f=w2270) -> (s? t:f=w2272:i32)
        n820 = Select(t=w2275, s=w2271, f=w2270) -> (s? t:f=w2273:i32)
      }
    }
    n821 = case shown="True" w1122 {
      selector: w1122 -> [_ w2229]
      tunnel: [w2226 w2228] -> w1171
      tunnel: [w2225 i16 0] -> w1172
      tunnel: w1217 -> [w2226 _]
      tunnel: w1218 -> [w2225 _]
      frame False {
      }
      frame True {
        n822 = Not(x=w2229) -> (.not. x?=w2228:bool)
      }
    }
    "Move Respond - R" <- w1171
    "deltaMoveServo\n- R" <- w1172
    n823 = case shown="False" w1182 {
      selector: w1182 -> [_ w2256]
      tunnel: [w2253 w2255] -> w1174
      tunnel: [w2252 i16 0] -> w1177
      tunnel: w1213 -> [w2253 _]
      tunnel: w1214 -> [w2252 _]
      frame False {
      }
      frame True {
        n824 = Not(x=w2256) -> (.not. x?=w2255:bool)
      }
    }
    "Move Respond - L" <- w1174
    "deltaMoveServo\n- L" <- w1177
    "Current Main State - Left" <- w1205
    "Frames Processed\nCount - in -L" <- w1197
    "Recovery Mode Count - in Left" <- w1192
    "Recovery Search\nmove Count - in - L" <- w1191
    "Recovery Search\nAttempt Count - in - L" <- w1190
    "Current Main State - Right" <- w1152
    "Frames Processed\nCount - in Right" <- w1135
    "Recovery Search\nmove Count - Right" <- w1137
    "Recovery Search\nAttempt Count - Right" <- w1136
    "Recovery Mode Count in Right" <- w1128
    "Tracking Timeout\nCount - L" <- w1169
    "Tracking Timeout\nCount - R" <- w1144
    "Current Tracking State - Left" <- w1168
    "Current Tracking State - Right 2" <- w1150
    "Current Recovery State - Right" <- w1151
    "Current Recovery State -L" <- w1165
  }
